vi "PLC_comm.vi"() -> ()   [LabVIEW 2017]
uses:
  <vilib>/addons/database/NI_Database_API.lvlib
  Global/DATA LOG.vi
  Global/Global 1.vi
  <vilib>/DATA AHEAD/SP7/typedefs/PLC Type.ctl
  <vilib>/DATA AHEAD/SP7/SP7.lvlib
  <vilib>/DATA AHEAD/SP7/functions/read/read String.vi
  <vilib>/DATA AHEAD/SP7/functions/write/write Dint array.vi
  <vilib>/DATA AHEAD/SP7/functions/read/read Dint array.vi
  <vilib>/Utility/error.llb/DialogType.ctl
  <vilib>/DATA AHEAD/SP7/functions/read/read real array.vi
  <vilib>/DATA AHEAD/SP7/functions/write/writeString.vi
  84f8396c-11e3-4f6e-927f-d6cb52f8486f.vi
  edb3f7e3-deb4-4efd-b63a-82a20ab466dd.vi
  737c4a97-5810-4f09-bfe1-7e6a970161fd.vi
  98a23aa7-5d76-4ce5-89a1-7ffa2d6e86d6.vi
  065602cd-1ec6-46a4-aff5-3b00a0c776c3.vi
  <vilib>/DATA AHEAD/SP7/typedefs/S7 Connection.ctl
  Control/PLC_Comm_State.ctl
  <vilib>/addons/database/Connection.llb/DB Tools Open Connec (String).vi
  f53d9a16-31ea-4c58-9ec6-4ab155e6634a.vi
  f2e501b8-8033-40fd-b99e-90a89dd29cf5.vi
  a17ecfbb-e8aa-4e6f-9723-a9b27e8c0652.vi
  3deaaee4-0312-4209-8b7c-ccc637c44985.vi
  adc7d8b8-ea76-443b-992e-07ffa118bf03.vi
  cf2a4f70-d875-4391-b4be-4b1ea527ec99.vi
  b767813d-b0bc-4642-82b7-59e8eeaf8486.vi
panel:
  out "error out 4":errorcluster
  out "error out 3":errorcluster
  out "IP1 8":string
  out "PLC 8":bool
  out "IP1 7":string
  out "PLC 7":bool
  out "IP1 6":string
  out "PLC 6":bool
  out "IP1 5":string
  out "PLC 5":bool
  out "PLC 4":bool
  out "PLC 3":bool
  out "PLC 1":bool
  out "IP1 4":string
  out "IP1 3":string
  out "IP1 2":string
  out "IP1":string
  in  "stop":bool
  out "error out":errorcluster
  in  "error in (no error)":errorcluster
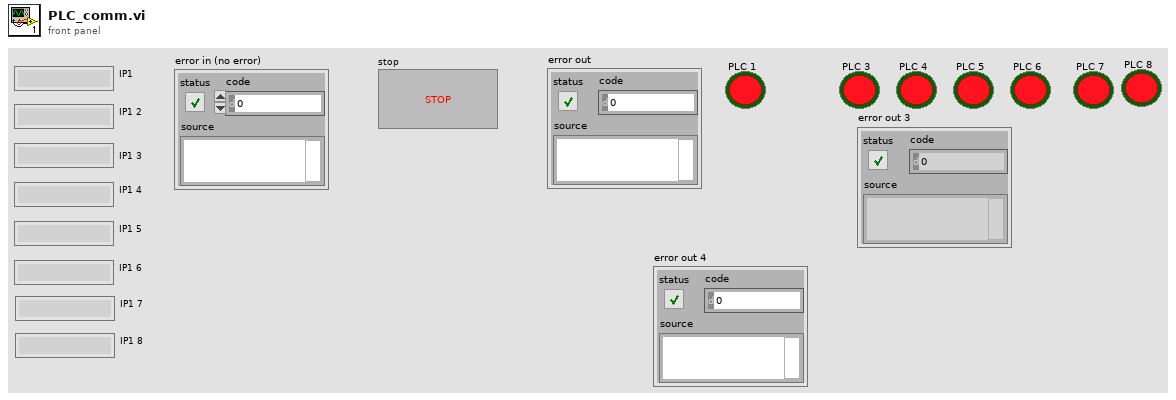
[diagram p1: front panel]
types:
  T1 = typedef "PLC_Comm_State.ctl" = enum16{"Int", "Connect", "Write", "Write2", "Write3", "Read", "Read2", "Read3", "Error", "Disconnect"}
  T2 = typedef "DialogType.ctl" = u16
  T3 = typedef "NI_Database_API.lvlib/Conn ObjectReference.ctl" = refnum<k1>
  T4 = typedef "SP7.lvlib/PLC Type.ctl" = enum16{"S7 200", "S7 300/400", "S7 1200", "S7 1500", "LOGO!8"}
  T5 = typedef "SP7.lvlib/S7 Connection.ctl" = cluster{"TCP Connection Ref":refnum<k5>, "IP address":string, "timeout ms":i32, "Connected?":bool, "PLC Type":T4, "Rack S7 400":u8, "Slot S7 400":u8, "PDU Size":u16, "connection semaphore":T6}
  T6 = typedef "Semaphore RefNum" = refnum<k1>
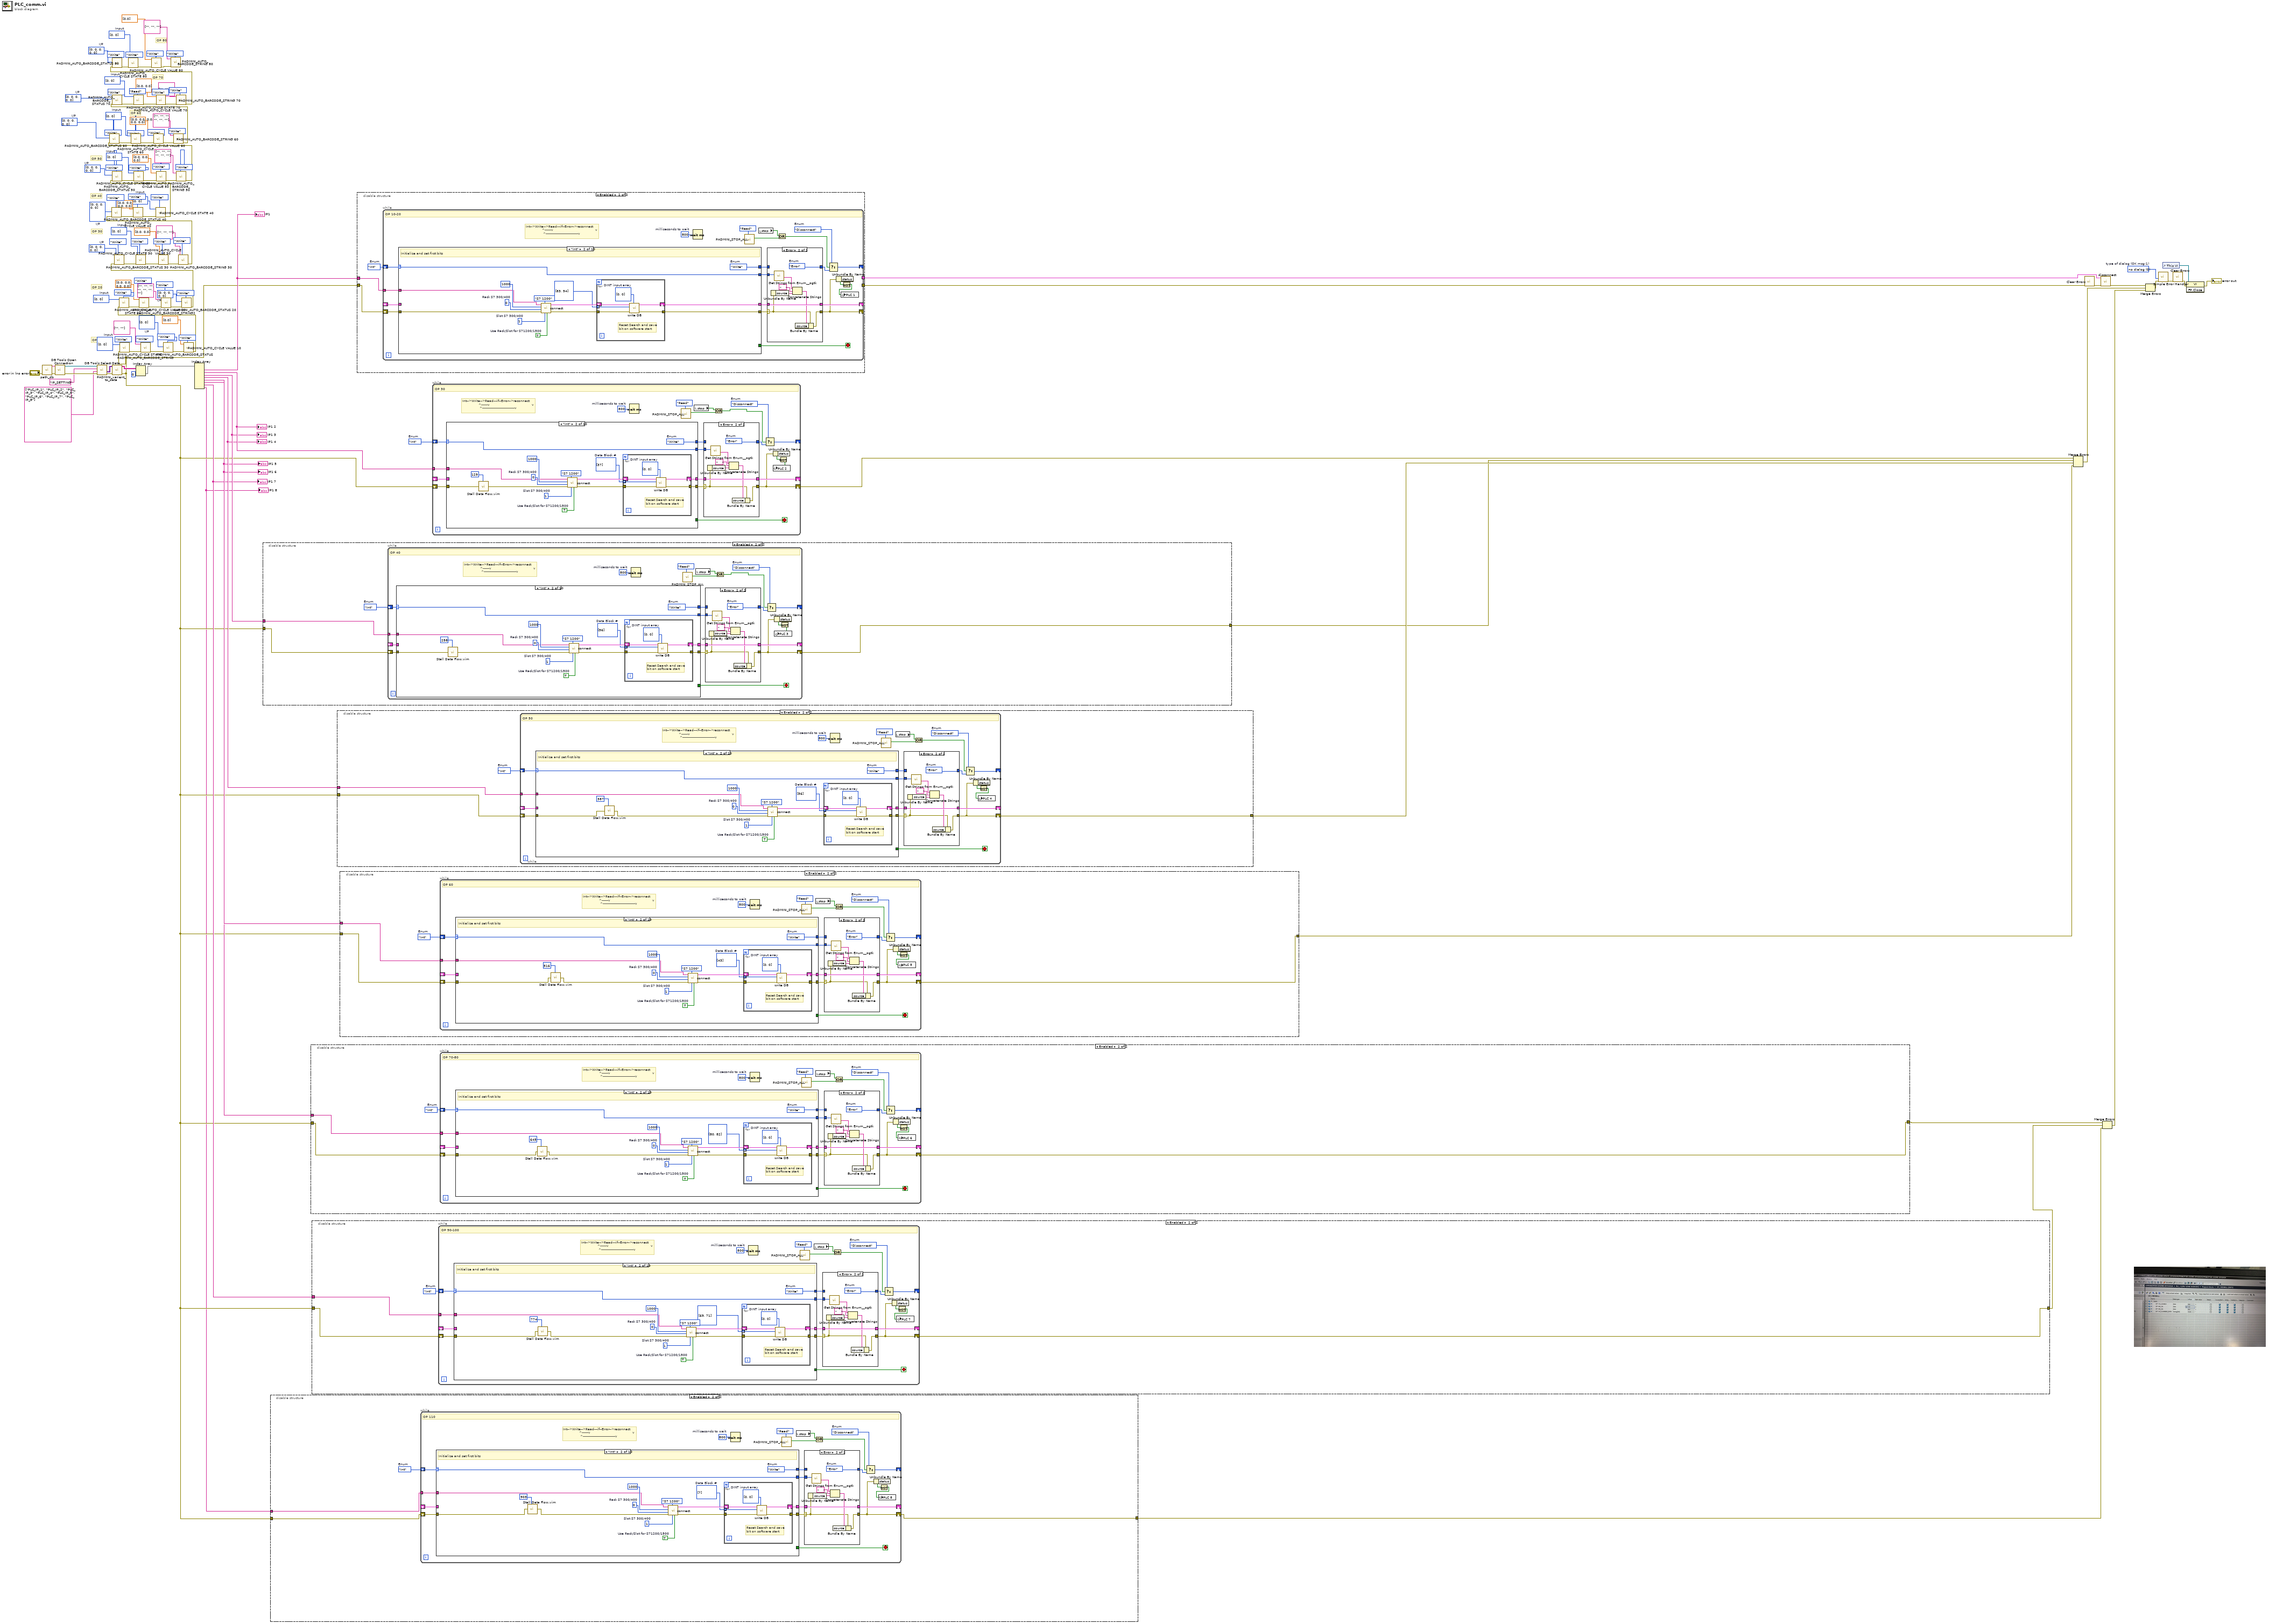
[diagram p0: block diagram]
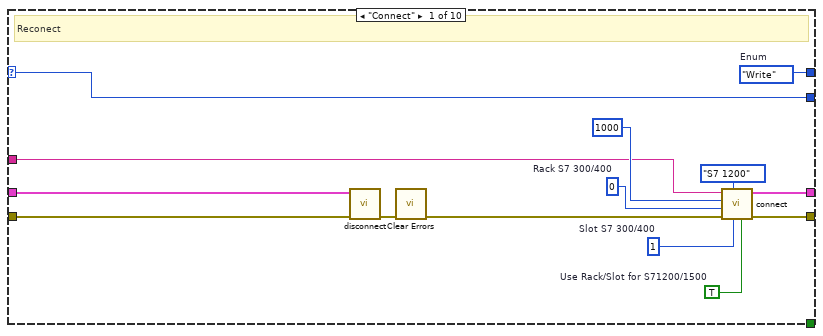
[diagram p3: hidden frame]
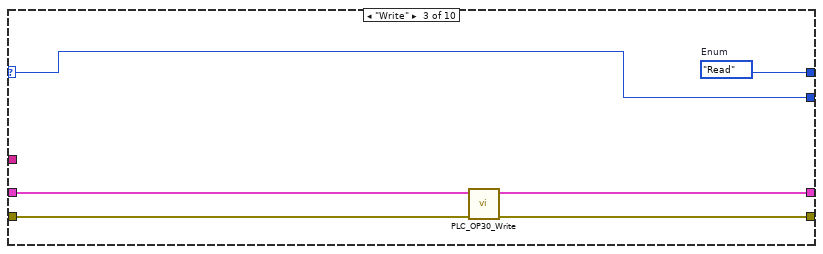
[diagram p4: hidden frame]
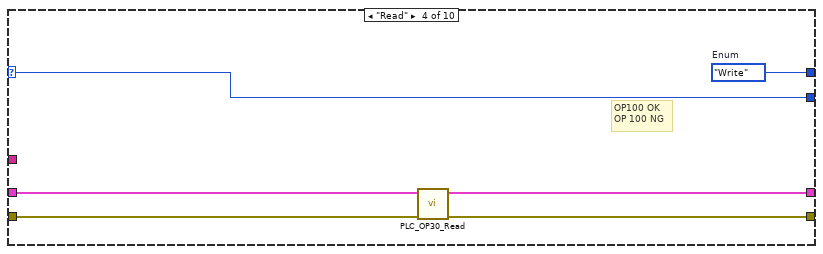
[diagram p5: hidden frame]
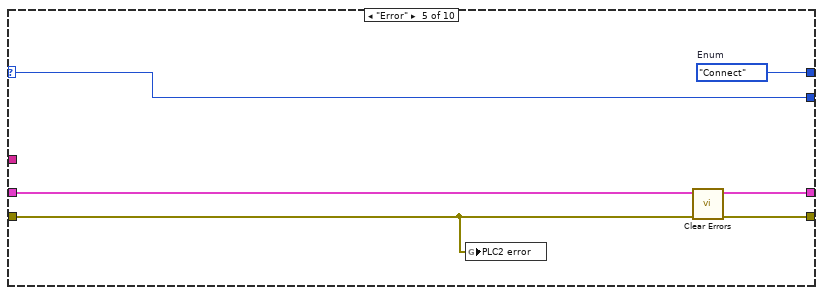
[diagram p6: hidden frame]
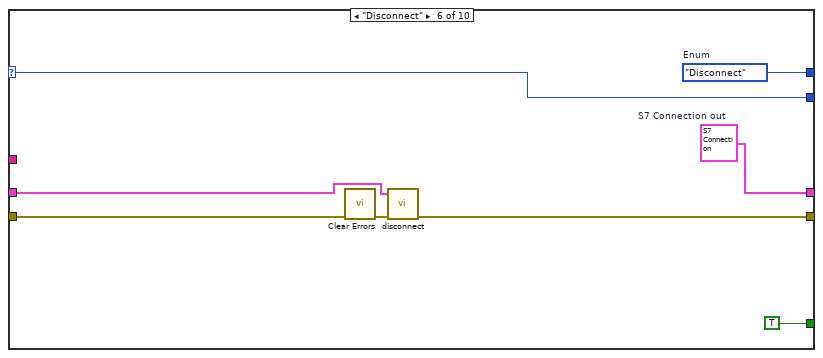
[diagram p7: hidden frame]
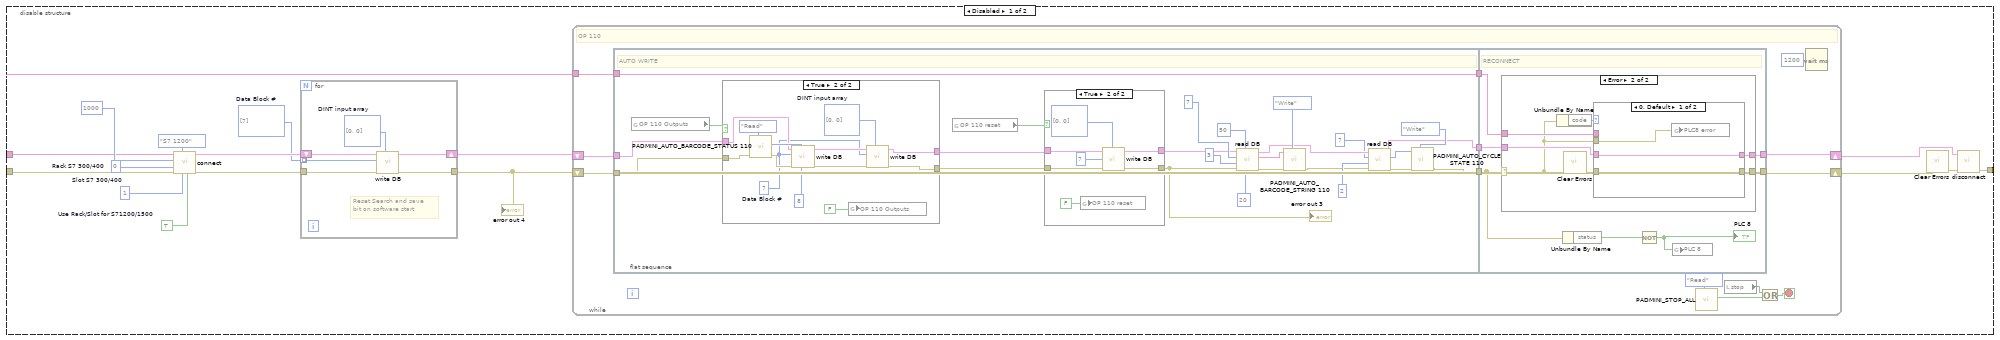
[diagram p12: hidden frame]
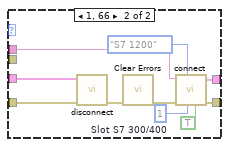
[diagram p16: hidden frame]
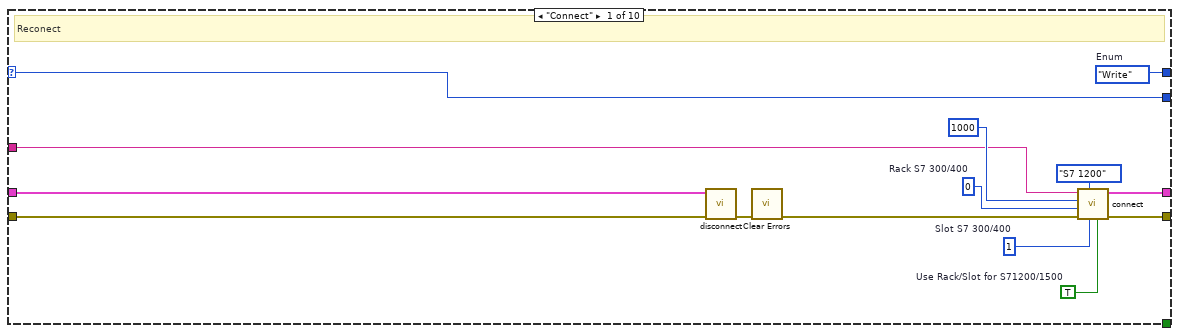
[diagram p18: hidden frame]
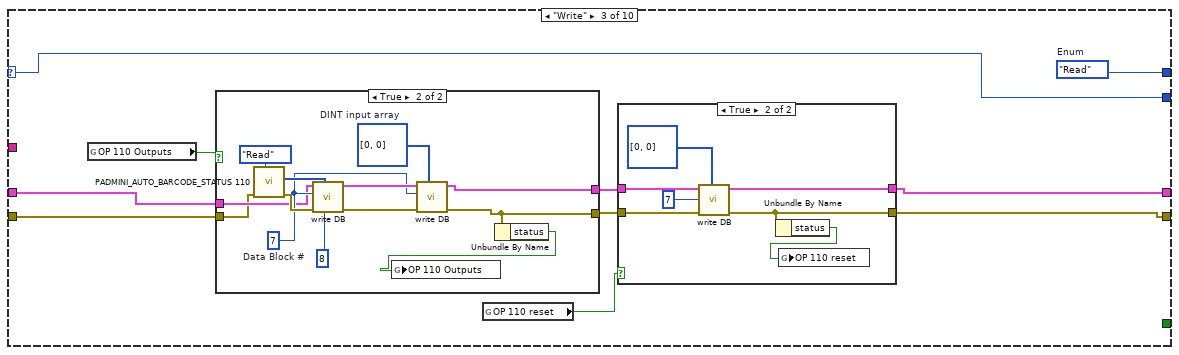
[diagram p19: hidden frame]
diagram:
  w1 = PLC_Comm_State."Int"  # Enum
  w10 = T2 0 items=["no dialog", "OK message", "continue or stop message", "OK message + warnings", "continue/stop + warnings"]  # type of dialog (OK msg:1)
  w12 = i32[] [0, 0, 0, 0, 0]  # I/P
  w13 = i32[] [0, 0]  # Input
  w15 = i32[] [0, 0]  # Input
  w16 = i32[] [0, 0]  # Input
  w18 = i32[] [0, 0]  # Input
  w14 = i32[] [0, 0, 0, 0, 0]  # I/P
  w17 = i32[] [0, 0, 0, 0, 0]  # I/P
  w19 = i32[] [0, 0, 0, 0, 0]  # I/P
  w20 = i32[] [0, 0, 0, 0, 0]  # I/P
  w21 = i32[] [0, 0]  # Input
  w22 = i32[] [0, 0]  # Input
  w23 = i32[] [0, 0, 0, 0, 0]  # I/P
  w24 = i32[] [0, 0, 0, 0, 0]  # I/P
  w25 = i32[] [0, 0]  # Input
  w26 = i32[] [0, 0]  # I/P
  w27 = i32[] [0, 0]  # Input
  # "OP 80"
  # "OP 70"
  # "OP 60"
  # "OP 50"
  # "OP 40"
  # "OP 30"
  # "OP 20"
  # "OP 10"
  n1 = call "path_db.vi"("error in"="error in (no error)") -> ("error out"=w128:errorcluster, "resulting string"=w133:string)  [unwired: 9 in]
  n2 = call-poly <vilib>:"DB Tools Open Connection.vi"("error in (no error)"=w128, "connection information"=w133) -> ("error out"=w132:errorcluster, "connection reference"=w131:T3)  [unwired: 6 in]
  n3 = call <vilib>:"DB Tools Select Data.vi"("error in (no error)"=w132, "columns"=string[] ["PLC_IP_1", "PLC_IP_2", "PLC_IP_3", "PLC_IP_4", "PLC_IP_5", "PLC_IP_6", "PLC_IP_7", "PLC_IP_8"], "table"="IP_SETTING", "connection reference"=w131) -> ("error out"=w130:errorcluster, "data"=w129:variant[][])  [unwired: 2 in, 1 out]
  n4 = call "PADMINI_varient_to_data.vi"("error in (no error)"=w130, "data"=w129) -> ("error out"=w9:errorcluster, "Array"=w124:string[][])  [unwired: 8 in]
  n5 = call "PADMINI_AUTO_CYCLE STATE.vi"("Enum"=enum16{"Read", "Write"}."Write", "error in (no error)"=w9, "Input"=w27) -> ("error out"=w114:errorcluster)  [unwired: 7 in, 1 out]
  n6 = Index Array(array=w124, index (row)=0) -> (element=w123:string[])  [unwired: 1 in]
  n7 = call "PADMINI_AUTO_BARCODE_STRING.vi"("Enum"=enum16{"Read", "Write"}."Write", "error in (no error)"=w114, "Input"=string[] ["", ""]) -> ("error out"=w111:errorcluster)  [unwired: 7 in, 1 out]
  n8 = call "PADMINI_AUTO_BARCODE_STATUS.vi"("Enum"=enum16{"Read", "Write"}."Write", "error in (no error)"=w111, "I/P"=w26) -> ("error out"=w109:errorcluster)  [unwired: 7 in, 1 out]
  n9 = call "PADMINI_AUTO_CYCLE VALUE 10.vi"("Enum"=enum16{"Read", "Write"}."Write", "error in (no error)"=w109, "Input"=dbl[] [0.0]) -> ("error out"=w103:errorcluster)  [unwired: 7 in, 1 out]
  n10 = call "PADMINI_AUTO_CYCLE STATE 20.vi"("Enum"=enum16{"Read", "Write"}."Write", "error in (no error)"=w103, "Input"=w13) -> ("error out"=w101:errorcluster)  [unwired: 7 in, 1 out]
  n11 = call "PADMINI_AUTO_CYCLE VALUE 20.vi"("Enum"=enum16{"Read", "Write"}."Write", "error in (no error)"=w101, "Input"=dbl[] [0.0, 0.0, 0.0, 0.0]) -> ("error out"=w97:errorcluster)  [unwired: 7 in, 1 out]
  n12 = call "PADMINI_AUTO_BARCODE_STRING2.vi"("Enum"=enum16{"Read", "Write"}."Write", "error in (no error)"=w97, "Input"=string[] ["", "", "", "", "", "", ""]) -> ("error out"=w95:errorcluster)  [unwired: 7 in, 1 out]
  n13 = call "PADMINI_AUTO_BARCODE_STATUS 20.vi"("Enum"=enum16{"Read", "Write"}."Write", "error in (no error)"=w95, "I/P"=w12) -> ("error out"=w93:errorcluster)  [unwired: 7 in, 1 out]
  n14 = call "PADMINI_AUTO_BARCODE_STATUS 30.vi"("Enum"=enum16{"Read", "Write"}."Write", "error in (no error)"=w93, "I/P"=w14) -> ("error out"=w90:errorcluster)  [unwired: 7 in, 1 out]
  n15 = call "PADMINI_AUTO_CYCLE STATE 30.vi"("Enum"=enum16{"Read", "Write"}."Write", "error in (no error)"=w90, "Input"=w15) -> ("error out"=w89:errorcluster)  [unwired: 7 in, 1 out]
  n16 = call "PADMINI_AUTO_CYCLE VALUE 30.vi"("Enum"=enum16{"Read", "Write"}."Write", "error in (no error)"=w89, "Input"=dbl[] [0.0, 0.0]) -> ("error out"=w86:errorcluster)  [unwired: 7 in, 1 out]
  n17 = call "PADMINI_AUTO_BARCODE_STRING 30.vi"("Enum"=enum16{"Read", "Write"}."Write", "error in (no error)"=w86, "Input"=string[] ["", "", ""]) -> ("error out"=w76:errorcluster)  [unwired: 7 in, 1 out]
  n18 = call "PADMINI_AUTO_BARCODE_STATUS 40.vi"("Enum"=enum16{"Read", "Write"}."Write", "error in (no error)"=w76, "I/P"=w17) -> ("error out"=w75:errorcluster)  [unwired: 7 in, 1 out]
  n19 = call "PADMINI_AUTO_CYCLE VALUE 40.vi"("Enum"=enum16{"Read", "Write"}."Write", "error in (no error)"=w75, "Input"=dbl[] [0.0, 0.0, 0.0, 0.0]) -> ("error out"=w74:errorcluster)  [unwired: 7 in, 1 out]
  n20 = call "PADMINI_AUTO_CYCLE STATE 40.vi"("Enum"=enum16{"Read", "Write"}."Write", "error in (no error)"=w74, "Input"=w16) -> ("error out"=w73:errorcluster)  [unwired: 7 in, 1 out]
  n21 = call "PADMINI_AUTO_BARCODE_STATUS 50.vi"("Enum"=enum16{"Read", "Write"}."Write", "error in (no error)"=w73, "I/P"=w19) -> ("error out"=w65:errorcluster)  [unwired: 7 in, 1 out]
  n22 = call "PADMINI_AUTO_CYCLE STATE 50.vi"("Enum"=enum16{"Read", "Write"}."Write", "error in (no error)"=w65, "Input"=w18) -> ("error out"=w69:errorcluster)  [unwired: 7 in, 1 out]
  n23 = call "PADMINI_AUTO_CYCLE VALUE 50.vi"("Enum"=enum16{"Read", "Write"}."Write", "error in (no error)"=w69, "Input"=dbl[] [0.0, 0.0, 0.0]) -> ("error out"=w66:errorcluster)  [unwired: 7 in, 1 out]
  n24 = call "PADMINI_AUTO_BARCODE_STRING 50.vi"("Enum"=enum16{"Read", "Write"}."Write", "error in (no error)"=w66, "Input"=string[] ["", "", "", "", "", ""]) -> ("error out"=w51:errorcluster)  [unwired: 7 in, 1 out]
  n25 = call "PADMINI_AUTO_BARCODE_STATUS 60.vi"("Enum"=enum16{"Read", "Write"}."Write", "error in (no error)"=w51, "I/P"=w20) -> ("error out"=w55:errorcluster)  [unwired: 7 in, 1 out]
  n26 = call "PADMINI_AUTO_CYCLE STATE 60.vi"("Enum"=enum16{"Read", "Write"}."Write", "error in (no error)"=w55, "Input"=w21) -> ("error out"=w57:errorcluster)  [unwired: 7 in, 1 out]
  n27 = call "PADMINI_AUTO_CYCLE VALUE 60.vi"("Enum"=enum16{"Read", "Write"}."Write", "error in (no error)"=w57, "Input"=dbl[] [0.0, 0.0, 0.0, 0.0, 0.0]) -> ("error out"=w60:errorcluster)  [unwired: 7 in, 1 out]
  n28 = call "PADMINI_AUTO_BARCODE_STRING 60.vi"("Enum"=enum16{"Read", "Write"}."Write", "error in (no error)"=w60, "Input"=string[] ["", "", "", "", "", ""]) -> ("error out"=w34:errorcluster)  [unwired: 7 in, 1 out]
  n29 = call "PADMINI_AUTO_BARCODE_STATUS 70.vi"("Enum"=enum16{"Read", "Write"}."Write", "error in (no error)"=w34, "I/P"=w23) -> ("error out"=w37:errorcluster)  [unwired: 7 in, 1 out]
  n30 = call "PADMINI_AUTO_CYCLE STATE 70.vi"("Enum"=enum16{"Read", "Write"}."Read", "error in (no error)"=w37, "Input"=w22) -> ("error out"=w49:errorcluster)  [unwired: 7 in, 1 out]
  n31 = call "PADMINI_AUTO_CYCLE VALUE 70.vi"("Enum"=enum16{"Read", "Write"}."Write", "error in (no error)"=w49, "Input"=dbl[] [0.0, 0.0]) -> ("error out"=w46:errorcluster)  [unwired: 7 in, 1 out]
  n32 = call "PADMINI_AUTO_BARCODE_STRING 70.vi"("Enum"=enum16{"Read", "Write"}."Write", "error in (no error)"=w46, "Input"=string[] ["", ""]) -> ("error out"=w31:errorcluster)  [unwired: 7 in, 1 out]
  n33 = call "PADMINI_AUTO_BARCODE_STATUS 80.vi"("Enum"=enum16{"Read", "Write"}."Write", "error in (no error)"=w31, "I/P"=w24) -> ("error out"=w38:errorcluster)  [unwired: 7 in, 1 out]
  n34 = call "PADMINI_AUTO_CYCLE STATE 80.vi"("Enum"=enum16{"Read", "Write"}."Write", "error in (no error)"=w38, "Input"=w25) -> ("error out"=w42:errorcluster)  [unwired: 7 in, 1 out]
  n35 = call "PADMINI_AUTO_CYCLE VALUE 80.vi"("Enum"=enum16{"Read", "Write"}."Write", "error in (no error)"=w42, "Input"=sgl[] [0.0]) -> ("error out"=w45:errorcluster)  [unwired: 7 in, 1 out]
  n36 = call "PADMINI_AUTO_BARCODE_STRING 80.vi"("Enum"=enum16{"Read", "Write"}."Write", "error in (no error)"=w45, "Input"=string[] ["", "", ""]) -> ()  [unwired: 7 in, 2 out]
  n37 = Index Array(array=w123) -> (element #1=w82:string, element #2=w83:string, element #3=w81:string, element #4=w71:string, element #5=w61:string, element #6=w30:string, element #7=w29:string, element #8=w8:string)  [unwired: 8 in]
  "IP1" <- w82
  "IP1 2" <- w83
  "IP1 3" <- w81
  "IP1 4" <- w71
  "IP1 5" <- w61
  "IP1 6" <- w30
  "IP1 7" <- w29
  "IP1 8" <- w8
  n38 = disable-structure shown="Enabled" {
    disable-tunnel: w81 -> [w148 w270]
    disable-tunnel: w9 -> [w139 w269]
    disable-tunnel: [w134 w268] -> w3
    frame Disabled {
      w136 = TRUE  # Use Rack/Slot for S71200/1500
      w137 = u8 0  # Rack S7 300/400
      w138 = u8 1  # Slot S7 300/400
      w144 = i32[] [0, 0]  # DINT input array
      # "Reset Search and save \nbit on software start"
      n39 = call <vilib>:"connect.vi"("Use Rack/Slot for S71200/1500"=w136, "Slot S7 300/400"=w138, "PLC Type"=PLC_Type."S7 1200" ("PLC Type 2"), "error in (no error)"=w139, "Rack S7 300/400"=w137, "timeout [ms]"=1000 ("timeout [ms] 2"), "IP address"=w148) -> ("error out"=w141:errorcluster, "S7 Connection out"=w140:T5)  [unwired: 3 in]
      n40 = call-poly <vilib>:"write DB.vi"("DINT input array"=w144, "error in (no error)"=w141, "Data Block #"=u16 56, "S7 Connection in"=w140) -> ("error out"=w143:errorcluster, "S7 Connection out"=w142:T5)  [unwired: 4 in, 2 out]
      n41 = while {
        shift-right: [w153] -> w146
        shift-left: w142 -> [w163]
        shift-right: [w161] -> w147
        shift-left: w143 -> [w162]
        tunnel: w148 -> [w152]
        stop <- w155 stop-if-true
        # "OP 40"
        n42 = flat-sequence {
          tunnel: [w165] -> w159
          tunnel: [w168] -> w154
          tunnel: w162 -> [w213]
          tunnel: w163 -> [w212]
          tunnel: w152 -> [w200]
          tunnel: [w200] -> w151
          tunnel: [w241] -> w161
          tunnel: [w240] -> w153
          tunnel: w159 -> [w243]
          tunnel: w154 -> [w242]
          tunnel: w151 -> [w239]
          frame #0 {
            w193 = u16 57 ("Data Block #")
            w164 = u16 56 ("Data Block #")
            # "AUTO WRITE"
            n43 = global read "DATA LOG.vi" "OP 40 Outputs"() -> (w211:bool)
            n44 = case shown="True" w211 {
              tunnel: w212 -> [w224 w237]
              tunnel: [w225 w229] -> w198
              tunnel: [w224 w231] -> w199
              tunnel: w213 -> [w225 w234]
              frame False {
              }
              frame True {
                w238 = u16 57  # Data Block #
                n45 = call "PADMINI_AUTO_BARCODE_STATUS 40.vi"("Enum"=enum16{"Read", "Write"}."Read", "error in (no error)"=w234) -> ("error out"=w233:errorcluster, "O/P"=w235:i32[])  [unwired: 8 in]
                n46 = global write "DATA LOG.vi" "OP 40 Outputs"(FALSE) -> ()
                n47 = call-poly <vilib>:"write DB.vi"("DINT input array"=w235, "error in (no error)"=w233, "Data Block #"=w238, "S7 Connection in"=w237) -> ("error out"=w228:errorcluster, "S7 Connection out"=w230:T5)  [unwired: 4 in, 2 out]
                n48 = call-poly <vilib>:"write DB.vi"("DINT input array"=i32[] [0], "error in (no error)"=w228, "Data Block #"=u16 56, "S7 Connection in"=w230) -> ("error out"=w229:errorcluster, "S7 Connection out"=w231:T5)  [unwired: 4 in, 2 out]
              }
            }
            n49 = global read "DATA LOG.vi" "OP 40 reset"() -> (w197:bool)
            n50 = global read "DATA LOG.vi" "Auto Cycle On"() -> (w175:bool)
            n51 = case shown="True" w197 {
              tunnel: w198 -> [w214 w223]
              tunnel: [w214 w222] -> w186
              tunnel: w199 -> [w215 w221]
              tunnel: [w215 w220] -> w187
              frame False {
              }
              frame True {
                n52 = global write "DATA LOG.vi" "OP 40 reset"(FALSE) -> ()
                n53 = call-poly <vilib>:"write DB.vi"("Item offset [byte]"=u16 4 ("Data Block #"), "DINT input array"=i32[] [0], "error in (no error)"=w223, "Data Block #"=u16 56, "S7 Connection in"=w221) -> ("error out"=w222:errorcluster, "S7 Connection out"=w220:T5)  [unwired: 3 in, 2 out]
              }
            }
            n54 = Boolean To (0,1)(Boolean=w175) -> (0, 1=w174:i16)
            n55 = Build Array(w174) -> (w173:i16[])
            n56 = global read "Global 1.vi" "Filtered BARCODE selected"() -> (w196:string[])
            n57 = call-poly <vilib>:"write DB.vi"("Item offset [byte]"=u32 20, "DINT input array"=w173, "error in (no error)"=w186, "Data Block #"=w193, "S7 Connection in"=w187) -> ("error out"=w191:errorcluster, "S7 Connection out"=w190:T5)  [unwired: 3 in, 2 out]
            n58 = call-poly <vilib>:"write DB.vi"("Item offset [byte]"=u32 24, "Input STRINGS"=w196, "error in (no error)"=w191, "String length reserved in DB (default=254)"=u16 15, "Data Block #"=w193, "S7 Connection in"=w190) -> ("error out"=w188:errorcluster, "S7 Connection out"=w189:T5)  [unwired: 2 in, 2 out]
            n59 = call-poly <vilib>:"read DB.vi"("Item offset [byte]"=u32 8, "error in (no error)"=w188, "items #"=u16 4 ("Items # [byte]"), "Data Block #"=w164, "S7 Connection in"=w189) -> ("error out"=w203:errorcluster, "REAL result array"=w201:sgl[], "S7 Connection out"=w209:T5)  [unwired: 4 in]
            n60 = call "PADMINI_AUTO_CYCLE VALUE 40.vi"("Enum"=enum16{"Read", "Write"}."Write", "error in (no error)"=w203, "Input"=w201) -> ("error out"=w202:errorcluster)  [unwired: 7 in, 1 out]
            n61 = call-poly <vilib>:"read DB.vi"("Item offset [byte]"=u32 24, "String length reserved in DB (default=254)"=u16 50, "error in (no error)"=w202, "items #"=u16 1 ("Items # [byte]"), "Data Block #"=w164, "S7 Connection in"=w209) -> ("error out"=w185:errorcluster, "STRING result Array"=w178:string[], "S7 Connection out"=w183:T5)  [unwired: 2 in, 1 out]
            n62 = call-poly <vilib>:"read DB.vi"("Item offset [byte]"=u32 76, "String length reserved in DB (default=254)"=u16 10, "error in (no error)"=w185, "items #"=u16 4 ("Items # [byte]"), "Data Block #"=w164, "S7 Connection in"=w183) -> ("error out"=w184:errorcluster, "STRING result Array"=w177:string[], "S7 Connection out"=w166:T5)  [unwired: 2 in, 1 out]
            n63 = Build Array (concatenate)(w178, w177) -> (w176:string[])
            n64 = call "PADMINI_AUTO_BARCODE_STRING 40.vi"("Enum"=enum16{"Read", "Write"}."Write", "error in (no error)"=w184, "Input"=w176) -> ("error out"=w167:errorcluster)  [unwired: 7 in, 1 out]
            n65 = call-poly <vilib>:"read DB.vi"("error in (no error)"=w167, "items #"=u16 2 ("Items # [byte]"), "Data Block #"=w164, "S7 Connection in"=w166) -> ("error out"=w172:errorcluster, "DINT result array"=w171:i32[], "S7 Connection out"=w165:T5)  [unwired: 5 in]
            n66 = call "PADMINI_AUTO_CYCLE STATE 40.vi"("Enum"=enum16{"Read", "Write"}."Write", "error in (no error)"=w172, "Input"=w171) -> ("error out"=w168:errorcluster)  [unwired: 7 in, 1 out]
          }
          frame #1 {
            # "RECONNECT"
            n67 = case shown="Error" w242 {
              selector: w242 -> [w247 w248]
              tunnel: [w246 w252] -> w240
              tunnel: [w247 w253] -> w241
              tunnel: w243 -> [w246 w251]
              tunnel: w239 -> [_ w250]
              frame No Error {
              }
              frame Error {
                n68 = Unbundle By Name(w248) -> ("code"=w249:i32)
                n69 = call <vilib>:"Clear Errors.vi"("error in (no error)"=w248) -> ("error out"=w254:errorcluster)  [unwired: 5 in, 1 out]
                n70 = case shown="1" w249 {
                  tunnel: w254 -> [w256 w267]
                  tunnel: [w256 w265] -> w253
                  tunnel: [w257 w264] -> w252
                  tunnel: w251 -> [w257 w261]
                  tunnel: w250 -> [_ w260]
                  tunnel: w248 -> [w255 _]
                  frame 0, Default {
                    n71 = global write "Global 1.vi" "PLC3 error"(w255) -> ()
                  }
                  frame 1 {
                    n72 = call <vilib>:"disconnect.vi"("error in (no error)"=w267, "S7 Connection in"=w261) -> ("error out"=w266:errorcluster)  [unwired: 8 in, 1 out]
                    n73 = call <vilib>:"Clear Errors.vi"("error in (no error)"=w266) -> ("error out"=w263:errorcluster)  [unwired: 5 in, 1 out]
                    n74 = call <vilib>:"connect.vi"("Use Rack/Slot for S71200/1500"=TRUE, "Slot S7 300/400"=u8 1, "PLC Type"=PLC_Type."S7 1200" ("PLC Type 2"), "error in (no error)"=w263, "IP address"=w260) -> ("error out"=w265:errorcluster, "S7 Connection out"=w264:T5)  [unwired: 5 in]
                  }
                }
              }
            }
            n75 = Unbundle By Name(w242) -> ("status"=w245:bool)
            n76 = Not(x=w245) -> (.not. x?=w244:bool)
            "PLC 3" <- w244
            n77 = global write "Global 1.vi" "PLC 3"(w244) -> ()
          }
        }
        n78 = call "PADMINI_STOP_ALL.vi"("Enum"=enum16{"Read", "Write"}."Read") -> ("Boolean 2"=w157:bool)  [unwired: 9 in, 1 out]
        n79 = local read "stop"() -> (w156:bool)
        n80 = Or(x=w156, y=w157) -> (x .or. y?=w155:bool)
        n81 = Wait (ms)(milliseconds to wait=u32 1200) -> ()  [unwired: 1 out]
      }
      n82 = call <vilib>:"Clear Errors.vi"("error in (no error)"=w147) -> ("error out"=w135:errorcluster)  [unwired: 5 in, 1 out]
      n83 = call <vilib>:"disconnect.vi"("error in (no error)"=w135, "S7 Connection in"=w146) -> ("error out"=w134:errorcluster)  [unwired: 8 in, 1 out]
    }
    frame Enabled {
      w271 = PLC_Comm_State."Int"  # Enum
      n84 = while {
        shift-right: [w282] -> _
        shift-left: w271 -> [w291]
        shift-right: [w272] -> w268
        shift-left: w269 -> [w290]
        shift-right: [w285] -> _
        shift-left: _ -> [w289]
        tunnel: w270 -> [w288]
        stop <- w283 stop-if-true
        w279 = PLC_Comm_State."Disconnect"  # Enum
        w287 = u32 800  # milliseconds to wait
        # "Int-->Write-->Read---if--Error-->reconnect\n               ^------v                                       v\n                ^------------------------------v"
        # "OP 40"
        n85 = case shown="\"Int\"" w291 {
          selector: w291 -> [w306 w324 w362 w415 w427 w431 _ _ _ _]
          tunnel: [w311 w326 w343 w390 w428 w436 w438 w441 w443 w445] -> w292
          tunnel: [w312 w322 w341 w388 w429 w433 w439 w440 w442 w444] -> w284
          tunnel: w290 -> [w309 w320 w344 w391 w425 w434 w438 w441 w443 w445]
          tunnel: w289 -> [w307 _ w342 w389 w429 w435 w439 w440 w442 w444]
          tunnel: w288 -> [w313 w325 _ _ _ _ _ _ _ _]
          tunnel: [w305 w323 w361 w414 w426 w430 _ _ _ _] -> w286
          tunnel: [_ _ _ _ _ TRUE _ _ _ _] -> w283
          tunnel: [w306 w324 w362 w415 w427 w431 _ _ _ _] -> w280
          frame "Connect" {
            w305 = PLC_Comm_State."Write"  # Enum
            w318 = TRUE  # Use Rack/Slot for S71200/1500
            w317 = u8 1  # Slot S7 300/400
            w315 = u8 0  # Rack S7 300/400
            # "Reconect"
            n86 = call <vilib>:"disconnect.vi"("error in (no error)"=w309, "S7 Connection in"=w307) -> ("error out"=w310:errorcluster)  [unwired: 8 in, 1 out]
            n87 = call <vilib>:"Clear Errors.vi"("error in (no error)"=w310) -> ("error out"=w308:errorcluster)  [unwired: 5 in, 1 out]
            n88 = call <vilib>:"connect.vi"("Use Rack/Slot for S71200/1500"=w318, "Slot S7 300/400"=w317, "PLC Type"=PLC_Type."S7 1200" ("PLC Type 2"), "error in (no error)"=w308, "Rack S7 300/400"=w315, "timeout [ms]"=1000 ("timeout [ms] 2"), "IP address"=w313) -> ("error out"=w311:errorcluster, "S7 Connection out"=w312:T5)  [unwired: 3 in]
          }
          frame "Int" {
            w323 = PLC_Comm_State."Write"  # Enum
            w327 = TRUE  # Use Rack/Slot for S71200/1500
            w328 = u8 1  # Slot S7 300/400
            w329 = u8 0  # Rack S7 300/400
            w330 = u16[] [56]  # Data Block #
            n89 = call "Stall Data Flow.vim"("value in"=w320, "milliseconds to wait"=u32 258) -> ("value out"=w319:errorcluster)  [unwired: 1 out]
            n90 = call <vilib>:"connect.vi"("Use Rack/Slot for S71200/1500"=w327, "Slot S7 300/400"=w328, "PLC Type"=PLC_Type."S7 1200" ("PLC Type 2"), "error in (no error)"=w319, "Rack S7 300/400"=w329, "timeout [ms]"=1000 ("timeout [ms] 2"), "IP address"=w325) -> ("error out"=w332:errorcluster, "S7 Connection out"=w331:T5)  [unwired: 3 in]
            n91 = for {
              tunnel: w330 -> [w340] mode=indexing
              shift-right: [w338] -> w322
              shift-left: w331 -> [w336]
              tunnel: w332 -> [w337]
              tunnel: [w335] -> w326
              w339 = i32[] [0, 0]  # DINT input array
              # "Reset Search and save \nbit on software start"
              n92 = call-poly <vilib>:"write DB.vi"("DINT input array"=w339, "error in (no error)"=w337, "Data Block #"=w340, "S7 Connection in"=w336) -> ("error out"=w335:errorcluster, "S7 Connection out"=w338:T5)  [unwired: 4 in, 2 out]
            }
          }
          frame "Write" {
            w346 = u16 57 ("Data Block #")
            w361 = PLC_Comm_State."Read"  # Enum
            n93 = global read "DATA LOG.vi" "OP 40 Outputs"() -> (w360:bool)
            n94 = case shown="True" w360 {
              tunnel: w342 -> [w373 w375]
              tunnel: [w374 w377] -> w358
              tunnel: [w373 w382] -> w359
              tunnel: w344 -> [w374 w384]
              frame False {
              }
              frame True {
                w387 = u16 57  # Data Block #
                n95 = call "PADMINI_AUTO_BARCODE_STATUS 40.vi"("Enum"=enum16{"Read", "Write"}."Read", "error in (no error)"=w384) -> ("error out"=w383:errorcluster, "O/P"=w385:i32[])  [unwired: 8 in]
                n96 = call-poly <vilib>:"write DB.vi"("DINT input array"=w385, "error in (no error)"=w383, "Data Block #"=w387, "S7 Connection in"=w375) -> ("error out"=w380:errorcluster, "S7 Connection out"=w381:T5)  [unwired: 4 in, 2 out]
                n97 = call-poly <vilib>:"write DB.vi"("DINT input array"=i32[] [0], "error in (no error)"=w380, "Data Block #"=u16 56, "S7 Connection in"=w381) -> ("error out"=w377:errorcluster, "S7 Connection out"=w382:T5)  [unwired: 4 in, 2 out]
                n98 = Unbundle By Name(w377) -> ("status"=w376:bool)
                n99 = global write "DATA LOG.vi" "OP 40 Outputs"(w376) -> ()
              }
            }
            n100 = global read "DATA LOG.vi" "OP 40 reset"() -> (w357:bool)
            n101 = case shown="True" w357 {
              tunnel: w358 -> [w363 w372]
              tunnel: [w363 w367] -> w352
              tunnel: w359 -> [w364 w371]
              tunnel: [w364 w365] -> w353
              frame False {
              }
              frame True {
                n102 = call-poly <vilib>:"write DB.vi"("Item offset [byte]"=u16 4 ("Data Block #"), "DINT input array"=i32[] [0], "error in (no error)"=w372, "Data Block #"=u16 56, "S7 Connection in"=w371) -> ("error out"=w367:errorcluster, "S7 Connection out"=w365:T5)  [unwired: 3 in, 2 out]
                n103 = Unbundle By Name(w367) -> ("status"=w366:bool)
                n104 = global write "DATA LOG.vi" "OP 40 reset"(w366) -> ()
              }
            }
            n105 = global read "Global 1.vi" "Filtered BARCODE selected"() -> (w356:string[])
            n106 = global read "DATA LOG.vi" "Auto Cycle On"() -> (w351:bool)
            n107 = Boolean To (0,1)(Boolean=w351) -> (0, 1=w350:i16)
            n108 = Build Array(w350) -> (w349:i16[])
            n109 = call-poly <vilib>:"write DB.vi"("Item offset [byte]"=u32 20, "DINT input array"=w349, "error in (no error)"=w352, "Data Block #"=w346, "S7 Connection in"=w353) -> ("error out"=w355:errorcluster, "S7 Connection out"=w354:T5)  [unwired: 3 in, 2 out]
            n110 = call-poly <vilib>:"write DB.vi"("Item offset [byte]"=u32 24, "Input STRINGS"=w356, "error in (no error)"=w355, "String length reserved in DB (default=254)"=u16 15, "Data Block #"=w346, "S7 Connection in"=w354) -> ("error out"=w343:errorcluster, "S7 Connection out"=w341:T5)  [unwired: 2 in, 2 out]
          }
          frame "Read" {
            w400 = u16 56 ("Data Block #")
            w414 = PLC_Comm_State."Write"  # Enum
            n111 = call-poly <vilib>:"read DB.vi"("Item offset [byte]"=u32 8, "error in (no error)"=w391, "items #"=u16 4 ("Items # [byte]"), "Data Block #"=w400, "S7 Connection in"=w389) -> ("error out"=w410:errorcluster, "REAL result array"=w413:sgl[], "S7 Connection out"=w411:T5)  [unwired: 4 in]
            n112 = call-poly <vilib>:"read DB.vi"("Item offset [byte]"=u32 24, "String length reserved in DB (default=254)"=u16 50, "error in (no error)"=w410, "items #"=u16 1 ("Items # [byte]"), "Data Block #"=w400, "S7 Connection in"=w411) -> ("error out"=w409:errorcluster, "STRING result Array"=w406:string[], "S7 Connection out"=w407:T5)  [unwired: 2 in, 1 out]
            n113 = call-poly <vilib>:"read DB.vi"("Item offset [byte]"=u32 76, "String length reserved in DB (default=254)"=u16 10, "error in (no error)"=w409, "items #"=u16 4 ("Items # [byte]"), "Data Block #"=w400, "S7 Connection in"=w407) -> ("error out"=w408:errorcluster, "STRING result Array"=w405:string[], "S7 Connection out"=w402:T5)  [unwired: 2 in, 1 out]
            n114 = Build Array (concatenate)(w406, w405) -> (w412:string[])
            n115 = call-poly <vilib>:"read DB.vi"("error in (no error)"=w408, "items #"=u16 2 ("Items # [byte]"), "Data Block #"=w400, "S7 Connection in"=w402) -> ("error out"=w404:errorcluster, "DINT result array"=w403:i32[], "S7 Connection out"=w388:T5)  [unwired: 5 in]
            n116 = case shown="No Error" w404 {
              selector: w404 -> [w419 w424]
              tunnel: w403 -> [w423 _]
              tunnel: w412 -> [w421 _]
              tunnel: w413 -> [w417 _]
              tunnel: [w416 w424] -> w390
              frame No Error {
                w418 = enum16{"Read", "Write"}."Write" ("Enum")
                n117 = call "PADMINI_AUTO_CYCLE VALUE 40.vi"("Enum"=w418, "error in (no error)"=w419, "Input"=w417) -> ("error out"=w420:errorcluster)  [unwired: 7 in, 1 out]
                n118 = call "PADMINI_AUTO_BARCODE_STRING 40.vi"("Enum"=w418, "error in (no error)"=w420, "Input"=w421) -> ("error out"=w422:errorcluster)  [unwired: 7 in, 1 out]
                n119 = call "PADMINI_AUTO_CYCLE STATE 40.vi"("Enum"=w418, "error in (no error)"=w422, "Input"=w423) -> ("error out"=w416:errorcluster)  [unwired: 7 in, 1 out]
              }
              frame Error {
              }
            }
          }
          frame "Error" {
            w426 = PLC_Comm_State."Connect"  # Enum
            n120 = global write "Global 1.vi" "PLC3 error"(w425) -> ()
            n121 = call <vilib>:"Clear Errors.vi"("error in (no error)"=w425) -> ("error out"=w428:errorcluster)  [unwired: 5 in, 1 out]
          }
          frame "Disconnect" {
            w430 = PLC_Comm_State."Disconnect"  # Enum
            w433 = T5 {"TCP Connection Ref"=refnum, "IP address"="", "timeout ms"=5000, "Connected?"=FALSE, "PLC Type"=enum."S7 1200", "Rack S7 400"=0, "Slot S7 400"=0, "PDU Size"=0, "connection semaphore"=refnum}  # S7 Connection out
            n122 = call <vilib>:"Clear Errors.vi"("error in (no error)"=w434) -> ("error out"=w437:errorcluster)  [unwired: 5 in, 1 out]
            n123 = call <vilib>:"disconnect.vi"("error in (no error)"=w437, "S7 Connection in"=w435) -> ("error out"=w436:errorcluster)  [unwired: 8 in, 1 out]
          }
          frame "Write2" {
            # "No Use"
          }
          frame "Write3" {
            # "No Use"
          }
          frame "Read2" {
            # "No Use"
          }
          frame "Read3" {
            # "No Use"
          }
        }
        n124 = Wait (ms)(milliseconds to wait=w287) -> ()  [unwired: 1 out]
        n125 = call "PADMINI_STOP_ALL.vi"("Enum"=enum16{"Read", "Write"}."Read") -> ("Boolean 2"=w278:bool)  [unwired: 9 in, 1 out]
        n126 = local read "stop"() -> (w277:bool)
        n127 = case shown="Error" w292 {
          selector: w292 -> [w295 w298]
          tunnel: [w295 w297] -> w272
          tunnel: [w294 w296] -> w281
          tunnel: w286 -> [w294 _]
          tunnel: [w293 w304] -> w285
          tunnel: w284 -> [w293 w304]
          tunnel: w280 -> [_ w302]
          frame No Error {
          }
          frame Error {
            w296 = PLC_Comm_State."Error"  # Enum
            n128 = Unbundle By Name(w298) -> ("source"=w303:string)
            n129 = call <userlib>:"Get Strings from Enum__ogtk.vi"("Enum"=w302) -> ("String Value"=w301:string)  [unwired: 7 in, 3 out]
            n130 = Concatenate Strings(w301, "    " ("string"), w303) -> (w299:string)
            n131 = Bundle By Name(cluster=w298, "source"=w299) -> (w297:errorcluster)
          }
        }
        n132 = Or(x=w277, y=w278) -> (x .or. y?=w275:bool)
        n133 = Select(t=w279, s=w275, f=w281) -> (s? t:f=w282:T1)
        n134 = Unbundle By Name(w272) -> ("status"=w274:bool)
        n135 = Not(x=w274) -> (.not. x?=w273:bool)
        n136 = global write "Global 1.vi" "PLC 3"(w273) -> ()
      }
    }
  }
  n137 = disable-structure shown="Enabled" {
    disable-tunnel: w9 -> [w455 w560]
    disable-tunnel: w8 -> [w453 w561]
    disable-tunnel: [w449 w559] -> w7
    frame Disabled {
      w446 = TRUE  # Use Rack/Slot for S71200/1500
      w447 = u8 1  # Slot S7 300/400
      w448 = u8 0  # Rack S7 300/400
      w454 = u16[] [7]  # Data Block #
      n138 = call <vilib>:"connect.vi"("Use Rack/Slot for S71200/1500"=w446, "Slot S7 300/400"=w447, "PLC Type"=PLC_Type."S7 1200" ("PLC Type 2"), "error in (no error)"=w455, "Rack S7 300/400"=w448, "timeout [ms]"=1000 ("timeout [ms] 2"), "IP address"=w453) -> ("error out"=w457:errorcluster, "S7 Connection out"=w456:T5)  [unwired: 3 in]
      n139 = for {
        tunnel: w454 -> [w467] mode=indexing
        shift-right: [w465] -> w460
        shift-left: w456 -> [w462]
        tunnel: w457 -> [w463]
        tunnel: [w464] -> w461
        w466 = i32[] [0, 0]  # DINT input array
        # "Reset Search and save \nbit on software start"
        n140 = call-poly <vilib>:"write DB.vi"("DINT input array"=w466, "error in (no error)"=w463, "Data Block #"=w467, "S7 Connection in"=w462) -> ("error out"=w464:errorcluster, "S7 Connection out"=w465:T5)  [unwired: 4 in, 2 out]
      }
      "error out 4" <- w461
      n141 = while {
        shift-right: [w470] -> w450
        shift-left: w460 -> [w480]
        shift-right: [w478] -> w451
        shift-left: w461 -> [w479]
        tunnel: w453 -> [w469]
        stop <- w472 stop-if-true
        # "OP 110"
        n142 = flat-sequence {
          tunnel: [w484] -> w476
          tunnel: [w485] -> w471
          tunnel: w479 -> [w503]
          tunnel: w480 -> [w504]
          tunnel: w469 -> [w505]
          tunnel: [w505] -> w468
          tunnel: [w532] -> w478
          tunnel: [w531] -> w470
          tunnel: w476 -> [w534]
          tunnel: w471 -> [w533]
          tunnel: w468 -> [w530]
          frame #0 {
            # "AUTO WRITE"
            n143 = global read "DATA LOG.vi" "OP 110 Outputs"() -> (w502:bool)
            n144 = case shown="True" w502 {
              tunnel: [w515 w520] -> w494
              tunnel: [w516 w521] -> w493
              tunnel: w503 -> [w515 w525]
              tunnel: w504 -> [w516 w524]
              frame False {
              }
              frame True {
                w517 = i32[] [0, 0]  # DINT input array
                w518 = u16 7  # Data Block #
                n145 = call "PADMINI_AUTO_BARCODE_STATUS 110.vi"("Enum"=enum16{"Read", "Write"}."Read", "error in (no error)"=w525) -> ("error out"=w527:errorcluster, "O/P"=w528:i32[])  [unwired: 8 in]
                n146 = call-poly <vilib>:"write DB.vi"("Item offset [byte]"=u32 8, "DINT input array"=w528, "error in (no error)"=w527, "Data Block #"=w518, "S7 Connection in"=w524) -> ("error out"=w519:errorcluster, "S7 Connection out"=w522:T5)  [unwired: 3 in, 2 out]
                n147 = global write "DATA LOG.vi" "OP 110 Outputs"(FALSE) -> ()
                n148 = call-poly <vilib>:"write DB.vi"("DINT input array"=w517, "error in (no error)"=w519, "Data Block #"=w518, "S7 Connection in"=w522) -> ("error out"=w520:errorcluster, "S7 Connection out"=w521:T5)  [unwired: 4 in, 2 out]
              }
            }
            n149 = global read "DATA LOG.vi" "OP 110 reset"() -> (w491:bool)
            n150 = case shown="True" w491 {
              tunnel: w494 -> [w506 w514]
              tunnel: [w506 w513] -> w495
              tunnel: w493 -> [w507 w512]
              tunnel: [w507 w511] -> w492
              frame False {
              }
              frame True {
                n151 = global write "DATA LOG.vi" "OP 110 reset"(FALSE) -> ()
                n152 = call-poly <vilib>:"write DB.vi"("DINT input array"=i32[] [0, 0], "error in (no error)"=w514, "Data Block #"=u16 7, "S7 Connection in"=w512) -> ("error out"=w513:errorcluster, "S7 Connection out"=w511:T5)  [unwired: 4 in, 2 out]
              }
            }
            "error out 3" <- w495
            n153 = call-poly <vilib>:"read DB.vi"("Item offset [byte]"=u32 20, "String length reserved in DB (default=254)"=u16 50, "error in (no error)"=w495, "items #"=u16 3 ("Items # [byte]"), "Data Block #"=u16 7, "S7 Connection in"=w492) -> ("error out"=w497:errorcluster, "STRING result Array"=w498:string[], "S7 Connection out"=w483:T5)  [unwired: 2 in, 1 out]
            n154 = call "PADMINI_AUTO_BARCODE_STRING 110.vi"("Enum"=enum16{"Read", "Write"}."Write", "error in (no error)"=w497, "Input"=w498) -> ("error out"=w486:errorcluster)  [unwired: 7 in, 1 out]
            n155 = call-poly <vilib>:"read DB.vi"("error in (no error)"=w486, "items #"=u16 2 ("Items # [byte]"), "Data Block #"=u16 7, "S7 Connection in"=w483) -> ("error out"=w490:errorcluster, "DINT result array"=w489:i32[], "S7 Connection out"=w484:T5)  [unwired: 5 in]
            n156 = call "PADMINI_AUTO_CYCLE STATE 110.vi"("Enum"=enum16{"Read", "Write"}."Write", "error in (no error)"=w490, "Input"=w489) -> ("error out"=w485:errorcluster)  [unwired: 7 in, 1 out]
          }
          frame #1 {
            # "RECONNECT"
            n157 = case shown="Error" w533 {
              selector: w533 -> [w538 w539]
              tunnel: [w537 w543] -> w531
              tunnel: [w538 w544] -> w532
              tunnel: w534 -> [w537 w542]
              tunnel: w530 -> [_ w541]
              frame No Error {
              }
              frame Error {
                n158 = Unbundle By Name(w539) -> ("code"=w540:i32)
                n159 = call <vilib>:"Clear Errors.vi"("error in (no error)"=w539) -> ("error out"=w545:errorcluster)  [unwired: 5 in, 1 out]
                n160 = case shown="0, Default" w540 {
                  tunnel: w545 -> [w547 w558]
                  tunnel: [w547 w556] -> w544
                  tunnel: [w548 w555] -> w543
                  tunnel: w542 -> [w548 w552]
                  tunnel: w541 -> [_ w551]
                  tunnel: w539 -> [w546 _]
                  frame 0, Default {
                    n161 = global write "Global 1.vi" "PLC8 error"(w546) -> ()
                  }
                  frame 1, 66 {
                    w550 = u8 1  # Slot S7 300/400
                    n162 = call <vilib>:"disconnect.vi"("error in (no error)"=w558, "S7 Connection in"=w552) -> ("error out"=w557:errorcluster)  [unwired: 8 in, 1 out]
                    n163 = call <vilib>:"Clear Errors.vi"("error in (no error)"=w557) -> ("error out"=w554:errorcluster)  [unwired: 5 in, 1 out]
                    n164 = call <vilib>:"connect.vi"("Use Rack/Slot for S71200/1500"=TRUE, "Slot S7 300/400"=w550, "PLC Type"=PLC_Type."S7 1200" ("PLC Type 2"), "error in (no error)"=w554, "IP address"=w551) -> ("error out"=w556:errorcluster, "S7 Connection out"=w555:T5)  [unwired: 5 in]
                  }
                }
              }
            }
            n165 = Unbundle By Name(w533) -> ("status"=w536:bool)
            n166 = Not(x=w536) -> (.not. x?=w535:bool)
            "PLC 8" <- w535
            n167 = global write "Global 1.vi" "PLC 8"(w535) -> ()
          }
        }
        n168 = call "PADMINI_STOP_ALL.vi"("Enum"=enum16{"Read", "Write"}."Read") -> ("Boolean 2"=w474:bool)  [unwired: 9 in, 1 out]
        n169 = local read "stop"() -> (w473:bool)
        n170 = Or(x=w473, y=w474) -> (x .or. y?=w472:bool)
        n171 = Wait (ms)(milliseconds to wait=u32 1200) -> ()  [unwired: 1 out]
      }
      n172 = call <vilib>:"Clear Errors.vi"("error in (no error)"=w451) -> ("error out"=w452:errorcluster)  [unwired: 5 in, 1 out]
      n173 = call <vilib>:"disconnect.vi"("error in (no error)"=w452, "S7 Connection in"=w450) -> ("error out"=w449:errorcluster)  [unwired: 8 in, 1 out]
    }
    frame Enabled {
      w562 = PLC_Comm_State."Int"  # Enum
      n174 = while {
        shift-right: [w574] -> _
        shift-left: w562 -> [w582]
        shift-right: [w566] -> w559
        shift-left: w560 -> [w581]
        shift-right: [w577] -> _
        shift-left: _ -> [w580]
        tunnel: w561 -> [w563]
        stop <- w575 stop-if-true
        w571 = PLC_Comm_State."Disconnect"  # Enum
        w579 = u32 800  # milliseconds to wait
        # "Int-->Write-->Read---if--Error-->reconnect\n               ^------v                                       v\n                ^------------------------------v"
        # "OP 110"
        n175 = case shown="\"Int\"" w582 {
          selector: w582 -> [w598 w615 w641 w682 w692 w696 _ _ _ _]
          tunnel: [w603 w617 w634 w668 w693 w701 w703 w706 w708 w710] -> w583
          tunnel: [w604 w616 w635 w669 w694 w698 w704 w705 w707 w709] -> w576
          tunnel: w581 -> [w601 w611 w632 w666 w690 w699 w703 w706 w708 w710]
          tunnel: w580 -> [w599 _ w633 w667 w694 w700 w704 w705 w707 w709]
          tunnel: [w597 w614 w640 w681 w691 w695 _ _ _ _] -> w578
          tunnel: [_ _ _ _ _ TRUE _ _ _ _] -> w575
          tunnel: [w598 w615 w641 w682 w692 w696 _ _ _ _] -> w572
          tunnel: w563 -> [w596 w613 _ _ _ _ _ _ _ _]
          frame "Connect" {
            w597 = PLC_Comm_State."Write"  # Enum
            w609 = TRUE  # Use Rack/Slot for S71200/1500
            w608 = u8 1  # Slot S7 300/400
            w606 = u8 0  # Rack S7 300/400
            # "Reconect"
            n176 = call <vilib>:"disconnect.vi"("error in (no error)"=w601, "S7 Connection in"=w599) -> ("error out"=w602:errorcluster)  [unwired: 8 in, 1 out]
            n177 = call <vilib>:"Clear Errors.vi"("error in (no error)"=w602) -> ("error out"=w600:errorcluster)  [unwired: 5 in, 1 out]
            n178 = call <vilib>:"connect.vi"("Use Rack/Slot for S71200/1500"=w609, "Slot S7 300/400"=w608, "PLC Type"=PLC_Type."S7 1200" ("PLC Type 2"), "error in (no error)"=w600, "Rack S7 300/400"=w606, "timeout [ms]"=1000 ("timeout [ms] 2"), "IP address"=w596) -> ("error out"=w603:errorcluster, "S7 Connection out"=w604:T5)  [unwired: 3 in]
          }
          frame "Int" {
            w614 = PLC_Comm_State."Write"  # Enum
            w618 = TRUE  # Use Rack/Slot for S71200/1500
            w619 = u8 1  # Slot S7 300/400
            w620 = u8 0  # Rack S7 300/400
            w621 = u16[] [7]  # Data Block #
            # "Initialize and set first bits"
            n179 = call "Stall Data Flow.vim"("value in"=w611, "milliseconds to wait"=u32 903) -> ("value out"=w610:errorcluster)  [unwired: 1 out]
            n180 = call <vilib>:"connect.vi"("Use Rack/Slot for S71200/1500"=w618, "Slot S7 300/400"=w619, "PLC Type"=PLC_Type."S7 1200" ("PLC Type 2"), "error in (no error)"=w610, "Rack S7 300/400"=w620, "timeout [ms]"=1000 ("timeout [ms] 2"), "IP address"=w613) -> ("error out"=w623:errorcluster, "S7 Connection out"=w622:T5)  [unwired: 3 in]
            n181 = for {
              tunnel: w621 -> [w631] mode=indexing
              shift-right: [w629] -> w616
              shift-left: w622 -> [w627]
              tunnel: w623 -> [w628]
              tunnel: [w626] -> w617
              w630 = i32[] [0, 0]  # DINT input array
              # "Reset Search and save \nbit on software start"
              n182 = call-poly <vilib>:"write DB.vi"("DINT input array"=w630, "error in (no error)"=w628, "Data Block #"=w631, "S7 Connection in"=w627) -> ("error out"=w626:errorcluster, "S7 Connection out"=w629:T5)  [unwired: 4 in, 2 out]
            }
          }
          frame "Write" {
            w640 = PLC_Comm_State."Read"  # Enum
            n183 = global read "DATA LOG.vi" "OP 110 Outputs"() -> (w639:bool)
            n184 = case shown="True" w639 {
              tunnel: [w651 w656] -> w638
              tunnel: [w652 w660] -> w637
              tunnel: w633 -> [w652 w654]
              tunnel: w632 -> [w651 w653]
              frame False {
              }
              frame True {
                w657 = i32[] [0, 0]  # DINT input array
                w658 = u16 7  # Data Block #
                n185 = call "PADMINI_AUTO_BARCODE_STATUS 110.vi"("Enum"=enum16{"Read", "Write"}."Read", "error in (no error)"=w653) -> ("error out"=w663:errorcluster, "O/P"=w664:i32[])  [unwired: 8 in]
                n186 = call-poly <vilib>:"write DB.vi"("Item offset [byte]"=u32 8, "DINT input array"=w664, "error in (no error)"=w663, "Data Block #"=w658, "S7 Connection in"=w654) -> ("error out"=w659:errorcluster, "S7 Connection out"=w661:T5)  [unwired: 3 in, 2 out]
                n187 = call-poly <vilib>:"write DB.vi"("DINT input array"=w657, "error in (no error)"=w659, "Data Block #"=w658, "S7 Connection in"=w661) -> ("error out"=w656:errorcluster, "S7 Connection out"=w660:T5)  [unwired: 4 in, 2 out]
                n188 = Unbundle By Name(w656) -> ("status"=w655:bool)
                n189 = global write "DATA LOG.vi" "OP 110 Outputs"(w655) -> ()
              }
            }
            n190 = global read "DATA LOG.vi" "OP 110 reset"() -> (w636:bool)
            n191 = case shown="True" w636 {
              tunnel: w638 -> [w642 w650]
              tunnel: [w642 w645] -> w634
              tunnel: w637 -> [w643 w649]
              tunnel: [w643 w648] -> w635
              frame False {
              }
              frame True {
                n192 = call-poly <vilib>:"write DB.vi"("DINT input array"=i32[] [0, 0], "error in (no error)"=w650, "Data Block #"=u16 7, "S7 Connection in"=w649) -> ("error out"=w645:errorcluster, "S7 Connection out"=w648:T5)  [unwired: 4 in, 2 out]
                n193 = Unbundle By Name(w645) -> ("status"=w644:bool)
                n194 = global write "DATA LOG.vi" "OP 110 reset"(w644) -> ()
              }
            }
          }
          frame "Read" {
            w681 = PLC_Comm_State."Write"  # Enum
            n195 = call-poly <vilib>:"read DB.vi"("Item offset [byte]"=u32 20, "String length reserved in DB (default=254)"=u16 50, "error in (no error)"=w666, "items #"=u16 3 ("Items # [byte]"), "Data Block #"=u16 7, "S7 Connection in"=w667) -> ("error out"=w679:errorcluster, "STRING result Array"=w680:string[], "S7 Connection out"=w676:T5)  [unwired: 2 in, 1 out]
            n196 = call-poly <vilib>:"read DB.vi"("error in (no error)"=w679, "items #"=u16 2 ("Items # [byte]"), "Data Block #"=u16 7, "S7 Connection in"=w676) -> ("error out"=w678:errorcluster, "DINT result array"=w677:i32[], "S7 Connection out"=w669:T5)  [unwired: 5 in]
            n197 = case shown="Error" w678 {
              selector: w678 -> [w687 w689]
              tunnel: w677 -> [w688 _]
              tunnel: w680 -> [w684 _]
              tunnel: [w683 w689] -> w668
              frame No Error {
                w685 = enum16{"Read", "Write"}."Write" ("Enum")
                n198 = call "PADMINI_AUTO_BARCODE_STRING 110.vi"("Enum"=w685, "error in (no error)"=w687, "Input"=w684) -> ("error out"=w686:errorcluster)  [unwired: 7 in, 1 out]
                n199 = call "PADMINI_AUTO_CYCLE STATE 110.vi"("Enum"=w685, "error in (no error)"=w686, "Input"=w688) -> ("error out"=w683:errorcluster)  [unwired: 7 in, 1 out]
              }
              frame Error {
              }
            }
          }
          frame "Error" {
            w691 = PLC_Comm_State."Connect"  # Enum
            n200 = global write "Global 1.vi" "PLC8 error"(w690) -> ()
            n201 = call <vilib>:"Clear Errors.vi"("error in (no error)"=w690) -> ("error out"=w693:errorcluster)  [unwired: 5 in, 1 out]
          }
          frame "Disconnect" {
            w695 = PLC_Comm_State."Disconnect"  # Enum
            w698 = T5 {"TCP Connection Ref"=refnum, "IP address"="", "timeout ms"=5000, "Connected?"=FALSE, "PLC Type"=enum."S7 1200", "Rack S7 400"=0, "Slot S7 400"=0, "PDU Size"=0, "connection semaphore"=refnum}  # S7 Connection out
            n202 = call <vilib>:"Clear Errors.vi"("error in (no error)"=w699) -> ("error out"=w702:errorcluster)  [unwired: 5 in, 1 out]
            n203 = call <vilib>:"disconnect.vi"("error in (no error)"=w702, "S7 Connection in"=w700) -> ("error out"=w701:errorcluster)  [unwired: 8 in, 1 out]
          }
          frame "Write2" {
            # "No Use"
          }
          frame "Write3" {
            # "No Use"
          }
          frame "Read2" {
            # "No Use"
          }
          frame "Read3" {
            # "No Use"
          }
        }
        n204 = Wait (ms)(milliseconds to wait=w579) -> ()  [unwired: 1 out]
        n205 = call "PADMINI_STOP_ALL.vi"("Enum"=enum16{"Read", "Write"}."Read") -> ("Boolean 2"=w570:bool)  [unwired: 9 in, 1 out]
        n206 = local read "stop"() -> (w565:bool)
        n207 = case shown="Error" w583 {
          selector: w583 -> [w586 w589]
          tunnel: [w586 w588] -> w566
          tunnel: [w585 w587] -> w573
          tunnel: w578 -> [w585 _]
          tunnel: [w584 w595] -> w577
          tunnel: w576 -> [w584 w595]
          tunnel: w572 -> [_ w593]
          frame No Error {
          }
          frame Error {
            w587 = PLC_Comm_State."Error"  # Enum
            n208 = Unbundle By Name(w589) -> ("source"=w594:string)
            n209 = call <userlib>:"Get Strings from Enum__ogtk.vi"("Enum"=w593) -> ("String Value"=w592:string)  [unwired: 7 in, 3 out]
            n210 = Concatenate Strings(w592, "    " ("string"), w594) -> (w590:string)
            n211 = Bundle By Name(cluster=w589, "source"=w590) -> (w588:errorcluster)
          }
        }
        n212 = Or(x=w565, y=w570) -> (x .or. y?=w568:bool)
        n213 = Select(t=w571, s=w568, f=w573) -> (s? t:f=w574:T1)
        n214 = Unbundle By Name(w566) -> ("status"=w567:bool)
        n215 = Not(x=w567) -> (.not. x?=w564:bool)
        n216 = global write "Global 1.vi" "PLC 8"(w564) -> ()
      }
    }
  }
  n217 = disable-structure shown="Enabled" {
    disable-tunnel: w30 -> [w722 w936]
    disable-tunnel: w9 -> [w716 w935]
    disable-tunnel: [w711 w933] -> w5
    frame Disabled {
      w713 = TRUE  # Use Rack/Slot for S71200/1500
      w714 = u8 1  # Slot S7 300/400
      w715 = u8 0  # Rack S7 300/400
      n218 = call <vilib>:"connect.vi"("Use Rack/Slot for S71200/1500"=w713, "Slot S7 300/400"=w714, "PLC Type"=PLC_Type."S7 1200" ("PLC Type 2"), "error in (no error)"=w716, "Rack S7 300/400"=w715, "timeout [ms]"=1000 ("timeout [ms] 2"), "IP address"=w722) -> ("error out"=w717:errorcluster, "S7 Connection out"=w718:T5)  [unwired: 3 in]
      n219 = for {
        tunnel: u16[] [80, 82] ("Data Block #") -> [w732] mode=indexing
        shift-right: [w730] -> w719
        shift-left: w718 -> [w727]
        tunnel: w717 -> [w728]
        tunnel: [w729] -> w720
        w731 = i32[] [0, 0]  # DINT input array
        # "Reset Search and save \nbit on software start"
        n220 = call-poly <vilib>:"write DB.vi"("DINT input array"=w731, "error in (no error)"=w728, "Data Block #"=w732, "S7 Connection in"=w727) -> ("error out"=w729:errorcluster, "S7 Connection out"=w730:T5)  [unwired: 4 in, 2 out]
      }
      n221 = while {
        shift-right: [w735] -> w723
        shift-left: w719 -> [w745]
        shift-right: [w743] -> w724
        shift-left: w720 -> [w744]
        tunnel: w722 -> [w734]
        stop <- w737 stop-if-true
        # "OP 70 - 80"
        n222 = flat-sequence {
          tunnel: [w747] -> w741
          tunnel: [w751] -> w736
          tunnel: w744 -> [w853]
          tunnel: w745 -> [w852]
          tunnel: w734 -> [w840]
          tunnel: [w840] -> w733
          tunnel: [w906] -> w743
          tunnel: [w905] -> w735
          tunnel: w741 -> [w908]
          tunnel: w736 -> [w907]
          tunnel: w733 -> [w904]
          frame #0 {
            w772 = u32 500  # milliseconds to wait
            w799 = u16 83 ("Data Block #")
            w822 = u16 81 ("Data Block #")
            w783 = u16 82 ("Data Block #")
            w759 = u16 80 ("Data Block #")
            # "AUTO WRITE"
            n223 = global read "DATA LOG.vi" "OP 70 Outputs"() -> (w851:bool)
            n224 = case shown="True" w851 {
              tunnel: w852 -> [w889 w902]
              tunnel: [w890 w893] -> w827
              tunnel: [w889 w894] -> w826
              tunnel: w853 -> [w890 w899]
              frame False {
              }
              frame True {
                w903 = u16 81  # Data Block #
                n225 = call "PADMINI_AUTO_BARCODE_STATUS 70.vi"("Enum"=enum16{"Read", "Write"}."Read", "error in (no error)"=w899) -> ("error out"=w898:errorcluster, "O/P"=w900:i32[])  [unwired: 8 in]
                n226 = global write "DATA LOG.vi" "OP 70 Outputs"(FALSE) -> ()
                n227 = call-poly <vilib>:"write DB.vi"("DINT input array"=w900, "error in (no error)"=w898, "Data Block #"=w903, "S7 Connection in"=w902) -> ("error out"=w891:errorcluster, "S7 Connection out"=w892:T5)  [unwired: 4 in, 2 out]
                n228 = call-poly <vilib>:"write DB.vi"("DINT input array"=i32[] [0] ("Data Byte"), "error in (no error)"=w891, "Data Block #"=u16 80, "S7 Connection in"=w892) -> ("error out"=w893:errorcluster, "S7 Connection out"=w894:T5)  [unwired: 4 in, 2 out]
              }
            }
            n229 = global read "DATA LOG.vi" "OP 70 reset"() -> (w828:bool)
            n230 = global read "DATA LOG.vi" "Auto Cycle On"() -> (w776:bool)
            n231 = case shown="True" w828 {
              tunnel: w827 -> [w864 w873]
              tunnel: [w864 w872] -> w817
              tunnel: w826 -> [w865 w871]
              tunnel: [w865 w870] -> w818
              frame False {
              }
              frame True {
                n232 = global write "DATA LOG.vi" "OP 70 reset"(FALSE) -> ()
                n233 = call-poly <vilib>:"write DB.vi"("Item offset [byte]"=u16 4 ("Data Block #"), "DINT input array"=i32[] [0], "error in (no error)"=w873, "Data Block #"=u16 80, "S7 Connection in"=w871) -> ("error out"=w872:errorcluster, "S7 Connection out"=w870:T5)  [unwired: 3 in, 2 out]
              }
            }
            n234 = Boolean To (0,1)(Boolean=w776) -> (0, 1=w775:i16)
            n235 = Build Array(w775) -> (w774:i16[])
            n236 = call "Stall Data Flow.vim"("value in"=w817, "milliseconds to wait"=w772) -> ("value out"=w773:errorcluster)  [unwired: 1 out]
            n237 = global read "Global 1.vi" "Filtered BARCODE selected"() -> (w819:string[])
            n238 = call-poly <vilib>:"write DB.vi"("Item offset [byte]"=u32 20, "DINT input array"=w774, "error in (no error)"=w773, "Data Block #"=w822, "S7 Connection in"=w818) -> ("error out"=w824:errorcluster, "S7 Connection out"=w825:T5)  [unwired: 3 in, 2 out]
            n239 = call-poly <vilib>:"write DB.vi"("Item offset [byte]"=u32 24, "Input STRINGS"=w819, "error in (no error)"=w824, "String length reserved in DB (default=254)"=u16 15, "Data Block #"=w822, "S7 Connection in"=w825) -> ("error out"=w815:errorcluster, "S7 Connection out"=w816:T5)  [unwired: 2 in, 2 out]
            n240 = call "Stall Data Flow.vim"("value in"=w815, "milliseconds to wait"=u32 300) -> ("value out"=w771:errorcluster)  [unwired: 1 out]
            n241 = call-poly <vilib>:"read DB.vi"("Item offset [byte]"=u32 8, "error in (no error)"=w771, "items #"=u16 2 ("Items # [byte]"), "Data Block #"=w759, "S7 Connection in"=w816) -> ("error out"=w843:errorcluster, "REAL result array"=w841:sgl[], "S7 Connection out"=w849:T5)  [unwired: 4 in]
            n242 = call "PADMINI_AUTO_CYCLE VALUE 70.vi"("Enum"=enum16{"Read", "Write"}."Write", "error in (no error)"=w843, "Input"=w841) -> ("error out"=w842:errorcluster)  [unwired: 7 in, 1 out]
            n243 = call "Stall Data Flow.vim"("value in"=w842, "milliseconds to wait"=u32 0) -> ("value out"=w769:errorcluster)  [unwired: 1 out]
            n244 = call-poly <vilib>:"read DB.vi"("Item offset [byte]"=u32 16, "String length reserved in DB (default=254)"=u16 50, "error in (no error)"=w769, "items #"=u16 1 ("Items # [byte]"), "Data Block #"=w759, "S7 Connection in"=w849) -> ("error out"=w808:errorcluster, "STRING result Array"=w807:string[], "S7 Connection out"=w809:T5)  [unwired: 2 in, 1 out]
            n245 = call-poly <vilib>:"read DB.vi"("Item offset [byte]"=u32 68, "String length reserved in DB (default=254)"=u16 10, "error in (no error)"=w808, "items #"=u16 1 ("Items # [byte]"), "Data Block #"=w759, "S7 Connection in"=w809) -> ("error out"=w810:errorcluster, "STRING result Array"=w811:string[], "S7 Connection out"=w758:T5)  [unwired: 2 in, 1 out]
            n246 = Build Array (concatenate)(w807, w811) -> (w805:string[])
            n247 = call "PADMINI_AUTO_BARCODE_STRING 70.vi"("Enum"=enum16{"Read", "Write"}."Write", "error in (no error)"=w810, "Input"=w805) -> ("error out"=w756:errorcluster)  [unwired: 7 in, 1 out]
            n248 = call-poly <vilib>:"read DB.vi"("error in (no error)"=w756, "items #"=u16 2 ("Items # [byte]"), "Data Block #"=w759, "S7 Connection in"=w758) -> ("error out"=w761:errorcluster, "DINT result array"=w763:i32[], "S7 Connection out"=w757:T5)  [unwired: 5 in]
            n249 = call "PADMINI_AUTO_CYCLE STATE 70.vi"("Enum"=enum16{"Read", "Write"}."Write", "error in (no error)"=w761, "Input"=w763) -> ("error out"=w746:errorcluster)  [unwired: 7 in, 1 out]
            n250 = global read "DATA LOG.vi" "OP 80 Outputs"() -> (w829:bool)
            n251 = case shown="True" w829 {
              tunnel: [w875 w878] -> w804
              tunnel: [w874 w879] -> w781
              tunnel: w746 -> [w875 w885]
              tunnel: w757 -> [w874 w882]
              frame False {
              }
              frame True {
                w888 = u16 83  # Data Block #
                n252 = call "PADMINI_AUTO_BARCODE_STATUS 80.vi"("Enum"=enum16{"Read", "Write"}."Read", "error in (no error)"=w885) -> ("error out"=w884:errorcluster, "O/P"=w886:i32[])  [unwired: 8 in]
                n253 = global write "DATA LOG.vi" "OP 80 Outputs"(FALSE) -> ()
                n254 = call-poly <vilib>:"write DB.vi"("DINT input array"=w886, "error in (no error)"=w884, "Data Block #"=w888, "S7 Connection in"=w882) -> ("error out"=w876:errorcluster, "S7 Connection out"=w877:T5)  [unwired: 4 in, 2 out]
                n255 = call-poly <vilib>:"write DB.vi"("DINT input array"=i32[] [0] ("Data Byte"), "error in (no error)"=w876, "Data Block #"=u16 82, "S7 Connection in"=w877) -> ("error out"=w878:errorcluster, "S7 Connection out"=w879:T5)  [unwired: 4 in, 2 out]
              }
            }
            n256 = global read "DATA LOG.vi" "OP 80 reset"() -> (w803:bool)
            n257 = global read "DATA LOG.vi" "Auto Cycle On"() -> (w779:bool)
            n258 = case shown="True" w803 {
              tunnel: w804 -> [w855 w863]
              tunnel: [w855 w858] -> _
              tunnel: [w855 w858] -> w793
              tunnel: w781 -> [w854 w857]
              tunnel: [w854 w856] -> w780
              frame False {
              }
              frame True {
                n259 = global write "DATA LOG.vi" "OP 80 reset"(FALSE) -> ()
                n260 = call-poly <vilib>:"write DB.vi"("Item offset [byte]"=u16 4 ("Data Block #"), "DINT input array"=i32[] [0], "error in (no error)"=w863, "Data Block #"=u16 82, "S7 Connection in"=w857) -> ("error out"=w858:errorcluster, "S7 Connection out"=w856:T5)  [unwired: 3 in, 2 out]
              }
            }
            n261 = Boolean To (0,1)(Boolean=w779) -> (0, 1=w778:i16)
            n262 = Build Array(w778) -> (w777:i16[])
            n263 = global read "Global 1.vi" "Filtered BARCODE selected"() -> (w796:string[])
            n264 = call-poly <vilib>:"write DB.vi"("Item offset [byte]"=u32 20, "DINT input array"=w777, "error in (no error)"=w793, "Data Block #"=w799, "S7 Connection in"=w780) -> ("error out"=w801:errorcluster, "S7 Connection out"=w802:T5)  [unwired: 3 in, 2 out]
            n265 = call-poly <vilib>:"write DB.vi"("Item offset [byte]"=u32 24, "Input STRINGS"=w796, "error in (no error)"=w801, "String length reserved in DB (default=254)"=u16 15, "Data Block #"=w799, "S7 Connection in"=w802) -> ("error out"=w794:errorcluster, "S7 Connection out"=w795:T5)  [unwired: 2 in, 2 out]
            n266 = call-poly <vilib>:"read DB.vi"("Item offset [byte]"=u32 8, "error in (no error)"=w794, "items #"=u16 1 ("Items # [byte]"), "Data Block #"=w783, "S7 Connection in"=w795) -> ("error out"=w837:errorcluster, "REAL result array"=w839:sgl[], "S7 Connection out"=w831:T5)  [unwired: 4 in]
            n267 = call "PADMINI_AUTO_CYCLE VALUE 80.vi"("Enum"=enum16{"Read", "Write"}."Write", "error in (no error)"=w837, "Input"=w839) -> ("error out"=w838:errorcluster)  [unwired: 7 in, 1 out]
            n268 = call "Stall Data Flow.vim"("value in"=w838, "milliseconds to wait"=u32 300) -> ("value out"=w767:errorcluster)  [unwired: 1 out]
            n269 = call-poly <vilib>:"read DB.vi"("Item offset [byte]"=u32 12, "String length reserved in DB (default=254)"=u16 50, "error in (no error)"=w767, "items #"=u16 1 ("Items # [byte]"), "Data Block #"=w783, "S7 Connection in"=w831) -> ("error out"=w788:errorcluster, "STRING result Array"=w786:string[], "S7 Connection out"=w784:T5)  [unwired: 2 in, 1 out]
            n270 = call "Stall Data Flow.vim"("value in"=w788, "milliseconds to wait"=u32 300) -> ("value out"=w765:errorcluster)  [unwired: 1 out]
            n271 = call-poly <vilib>:"read DB.vi"("Item offset [byte]"=u32 64, "String length reserved in DB (default=254)"=u16 10, "error in (no error)"=w765, "items #"=u16 2 ("Items # [byte]"), "Data Block #"=w783, "S7 Connection in"=w784) -> ("error out"=w787:errorcluster, "STRING result Array"=w792:string[], "S7 Connection out"=w748:T5)  [unwired: 2 in, 1 out]
            n272 = Build Array (concatenate)(w786, w792) -> (w785:string[])
            n273 = call "PADMINI_AUTO_BARCODE_STRING 80.vi"("Enum"=enum16{"Read", "Write"}."Write", "error in (no error)"=w787, "Input"=w785) -> ("error out"=w750:errorcluster)  [unwired: 7 in, 1 out]
            n274 = call-poly <vilib>:"read DB.vi"("error in (no error)"=w750, "items #"=u16 2 ("Items # [byte]"), "Data Block #"=u16 82, "S7 Connection in"=w748) -> ("error out"=w754:errorcluster, "DINT result array"=w752:i32[], "S7 Connection out"=w747:T5)  [unwired: 5 in]
            n275 = call "PADMINI_AUTO_CYCLE STATE 80.vi"("Enum"=enum16{"Read", "Write"}."Write", "error in (no error)"=w754, "Input"=w752) -> ("error out"=w751:errorcluster)  [unwired: 7 in, 1 out]
          }
          frame #1 {
            # "RECONNECT"
            n276 = case shown="Error" w907 {
              selector: w907 -> [w912 w913]
              tunnel: [w911 w917] -> w905
              tunnel: [w912 w918] -> w906
              tunnel: w908 -> [w911 w916]
              tunnel: w904 -> [_ w915]
              frame No Error {
              }
              frame Error {
                n277 = Unbundle By Name(w913) -> ("code"=w914:i32)
                n278 = call <vilib>:"Clear Errors.vi"("error in (no error)"=w913) -> ("error out"=w919:errorcluster)  [unwired: 5 in, 1 out]
                n279 = case shown="1, 66" w914 {
                  tunnel: w919 -> [w921 w932]
                  tunnel: [w921 w930] -> w918
                  tunnel: [w922 w929] -> w917
                  tunnel: w916 -> [w922 w926]
                  tunnel: w915 -> [_ w925]
                  tunnel: w913 -> [w920 _]
                  frame 0, Default {
                    n280 = global write "Global 1.vi" "PLC6 error"(w920) -> ()
                  }
                  frame 1, 66 {
                    n281 = call <vilib>:"disconnect.vi"("error in (no error)"=w932, "S7 Connection in"=w926) -> ("error out"=w931:errorcluster)  [unwired: 8 in, 1 out]
                    n282 = call <vilib>:"Clear Errors.vi"("error in (no error)"=w931) -> ("error out"=w928:errorcluster)  [unwired: 5 in, 1 out]
                    n283 = call <vilib>:"connect.vi"("Use Rack/Slot for S71200/1500"=TRUE, "Slot S7 300/400"=u8 1, "PLC Type"=PLC_Type."S7 1200" ("PLC Type 2"), "error in (no error)"=w928, "IP address"=w925) -> ("error out"=w930:errorcluster, "S7 Connection out"=w929:T5)  [unwired: 5 in]
                  }
                }
              }
            }
            n284 = Unbundle By Name(w907) -> ("status"=w910:bool)
            n285 = Not(x=w910) -> (.not. x?=w909:bool)
            "PLC 6" <- w909
            n286 = global write "Global 1.vi" "PLC 6"(w909) -> ()
          }
        }
        n287 = call "PADMINI_STOP_ALL.vi"("Enum"=enum16{"Read", "Write"}."Read") -> ("Boolean 2"=w739:bool)  [unwired: 9 in, 1 out]
        n288 = local read "stop"() -> (w738:bool)
        n289 = Or(x=w738, y=w739) -> (x .or. y?=w737:bool)
        n290 = Wait (ms)(milliseconds to wait=u32 1000) -> ()  [unwired: 1 out]
      }
      n291 = call <vilib>:"Clear Errors.vi"("error in (no error)"=w724) -> ("error out"=w712:errorcluster)  [unwired: 5 in, 1 out]
      n292 = call <vilib>:"disconnect.vi"("error in (no error)"=w712, "S7 Connection in"=w723) -> ("error out"=w711:errorcluster)  [unwired: 8 in, 1 out]
    }
    frame Enabled {
      w934 = PLC_Comm_State."Int"  # Enum
      n293 = while {
        shift-right: [w948] -> _
        shift-left: w934 -> [w956]
        shift-right: [w940] -> w933
        shift-left: w935 -> [w955]
        shift-right: [w951] -> _
        shift-left: _ -> [w954]
        tunnel: w936 -> [w937]
        stop <- w949 stop-if-true
        w945 = PLC_Comm_State."Disconnect"  # Enum
        w953 = u32 800  # milliseconds to wait
        # "Int-->Write-->Read---if--Error-->reconnect\n               ^------v                                       v\n                ^------------------------------v"
        # "OP 70-80"
        n294 = case shown="\"Int\"" w956 {
          selector: w956 -> [w972 w990 w1027 w1079 w1133 w1170 w1183 w1187 _ _]
          tunnel: [w977 w992 w1007 w1061 w1107 w1146 w1184 w1192 w1195 w1197] -> w957
          tunnel: [w978 w991 w1006 w1062 w1106 w1145 w1185 w1189 w1194 w1196] -> w950
          tunnel: w955 -> [w975 w986 w1008 w1060 w1108 w1143 w1181 w1190 w1195 w1197]
          tunnel: w954 -> [w973 _ w1009 w1059 w1109 w1144 w1185 w1191 w1194 w1196]
          tunnel: [w971 w989 w1026 w1080 w1132 w1171 w1182 w1186 _ _] -> w952
          tunnel: [_ _ _ _ _ _ _ TRUE _ _] -> w949
          tunnel: [w972 w990 w1027 w1079 w1133 w1170 w1183 w1187 _ _] -> w946
          tunnel: w937 -> [w970 w988 _ _ _ _ _ _ _ _]
          frame "Connect" {
            w971 = PLC_Comm_State."Write"  # Enum
            w983 = TRUE  # Use Rack/Slot for S71200/1500
            w982 = u8 1  # Slot S7 300/400
            w980 = u8 0  # Rack S7 300/400
            # "Reconect"
            n295 = call <vilib>:"disconnect.vi"("error in (no error)"=w975, "S7 Connection in"=w973) -> ("error out"=w976:errorcluster)  [unwired: 8 in, 1 out]
            n296 = call <vilib>:"Clear Errors.vi"("error in (no error)"=w976) -> ("error out"=w974:errorcluster)  [unwired: 5 in, 1 out]
            n297 = call <vilib>:"connect.vi"("Use Rack/Slot for S71200/1500"=w983, "Slot S7 300/400"=w982, "PLC Type"=PLC_Type."S7 1200" ("PLC Type 2"), "error in (no error)"=w974, "Rack S7 300/400"=w980, "timeout [ms]"=1000 ("timeout [ms] 2"), "IP address"=w970) -> ("error out"=w977:errorcluster, "S7 Connection out"=w978:T5)  [unwired: 3 in]
          }
          frame "Int" {
            w989 = PLC_Comm_State."Write"  # Enum
            w993 = TRUE  # Use Rack/Slot for S71200/1500
            w994 = u8 1  # Slot S7 300/400
            w995 = u8 0  # Rack S7 300/400
            # "Initialize and set first bits"
            n298 = call "Stall Data Flow.vim"("value in"=w986, "milliseconds to wait"=u32 645) -> ("value out"=w985:errorcluster)  [unwired: 1 out]
            n299 = call <vilib>:"connect.vi"("Use Rack/Slot for S71200/1500"=w993, "Slot S7 300/400"=w994, "PLC Type"=PLC_Type."S7 1200" ("PLC Type 2"), "error in (no error)"=w985, "Rack S7 300/400"=w995, "timeout [ms]"=1000 ("timeout [ms] 2"), "IP address"=w988) -> ("error out"=w997:errorcluster, "S7 Connection out"=w996:T5)  [unwired: 3 in]
            n300 = for {
              tunnel: u16[] [80, 82] ("Data Block #") -> [w1005] mode=indexing
              shift-right: [w1003] -> w991
              shift-left: w996 -> [w1001]
              tunnel: w997 -> [w1002]
              tunnel: [w1000] -> w992
              w1004 = i32[] [0, 0]  # DINT input array
              # "Reset Search and save \nbit on software start"
              n301 = call-poly <vilib>:"write DB.vi"("DINT input array"=w1004, "error in (no error)"=w1002, "Data Block #"=w1005, "S7 Connection in"=w1001) -> ("error out"=w1000:errorcluster, "S7 Connection out"=w1003:T5)  [unwired: 4 in, 2 out]
            }
          }
          frame "Write" {
            w1011 = u16 81 ("Data Block #")
            w1026 = PLC_Comm_State."Write2"  # Enum
            # "OP 70 Write"
            n302 = global read "DATA LOG.vi" "OP 70 Outputs"() -> (w1025:bool)
            n303 = case shown="True" w1025 {
              tunnel: w1009 -> [w1041 w1054]
              tunnel: [w1042 w1043] -> w1023
              tunnel: [w1041 w1047] -> w1022
              tunnel: w1008 -> [w1042 w1051]
              frame False {
              }
              frame True {
                w1055 = u16 81  # Data Block #
                n304 = call "PADMINI_AUTO_BARCODE_STATUS 70.vi"("Enum"=enum16{"Read", "Write"}."Read", "error in (no error)"=w1051) -> ("error out"=w1050:errorcluster, "O/P"=w1052:i32[])  [unwired: 8 in]
                n305 = call-poly <vilib>:"write DB.vi"("DINT input array"=w1052, "error in (no error)"=w1050, "Data Block #"=w1055, "S7 Connection in"=w1054) -> ("error out"=w1045:errorcluster, "S7 Connection out"=w1046:T5)  [unwired: 4 in, 2 out]
                n306 = call-poly <vilib>:"write DB.vi"("DINT input array"=i32[] [0] ("Data Byte"), "error in (no error)"=w1045, "Data Block #"=u16 80, "S7 Connection in"=w1046) -> ("error out"=w1044:errorcluster, "S7 Connection out"=w1047:T5)  [unwired: 4 in, 2 out]
                n307 = case shown="No Error" w1044 {
                  selector: w1044 -> [w1056 w1058]
                  tunnel: [w1056 w1058] -> w1043
                  frame No Error {
                    n308 = global write "DATA LOG.vi" "OP 70 Outputs"(FALSE) -> ()
                  }
                  frame Error {
                  }
                }
              }
            }
            n309 = global read "DATA LOG.vi" "OP 70 reset"() -> (w1024:bool)
            n310 = global read "DATA LOG.vi" "Auto Cycle On"() -> (w1016:bool)
            n311 = case shown="True" w1024 {
              tunnel: w1023 -> [w1028 w1037]
              tunnel: [w1028 w1030] -> w1017
              tunnel: w1022 -> [w1029 w1036]
              tunnel: [w1029 w1035] -> w1018
              frame False {
              }
              frame True {
                n312 = call-poly <vilib>:"write DB.vi"("Item offset [byte]"=u16 4 ("Data Block #"), "DINT input array"=i32[] [0], "error in (no error)"=w1037, "Data Block #"=u16 80, "S7 Connection in"=w1036) -> ("error out"=w1031:errorcluster, "S7 Connection out"=w1035:T5)  [unwired: 3 in, 2 out]
                n313 = case shown="No Error" w1031 {
                  selector: w1031 -> [w1038 w1040]
                  tunnel: [w1038 w1040] -> w1030
                  frame No Error {
                    n314 = global write "DATA LOG.vi" "OP 70 reset"(FALSE) -> ()
                  }
                  frame Error {
                  }
                }
              }
            }
            n315 = Boolean To (0,1)(Boolean=w1016) -> (0, 1=w1015:i16)
            n316 = Build Array(w1015) -> (w1014:i16[])
            n317 = global read "Global 1.vi" "Filtered BARCODE selected"() -> (w1019:string[])
            n318 = call-poly <vilib>:"write DB.vi"("Item offset [byte]"=u32 20, "DINT input array"=w1014, "error in (no error)"=w1017, "Data Block #"=w1011, "S7 Connection in"=w1018) -> ("error out"=w1020:errorcluster, "S7 Connection out"=w1021:T5)  [unwired: 3 in, 2 out]
            n319 = call-poly <vilib>:"write DB.vi"("Item offset [byte]"=u32 24, "Input STRINGS"=w1019, "error in (no error)"=w1020, "String length reserved in DB (default=254)"=u16 15, "Data Block #"=w1011, "S7 Connection in"=w1021) -> ("error out"=w1007:errorcluster, "S7 Connection out"=w1006:T5)  [unwired: 2 in, 2 out]
          }
          frame "Write2" {
            w1064 = u16 83 ("Data Block #")
            w1080 = PLC_Comm_State."Read"  # Enum
            # "op 80 wirte 2"
            n320 = global read "DATA LOG.vi" "OP 80 Outputs"() -> (w1078:bool)
            n321 = case shown="True" w1078 {
              tunnel: [w1092 w1094] -> w1077
              tunnel: [w1091 w1097] -> w1071
              tunnel: w1060 -> [w1092 w1102]
              tunnel: w1059 -> [w1091 w1100]
              frame False {
              }
              frame True {
                w1105 = u16 83  # Data Block #
                n322 = call "PADMINI_AUTO_BARCODE_STATUS 80.vi"("Enum"=enum16{"Read", "Write"}."Read", "error in (no error)"=w1102) -> ("error out"=w1101:errorcluster, "O/P"=w1103:i32[])  [unwired: 8 in]
                n323 = call-poly <vilib>:"write DB.vi"("DINT input array"=w1103, "error in (no error)"=w1101, "Data Block #"=w1105, "S7 Connection in"=w1100) -> ("error out"=w1095:errorcluster, "S7 Connection out"=w1096:T5)  [unwired: 4 in, 2 out]
                n324 = call-poly <vilib>:"write DB.vi"("DINT input array"=i32[] [0] ("Data Byte"), "error in (no error)"=w1095, "Data Block #"=u16 82, "S7 Connection in"=w1096) -> ("error out"=w1094:errorcluster, "S7 Connection out"=w1097:T5)  [unwired: 4 in, 2 out]
                n325 = Unbundle By Name(w1094) -> ("status"=w1093:bool)
                n326 = global write "DATA LOG.vi" "OP 80 Outputs"(w1093) -> ()
              }
            }
            n327 = global read "DATA LOG.vi" "OP 80 reset"() -> (w1076:bool)
            n328 = case shown="True" w1076 {
              tunnel: w1077 -> [w1082 w1090]
              tunnel: [w1082 w1084] -> _
              tunnel: [w1082 w1084] -> w1072
              tunnel: w1071 -> [w1081 w1086]
              tunnel: [w1081 w1085] -> w1070
              frame False {
              }
              frame True {
                n329 = call-poly <vilib>:"write DB.vi"("Item offset [byte]"=u16 4 ("Data Block #"), "DINT input array"=i32[] [0], "error in (no error)"=w1090, "Data Block #"=u16 82, "S7 Connection in"=w1086) -> ("error out"=w1084:errorcluster, "S7 Connection out"=w1085:T5)  [unwired: 3 in, 2 out]
                n330 = Unbundle By Name(w1084) -> ("status"=w1083:bool)
                n331 = global write "DATA LOG.vi" "OP 80 reset"(w1083) -> ()
              }
            }
            n332 = global read "DATA LOG.vi" "Auto Cycle On"() -> (w1069:bool)
            n333 = Boolean To (0,1)(Boolean=w1069) -> (0, 1=w1068:i16)
            n334 = Build Array(w1068) -> (w1067:i16[])
            n335 = global read "Global 1.vi" "Filtered BARCODE selected"() -> (w1073:string[])
            n336 = call-poly <vilib>:"write DB.vi"("Item offset [byte]"=u32 20, "DINT input array"=w1067, "error in (no error)"=w1072, "Data Block #"=w1064, "S7 Connection in"=w1070) -> ("error out"=w1074:errorcluster, "S7 Connection out"=w1075:T5)  [unwired: 3 in, 2 out]
            n337 = call-poly <vilib>:"write DB.vi"("Item offset [byte]"=u32 24, "Input STRINGS"=w1073, "error in (no error)"=w1074, "String length reserved in DB (default=254)"=u16 15, "Data Block #"=w1064, "S7 Connection in"=w1075) -> ("error out"=w1061:errorcluster, "S7 Connection out"=w1062:T5)  [unwired: 2 in, 2 out]
          }
          frame "Read" {
            w1118 = u16 80 ("Data Block #")
            w1132 = PLC_Comm_State."Read2"  # Enum
            # "OP70 read"
            n338 = call-poly <vilib>:"read DB.vi"("Item offset [byte]"=u32 8, "error in (no error)"=w1108, "items #"=u16 2 ("Items # [byte]"), "Data Block #"=w1118, "S7 Connection in"=w1109) -> ("error out"=w1128:errorcluster, "REAL result array"=w1131:sgl[], "S7 Connection out"=w1129:T5)  [unwired: 4 in]
            n339 = call-poly <vilib>:"read DB.vi"("Item offset [byte]"=u32 16, "String length reserved in DB (default=254)"=u16 50, "error in (no error)"=w1128, "items #"=u16 1 ("Items # [byte]"), "Data Block #"=w1118, "S7 Connection in"=w1129) -> ("error out"=w1124:errorcluster, "STRING result Array"=w1123:string[], "S7 Connection out"=w1125:T5)  [unwired: 2 in, 1 out]
            n340 = call-poly <vilib>:"read DB.vi"("Item offset [byte]"=u32 68, "String length reserved in DB (default=254)"=u16 10, "error in (no error)"=w1124, "items #"=u16 1 ("Items # [byte]"), "Data Block #"=w1118, "S7 Connection in"=w1125) -> ("error out"=w1126:errorcluster, "STRING result Array"=w1127:string[], "S7 Connection out"=w1120:T5)  [unwired: 2 in, 1 out]
            n341 = Build Array (concatenate)(w1123, w1127) -> (w1130:string[])
            n342 = call-poly <vilib>:"read DB.vi"("error in (no error)"=w1126, "items #"=u16 2 ("Items # [byte]"), "Data Block #"=w1118, "S7 Connection in"=w1120) -> ("error out"=w1121:errorcluster, "DINT result array"=w1122:i32[], "S7 Connection out"=w1106:T5)  [unwired: 5 in]
            n343 = case shown="No Error" w1121 {
              selector: w1121 -> [w1136 w1142]
              tunnel: w1122 -> [w1141 _]
              tunnel: w1130 -> [w1140 _]
              tunnel: w1131 -> [w1137 _]
              tunnel: [w1135 w1142] -> w1107
              frame No Error {
                w1139 = enum16{"Read", "Write"}."Write" ("Enum")
                n344 = call "PADMINI_AUTO_BARCODE_STRING 70.vi"("Enum"=w1139, "error in (no error)"=w1136, "Input"=w1140) -> ("error out"=w1138:errorcluster)  [unwired: 7 in, 1 out]
                n345 = call "PADMINI_AUTO_CYCLE VALUE 70.vi"("Enum"=w1139, "error in (no error)"=w1138, "Input"=w1137) -> ("error out"=w1134:errorcluster)  [unwired: 7 in, 1 out]
                n346 = call "PADMINI_AUTO_CYCLE STATE 70.vi"("Enum"=w1139, "error in (no error)"=w1134, "Input"=w1141) -> ("error out"=w1135:errorcluster)  [unwired: 7 in, 1 out]
              }
              frame Error {
              }
            }
          }
          frame "Read2" {
            w1152 = u16 82 ("Data Block #")
            w1171 = PLC_Comm_State."Write"  # Enum
            # "Op80 Read2"
            n347 = call-poly <vilib>:"read DB.vi"("Item offset [byte]"=u32 8, "error in (no error)"=w1143, "items #"=u16 1 ("Items # [byte]"), "Data Block #"=w1152, "S7 Connection in"=w1144) -> ("error out"=w1158:errorcluster, "REAL result array"=w1169:sgl[], "S7 Connection out"=w1159:T5)  [unwired: 4 in]
            n348 = call-poly <vilib>:"read DB.vi"("Item offset [byte]"=u32 12, "String length reserved in DB (default=254)"=u16 50, "error in (no error)"=w1158, "items #"=u16 1 ("Items # [byte]"), "Data Block #"=w1152, "S7 Connection in"=w1159) -> ("error out"=w1161:errorcluster, "STRING result Array"=w1163:string[], "S7 Connection out"=w1164:T5)  [unwired: 2 in, 1 out]
            n349 = call-poly <vilib>:"read DB.vi"("Item offset [byte]"=u32 64, "String length reserved in DB (default=254)"=u16 10, "error in (no error)"=w1161, "items #"=u16 2 ("Items # [byte]"), "Data Block #"=w1152, "S7 Connection in"=w1164) -> ("error out"=w1162:errorcluster, "STRING result Array"=w1160:string[], "S7 Connection out"=w1167:T5)  [unwired: 2 in, 1 out]
            n350 = Build Array (concatenate)(w1163, w1160) -> (w1168:string[])
            n351 = call-poly <vilib>:"read DB.vi"("error in (no error)"=w1162, "items #"=u16 2 ("Items # [byte]"), "Data Block #"=u16 82, "S7 Connection in"=w1167) -> ("error out"=w1165:errorcluster, "DINT result array"=w1166:i32[], "S7 Connection out"=w1145:T5)  [unwired: 5 in]
            n352 = case shown="No Error" w1165 {
              selector: w1165 -> [w1174 w1180]
              tunnel: w1166 -> [w1179 _]
              tunnel: w1168 -> [w1177 _]
              tunnel: w1169 -> [w1176 _]
              tunnel: [w1172 w1180] -> w1146
              frame No Error {
                w1175 = enum16{"Read", "Write"}."Write" ("Enum")
                n353 = call "PADMINI_AUTO_CYCLE VALUE 80.vi"("Enum"=w1175, "error in (no error)"=w1174, "Input"=w1176) -> ("error out"=w1178:errorcluster)  [unwired: 7 in, 1 out]
                n354 = call "PADMINI_AUTO_BARCODE_STRING 80.vi"("Enum"=w1175, "error in (no error)"=w1178, "Input"=w1177) -> ("error out"=w1173:errorcluster)  [unwired: 7 in, 1 out]
                n355 = call "PADMINI_AUTO_CYCLE STATE 80.vi"("Enum"=w1175, "error in (no error)"=w1173, "Input"=w1179) -> ("error out"=w1172:errorcluster)  [unwired: 7 in, 1 out]
              }
              frame Error {
              }
            }
          }
          frame "Error" {
            w1182 = PLC_Comm_State."Connect"  # Enum
            n356 = global write "Global 1.vi" "PLC6 error"(w1181) -> ()
            n357 = call <vilib>:"Clear Errors.vi"("error in (no error)"=w1181) -> ("error out"=w1184:errorcluster)  [unwired: 5 in, 1 out]
          }
          frame "Disconnect" {
            w1186 = PLC_Comm_State."Disconnect"  # Enum
            w1189 = T5 {"TCP Connection Ref"=refnum, "IP address"="", "timeout ms"=5000, "Connected?"=FALSE, "PLC Type"=enum."S7 1200", "Rack S7 400"=0, "Slot S7 400"=0, "PDU Size"=0, "connection semaphore"=refnum}  # S7 Connection out
            n358 = call <vilib>:"Clear Errors.vi"("error in (no error)"=w1190) -> ("error out"=w1193:errorcluster)  [unwired: 5 in, 1 out]
            n359 = call <vilib>:"disconnect.vi"("error in (no error)"=w1193, "S7 Connection in"=w1191) -> ("error out"=w1192:errorcluster)  [unwired: 8 in, 1 out]
          }
          frame "Write3" {
            # "No Use"
          }
          frame "Read3" {
            # "No Use"
          }
        }
        n360 = Wait (ms)(milliseconds to wait=w953) -> ()  [unwired: 1 out]
        n361 = call "PADMINI_STOP_ALL.vi"("Enum"=enum16{"Read", "Write"}."Read") -> ("Boolean 2"=w944:bool)  [unwired: 9 in, 1 out]
        n362 = local read "stop"() -> (w939:bool)
        n363 = case shown="Error" w957 {
          selector: w957 -> [w960 w963]
          tunnel: [w960 w962] -> w940
          tunnel: [w959 w961] -> w947
          tunnel: w952 -> [w959 _]
          tunnel: [w958 w969] -> w951
          tunnel: w950 -> [w958 w969]
          tunnel: w946 -> [_ w967]
          frame No Error {
          }
          frame Error {
            w961 = PLC_Comm_State."Error"  # Enum
            n364 = Unbundle By Name(w963) -> ("source"=w968:string)
            n365 = call <userlib>:"Get Strings from Enum__ogtk.vi"("Enum"=w967) -> ("String Value"=w966:string)  [unwired: 7 in, 3 out]
            n366 = Concatenate Strings(w966, "    " ("string"), w968) -> (w964:string)
            n367 = Bundle By Name(cluster=w963, "source"=w964) -> (w962:errorcluster)
          }
        }
        n368 = Or(x=w939, y=w944) -> (x .or. y?=w942:bool)
        n369 = Select(t=w945, s=w942, f=w947) -> (s? t:f=w948:T1)
        n370 = Unbundle By Name(w940) -> ("status"=w941:bool)
        n371 = Not(x=w941) -> (.not. x?=w938:bool)
        n372 = global write "Global 1.vi" "PLC 6"(w938) -> ()
      }
    }
  }
  n373 = disable-structure shown="Enabled" {
    disable-tunnel: w29 -> [w1210 w1410]
    disable-tunnel: [w1209 w1408] -> w2
    disable-tunnel: w9 -> [w1203 w1409]
    frame Disabled {
      w1200 = TRUE  # Use Rack/Slot for S71200/1500
      w1201 = u8 1  # Slot S7 300/400
      w1202 = u8 0  # Rack S7 300/400
      n374 = call <vilib>:"connect.vi"("Use Rack/Slot for S71200/1500"=w1200, "Slot S7 300/400"=w1201, "PLC Type"=PLC_Type."S7 1200" ("PLC Type 2"), "error in (no error)"=w1203, "Rack S7 300/400"=w1202, "timeout [ms]"=1000 ("timeout [ms] 2"), "IP address"=w1210) -> ("error out"=w1205:errorcluster, "S7 Connection out"=w1204:T5)  [unwired: 3 in]
      n375 = for {
        tunnel: u16[] [69, 71] ("Data Block #") -> [w1218] mode=indexing
        shift-right: [w1216] -> w1207
        shift-left: w1204 -> [w1213]
        tunnel: w1205 -> [w1214]
        tunnel: [w1215] -> w1206
        w1217 = i32[] [0, 0]  # DINT input array
        # "Reset Search and save \nbit on software start"
        n376 = call-poly <vilib>:"write DB.vi"("DINT input array"=w1217, "error in (no error)"=w1214, "Data Block #"=w1218, "S7 Connection in"=w1213) -> ("error out"=w1215:errorcluster, "S7 Connection out"=w1216:T5)  [unwired: 4 in, 2 out]
      }
      n377 = while {
        shift-right: [w1221] -> w1198
        shift-left: w1207 -> [w1231]
        shift-right: [w1229] -> w1209
        shift-left: w1206 -> [w1230]
        tunnel: w1210 -> [w1220]
        stop <- w1223 stop-if-true
        # "OP 90 - 100"
        n378 = flat-sequence {
          tunnel: [w1233] -> w1227
          tunnel: [w1303] -> w1222
          tunnel: w1230 -> [w1328]
          tunnel: w1231 -> [w1327]
          tunnel: w1220 -> [w1315]
          tunnel: [w1315] -> w1219
          tunnel: [w1381] -> w1229
          tunnel: [w1380] -> w1221
          tunnel: w1227 -> [w1383]
          tunnel: w1222 -> [w1382]
          tunnel: w1219 -> [w1379]
          frame #0 {
            w1272 = u16 72 ("Data Block #")
            w1296 = u16 70 ("Data Block #")
            w1232 = u16 71 ("Data Block #")
            w1240 = u16 69 ("Data Block #")
            # "AUTO WRITE"
            n379 = global read "DATA LOG.vi" "OP 90 Outputs"() -> (w1326:bool)
            n380 = case shown="True" w1326 {
              tunnel: w1327 -> [w1364 w1377]
              tunnel: [w1365 w1366] -> w1301
              tunnel: [w1364 w1367] -> w1302
              tunnel: w1328 -> [w1365 w1374]
              frame False {
              }
              frame True {
                w1378 = u16 70  # Data Block #
                n381 = call "PADMINI_AUTO_BARCODE_STATUS 90.vi"("Enum"=enum16{"Read", "Write"}."Read", "error in (no error)"=w1374) -> ("error out"=w1373:errorcluster, "O/P"=w1375:i32[])  [unwired: 8 in]
                n382 = global write "DATA LOG.vi" "OP 90 Outputs"(FALSE) -> ()
                n383 = call-poly <vilib>:"write DB.vi"("DINT input array"=w1375, "error in (no error)"=w1373, "Data Block #"=w1378, "S7 Connection in"=w1377) -> ("error out"=w1369:errorcluster, "S7 Connection out"=w1368:T5)  [unwired: 4 in, 2 out]
                n384 = call-poly <vilib>:"write DB.vi"("DINT input array"=i32[] [0] ("Data Byte"), "error in (no error)"=w1369, "Data Block #"=u16 69, "S7 Connection in"=w1368) -> ("error out"=w1366:errorcluster, "S7 Connection out"=w1367:T5)  [unwired: 4 in, 2 out]
              }
            }
            n385 = global read "DATA LOG.vi" "OP 90 reset"() -> (w1300:bool)
            n386 = case shown="True" w1300 {
              tunnel: w1301 -> [w1339 w1348]
              tunnel: [w1339 w1347] -> w1289
              tunnel: w1302 -> [w1340 w1346]
              tunnel: [w1340 w1345] -> w1290
              frame False {
              }
              frame True {
                n387 = global write "DATA LOG.vi" "OP 90 reset"(FALSE) -> ()
                n388 = call-poly <vilib>:"write DB.vi"("Item offset [byte]"=u16 4 ("Data Block #"), "DINT input array"=i32[] [0], "error in (no error)"=w1348, "Data Block #"=u16 69, "S7 Connection in"=w1346) -> ("error out"=w1347:errorcluster, "S7 Connection out"=w1345:T5)  [unwired: 3 in, 2 out]
              }
            }
            n389 = global read "DATA LOG.vi" "Auto Cycle On"() -> (w1255:bool)
            n390 = Boolean To (0,1)(Boolean=w1255) -> (0, 1=w1254:i16)
            n391 = Build Array(w1254) -> (w1253:i16[])
            n392 = global read "Global 1.vi" "Filtered BARCODE selected"() -> (w1299:string[])
            n393 = call-poly <vilib>:"write DB.vi"("Item offset [byte]"=u32 20, "DINT input array"=w1253, "error in (no error)"=w1289, "Data Block #"=w1296, "S7 Connection in"=w1290) -> ("error out"=w1294:errorcluster, "S7 Connection out"=w1293:T5)  [unwired: 3 in, 2 out]
            n394 = call-poly <vilib>:"write DB.vi"("Item offset [byte]"=u32 24, "Input STRINGS"=w1299, "error in (no error)"=w1294, "String length reserved in DB (default=254)"=u16 15, "Data Block #"=w1296, "S7 Connection in"=w1293) -> ("error out"=w1291:errorcluster, "S7 Connection out"=w1292:T5)  [unwired: 2 in, 2 out]
            n395 = call-poly <vilib>:"read DB.vi"("Item offset [byte]"=u32 8, "error in (no error)"=w1291, "items #"=u16 2 ("Items # [byte]"), "Data Block #"=w1240, "S7 Connection in"=w1292) -> ("error out"=w1318:errorcluster, "REAL result array"=w1316:sgl[], "S7 Connection out"=w1324:T5)  [unwired: 4 in]
            n396 = call "PADMINI_AUTO_CYCLE VALUE 90.vi"("Enum"=enum16{"Read", "Write"}."Write", "error in (no error)"=w1318, "Input"=w1316) -> ("error out"=w1317:errorcluster)  [unwired: 7 in, 1 out]
            n397 = call-poly <vilib>:"read DB.vi"("Item offset [byte]"=u32 16, "String length reserved in DB (default=254)"=u16 50, "error in (no error)"=w1317, "items #"=u16 1 ("Items # [byte]"), "Data Block #"=w1240, "S7 Connection in"=w1324) -> ("error out"=w1288:errorcluster, "STRING result Array"=w1281:string[], "S7 Connection out"=w1287:T5)  [unwired: 2 in, 1 out]
            n398 = call-poly <vilib>:"read DB.vi"("Item offset [byte]"=u32 68, "String length reserved in DB (default=254)"=u16 10, "error in (no error)"=w1288, "items #"=u16 3 ("Items # [byte]"), "Data Block #"=w1240, "S7 Connection in"=w1287) -> ("error out"=w1286:errorcluster, "STRING result Array"=w1280:string[], "S7 Connection out"=w1243:T5)  [unwired: 2 in, 1 out]
            n399 = Build Array (concatenate)(w1281, w1280) -> (w1279:string[])
            n400 = call "PADMINI_AUTO_BARCODE_STRING 90.vi"("Enum"=enum16{"Read", "Write"}."Write", "error in (no error)"=w1286, "Input"=w1279) -> ("error out"=w1242:errorcluster)  [unwired: 7 in, 1 out]
            n401 = call-poly <vilib>:"read DB.vi"("error in (no error)"=w1242, "items #"=u16 2 ("Items # [byte]"), "Data Block #"=w1240, "S7 Connection in"=w1243) -> ("error out"=w1246:errorcluster, "DINT result array"=w1248:i32[], "S7 Connection out"=w1244:T5)  [unwired: 5 in]
            n402 = call "PADMINI_AUTO_CYCLE STATE 90.vi"("Enum"=enum16{"Read", "Write"}."Write", "error in (no error)"=w1246, "Input"=w1248) -> ("error out"=w1241:errorcluster)  [unwired: 7 in, 1 out]
            n403 = global read "DATA LOG.vi" "OP 100 Outputs"() -> (w1304:bool)
            n404 = case shown="True" w1304 {
              tunnel: w1244 -> [w1349 w1362]
              tunnel: [w1350 w1353] -> w1277
              tunnel: [w1349 w1354] -> w1278
              tunnel: w1241 -> [w1350 w1359]
              frame False {
              }
              frame True {
                w1363 = u16 72  # Data Block #
                n405 = call "PADMINI_AUTO_BARCODE_STATUS 100.vi"("Enum"=enum16{"Read", "Write"}."Read", "error in (no error)"=w1359) -> ("error out"=w1358:errorcluster, "O/P"=w1360:i32[])  [unwired: 8 in]
                n406 = global write "DATA LOG.vi" "OP 100 Outputs"(FALSE) -> ()
                n407 = call-poly <vilib>:"write DB.vi"("DINT input array"=w1360, "error in (no error)"=w1358, "Data Block #"=w1363, "S7 Connection in"=w1362) -> ("error out"=w1352:errorcluster, "S7 Connection out"=w1351:T5)  [unwired: 4 in, 2 out]
                n408 = call-poly <vilib>:"write DB.vi"("DINT input array"=i32[] [0] ("Data Byte"), "error in (no error)"=w1352, "Data Block #"=u16 71, "S7 Connection in"=w1351) -> ("error out"=w1353:errorcluster, "S7 Connection out"=w1354:T5)  [unwired: 4 in, 2 out]
              }
            }
            n409 = global read "DATA LOG.vi" "OP 100 reset"() -> (w1276:bool)
            n410 = case shown="True" w1276 {
              tunnel: w1277 -> [w1329 w1338]
              tunnel: [w1329 w1337] -> w1268
              tunnel: w1278 -> [w1330 w1336]
              tunnel: [w1330 w1335] -> w1267
              frame False {
              }
              frame True {
                n411 = global write "DATA LOG.vi" "OP 100 reset"(FALSE) -> ()
                n412 = call-poly <vilib>:"write DB.vi"("Item offset [byte]"=u16 4 ("Data Block #"), "DINT input array"=i32[] [0], "error in (no error)"=w1338, "Data Block #"=u16 71, "S7 Connection in"=w1336) -> ("error out"=w1337:errorcluster, "S7 Connection out"=w1335:T5)  [unwired: 3 in, 2 out]
              }
            }
            n413 = global read "DATA LOG.vi" "Auto Cycle On"() -> (w1252:bool)
            n414 = Boolean To (0,1)(Boolean=w1252) -> (0, 1=w1251:i16)
            n415 = Build Array(w1251) -> (w1250:i16[])
            n416 = global read "Global 1.vi" "Filtered BARCODE selected"() -> (w1269:string[])
            n417 = call-poly <vilib>:"write DB.vi"("Item offset [byte]"=u32 20, "DINT input array"=w1250, "error in (no error)"=w1268, "Data Block #"=w1272, "S7 Connection in"=w1267) -> ("error out"=w1274:errorcluster, "S7 Connection out"=w1275:T5)  [unwired: 3 in, 2 out]
            n418 = call-poly <vilib>:"write DB.vi"("Item offset [byte]"=u32 24, "Input STRINGS"=w1269, "error in (no error)"=w1274, "String length reserved in DB (default=254)"=u16 15, "Data Block #"=w1272, "S7 Connection in"=w1275) -> ("error out"=w1265:errorcluster, "S7 Connection out"=w1266:T5)  [unwired: 2 in, 2 out]
            n419 = call-poly <vilib>:"read DB.vi"("Item offset [byte]"=u32 8, "error in (no error)"=w1265, "items #"=u16 11 ("Items # [byte]"), "Data Block #"=w1232, "S7 Connection in"=w1266) -> ("error out"=w1312:errorcluster, "REAL result array"=w1314:sgl[], "S7 Connection out"=w1306:T5)  [unwired: 4 in]
            n420 = call "PADMINI_AUTO_CYCLE VALUE 100.vi"("Enum"=enum16{"Read", "Write"}."Write", "error in (no error)"=w1312, "Input"=w1314) -> ("error out"=w1313:errorcluster)  [unwired: 7 in, 1 out]
            n421 = call-poly <vilib>:"read DB.vi"("Item offset [byte]"=u32 52, "String length reserved in DB (default=254)"=u16 50, "error in (no error)"=w1313, "items #"=u16 1 ("Items # [byte]"), "Data Block #"=w1232, "S7 Connection in"=w1306) -> ("error out"=w1262:errorcluster, "STRING result Array"=w1260:string[], "S7 Connection out"=w1261:T5)  [unwired: 2 in, 1 out]
            n422 = call-poly <vilib>:"read DB.vi"("Item offset [byte]"=u32 104, "String length reserved in DB (default=254)"=u16 10, "error in (no error)"=w1262, "items #"=u16 2 ("Items # [byte]"), "Data Block #"=w1232, "S7 Connection in"=w1261) -> ("error out"=w1263:errorcluster, "STRING result Array"=w1258:string[], "S7 Connection out"=w1234:T5)  [unwired: 2 in, 1 out]
            n423 = Build Array (concatenate)(w1260, w1258) -> (w1259:string[])
            n424 = call "PADMINI_AUTO_BARCODE_STRING 100.vi"("Enum"=enum16{"Read", "Write"}."Write", "error in (no error)"=w1263, "Input"=w1259) -> ("error out"=w1235:errorcluster)  [unwired: 7 in, 1 out]
            n425 = call-poly <vilib>:"read DB.vi"("error in (no error)"=w1235, "items #"=u16 2 ("Items # [byte]"), "Data Block #"=w1232, "S7 Connection in"=w1234) -> ("error out"=w1238:errorcluster, "DINT result array"=w1239:i32[], "S7 Connection out"=w1233:T5)  [unwired: 5 in]
            n426 = call "PADMINI_AUTO_CYCLE STATE 100.vi"("Enum"=enum16{"Read", "Write"}."Write", "error in (no error)"=w1238, "Input"=w1239) -> ("error out"=w1303:errorcluster)  [unwired: 7 in, 1 out]
          }
          frame #1 {
            # "RECONNECT"
            n427 = case shown="Error" w1382 {
              selector: w1382 -> [w1387 w1388]
              tunnel: [w1386 w1392] -> w1380
              tunnel: [w1387 w1393] -> w1381
              tunnel: w1383 -> [w1386 w1391]
              tunnel: w1379 -> [_ w1390]
              frame No Error {
              }
              frame Error {
                n428 = Unbundle By Name(w1388) -> ("code"=w1389:i32)
                n429 = call <vilib>:"Clear Errors.vi"("error in (no error)"=w1388) -> ("error out"=w1394:errorcluster)  [unwired: 5 in, 1 out]
                n430 = case shown="1, 66" w1389 {
                  tunnel: w1394 -> [w1396 w1407]
                  tunnel: [w1396 w1405] -> w1393
                  tunnel: [w1397 w1404] -> w1392
                  tunnel: w1391 -> [w1397 w1401]
                  tunnel: w1390 -> [_ w1400]
                  tunnel: w1388 -> [w1395 _]
                  frame 0, Default {
                    n431 = global write "Global 1.vi" "PLC7 error"(w1395) -> ()
                  }
                  frame 1, 66 {
                    n432 = call <vilib>:"disconnect.vi"("error in (no error)"=w1407, "S7 Connection in"=w1401) -> ("error out"=w1406:errorcluster)  [unwired: 8 in, 1 out]
                    n433 = call <vilib>:"Clear Errors.vi"("error in (no error)"=w1406) -> ("error out"=w1403:errorcluster)  [unwired: 5 in, 1 out]
                    n434 = call <vilib>:"connect.vi"("Use Rack/Slot for S71200/1500"=TRUE, "Slot S7 300/400"=u8 1, "PLC Type"=PLC_Type."S7 1200" ("PLC Type 2"), "error in (no error)"=w1403, "IP address"=w1400) -> ("error out"=w1405:errorcluster, "S7 Connection out"=w1404:T5)  [unwired: 5 in]
                  }
                }
              }
            }
            n435 = Unbundle By Name(w1382) -> ("status"=w1385:bool)
            n436 = Not(x=w1385) -> (.not. x?=w1384:bool)
            "PLC 7" <- w1384
            n437 = global write "Global 1.vi" "PLC 7"(w1384) -> ()
          }
        }
        n438 = call "PADMINI_STOP_ALL.vi"("Enum"=enum16{"Read", "Write"}."Read") -> ("Boolean 2"=w1225:bool)  [unwired: 9 in, 1 out]
        n439 = local read "stop"() -> (w1224:bool)
        n440 = Or(x=w1224, y=w1225) -> (x .or. y?=w1223:bool)
        n441 = Wait (ms)(milliseconds to wait=u32 1200) -> ()  [unwired: 1 out]
      }
      n442 = call <vilib>:"Clear Errors.vi"() -> ("error out"=w1199:errorcluster)  [unwired: 6 in, 1 out]
      n443 = call <vilib>:"disconnect.vi"("error in (no error)"=w1199, "S7 Connection in"=w1198) -> ()  [unwired: 8 in, 2 out]
    }
    frame Enabled {
      w1411 = PLC_Comm_State."Int"  # Enum
      n444 = while {
        shift-right: [w1423] -> _
        shift-left: w1411 -> [w1431]
        shift-right: [w1415] -> w1408
        shift-left: w1409 -> [w1430]
        shift-right: [w1426] -> _
        shift-left: _ -> [w1429]
        tunnel: w1410 -> [w1412]
        stop <- w1424 stop-if-true
        w1420 = PLC_Comm_State."Disconnect"  # Enum
        w1428 = u32 800  # milliseconds to wait
        # "Int-->Write-->Read---if--Error-->reconnect\n               ^------v                                       v\n                ^------------------------------v"
        # "OP 90-100"
        n445 = case shown="\"Int\"" w1431 {
          selector: w1431 -> [w1447 w1465 w1502 w1548 w1602 w1638 w1651 w1655 _ _]
          tunnel: [w1452 w1467 w1484 w1529 w1578 w1614 w1652 w1660 w1663 w1665] -> w1432
          tunnel: [w1453 w1466 w1483 w1528 w1579 w1615 w1653 w1657 w1662 w1664] -> w1425
          tunnel: w1430 -> [w1450 w1461 w1481 w1531 w1582 w1613 w1649 w1658 w1663 w1665]
          tunnel: w1429 -> [w1448 _ w1482 w1530 w1583 w1612 w1653 w1659 w1662 w1664]
          tunnel: [w1446 w1464 w1501 w1549 w1601 w1639 w1650 w1654 _ _] -> w1427
          tunnel: [_ _ _ _ _ _ _ TRUE _ _] -> w1424
          tunnel: [w1447 w1465 w1502 w1548 w1602 w1638 w1651 w1655 _ _] -> w1421
          tunnel: w1412 -> [w1445 w1463 _ _ _ _ _ _ _ _]
          frame "Connect" {
            w1446 = PLC_Comm_State."Write"  # Enum
            w1458 = TRUE  # Use Rack/Slot for S71200/1500
            w1457 = u8 1  # Slot S7 300/400
            w1455 = u8 0  # Rack S7 300/400
            # "Reconect"
            n446 = call <vilib>:"disconnect.vi"("error in (no error)"=w1450, "S7 Connection in"=w1448) -> ("error out"=w1451:errorcluster)  [unwired: 8 in, 1 out]
            n447 = call <vilib>:"Clear Errors.vi"("error in (no error)"=w1451) -> ("error out"=w1449:errorcluster)  [unwired: 5 in, 1 out]
            n448 = call <vilib>:"connect.vi"("Use Rack/Slot for S71200/1500"=w1458, "Slot S7 300/400"=w1457, "PLC Type"=PLC_Type."S7 1200" ("PLC Type 2"), "error in (no error)"=w1449, "Rack S7 300/400"=w1455, "timeout [ms]"=1000 ("timeout [ms] 2"), "IP address"=w1445) -> ("error out"=w1452:errorcluster, "S7 Connection out"=w1453:T5)  [unwired: 3 in]
          }
          frame "Int" {
            w1464 = PLC_Comm_State."Write"  # Enum
            w1468 = TRUE  # Use Rack/Slot for S71200/1500
            w1469 = u8 1  # Slot S7 300/400
            w1470 = u8 0  # Rack S7 300/400
            # "Initialize and set first bits"
            n449 = call "Stall Data Flow.vim"("value in"=w1461, "milliseconds to wait"=u32 774) -> ("value out"=w1460:errorcluster)  [unwired: 1 out]
            n450 = call <vilib>:"connect.vi"("Use Rack/Slot for S71200/1500"=w1468, "Slot S7 300/400"=w1469, "PLC Type"=PLC_Type."S7 1200" ("PLC Type 2"), "error in (no error)"=w1460, "Rack S7 300/400"=w1470, "timeout [ms]"=1000 ("timeout [ms] 2"), "IP address"=w1463) -> ("error out"=w1472:errorcluster, "S7 Connection out"=w1471:T5)  [unwired: 3 in]
            n451 = for {
              tunnel: u16[] [69, 71] ("Data Block #") -> [w1480] mode=indexing
              shift-right: [w1478] -> w1466
              shift-left: w1471 -> [w1476]
              tunnel: w1472 -> [w1477]
              tunnel: [w1475] -> w1467
              w1479 = i32[] [0, 0]  # DINT input array
              # "Reset Search and save \nbit on software start"
              n452 = call-poly <vilib>:"write DB.vi"("DINT input array"=w1479, "error in (no error)"=w1477, "Data Block #"=w1480, "S7 Connection in"=w1476) -> ("error out"=w1475:errorcluster, "S7 Connection out"=w1478:T5)  [unwired: 4 in, 2 out]
            }
          }
          frame "Write" {
            w1486 = u16 70 ("Data Block #")
            w1501 = PLC_Comm_State."Write2"  # Enum
            # "OP 90 Write"
            n453 = global read "DATA LOG.vi" "OP 90 Outputs"() -> (w1494:bool)
            n454 = case shown="True" w1494 {
              tunnel: [w1513 w1518] -> w1495
              tunnel: [w1514 w1519] -> w1496
              tunnel: w1482 -> [w1514 w1516]
              tunnel: w1481 -> [w1513 w1515]
              frame False {
              }
              frame True {
                w1527 = u16 70  # Data Block #
                n455 = call "PADMINI_AUTO_BARCODE_STATUS 90.vi"("Enum"=enum16{"Read", "Write"}."Read", "error in (no error)"=w1515) -> ("error out"=w1524:errorcluster, "O/P"=w1525:i32[])  [unwired: 8 in]
                n456 = call-poly <vilib>:"write DB.vi"("DINT input array"=w1525, "error in (no error)"=w1524, "Data Block #"=w1527, "S7 Connection in"=w1516) -> ("error out"=w1521:errorcluster, "S7 Connection out"=w1520:T5)  [unwired: 4 in, 2 out]
                n457 = call-poly <vilib>:"write DB.vi"("DINT input array"=i32[] [0] ("Data Byte"), "error in (no error)"=w1521, "Data Block #"=u16 69, "S7 Connection in"=w1520) -> ("error out"=w1518:errorcluster, "S7 Connection out"=w1519:T5)  [unwired: 4 in, 2 out]
                n458 = Unbundle By Name(w1518) -> ("status"=w1517:bool)
                n459 = global write "DATA LOG.vi" "OP 90 Outputs"(w1517) -> ()
              }
            }
            n460 = global read "DATA LOG.vi" "Auto Cycle On"() -> (w1490:bool)
            n461 = global read "DATA LOG.vi" "OP 90 reset"() -> (w1500:bool)
            n462 = Boolean To (0,1)(Boolean=w1490) -> (0, 1=w1489:i16)
            n463 = case shown="True" w1500 {
              tunnel: w1495 -> [w1503 w1509]
              tunnel: w1496 -> [w1504 w1508]
              tunnel: [w1504 w1507] -> w1497
              tunnel: [w1503 w1506] -> w1498
              frame False {
              }
              frame True {
                n464 = call-poly <vilib>:"write DB.vi"("Item offset [byte]"=u16 4 ("Data Block #"), "DINT input array"=i32[] [0], "error in (no error)"=w1509, "Data Block #"=u16 69, "S7 Connection in"=w1508) -> ("error out"=w1506:errorcluster, "S7 Connection out"=w1507:T5)  [unwired: 3 in, 2 out]
                n465 = Unbundle By Name(w1506) -> ("status"=w1505:bool)
                n466 = global write "DATA LOG.vi" "OP 90 reset"(w1505) -> ()
              }
            }
            n467 = Build Array(w1489) -> (w1499:i16[])
            n468 = global read "Global 1.vi" "Filtered BARCODE selected"() -> (w1493:string[])
            n469 = call-poly <vilib>:"write DB.vi"("Item offset [byte]"=u32 20, "DINT input array"=w1499, "error in (no error)"=w1498, "Data Block #"=w1486, "S7 Connection in"=w1497) -> ("error out"=w1492:errorcluster, "S7 Connection out"=w1491:T5)  [unwired: 3 in, 2 out]
            n470 = call-poly <vilib>:"write DB.vi"("Item offset [byte]"=u32 24, "Input STRINGS"=w1493, "error in (no error)"=w1492, "String length reserved in DB (default=254)"=u16 15, "Data Block #"=w1486, "S7 Connection in"=w1491) -> ("error out"=w1484:errorcluster, "S7 Connection out"=w1483:T5)  [unwired: 2 in, 2 out]
          }
          frame "Write2" {
            w1533 = u16 72 ("Data Block #")
            w1549 = PLC_Comm_State."Read"  # Enum
            # "op 100 wirte 2"
            n471 = global read "DATA LOG.vi" "OP 100 Outputs"() -> (w1547:bool)
            n472 = case shown="True" w1547 {
              tunnel: w1530 -> [w1560 w1573]
              tunnel: [w1561 w1563] -> w1545
              tunnel: [w1560 w1566] -> w1546
              tunnel: w1531 -> [w1561 w1570]
              frame False {
              }
              frame True {
                w1574 = u16 72  # Data Block #
                n473 = call "PADMINI_AUTO_BARCODE_STATUS 100.vi"("Enum"=enum16{"Read", "Write"}."Read", "error in (no error)"=w1570) -> ("error out"=w1569:errorcluster, "O/P"=w1571:i32[])  [unwired: 8 in]
                n474 = call-poly <vilib>:"write DB.vi"("DINT input array"=w1571, "error in (no error)"=w1569, "Data Block #"=w1574, "S7 Connection in"=w1573) -> ("error out"=w1565:errorcluster, "S7 Connection out"=w1564:T5)  [unwired: 4 in, 2 out]
                n475 = call-poly <vilib>:"write DB.vi"("DINT input array"=i32[] [0] ("Data Byte"), "error in (no error)"=w1565, "Data Block #"=u16 71, "S7 Connection in"=w1564) -> ("error out"=w1563:errorcluster, "S7 Connection out"=w1566:T5)  [unwired: 4 in, 2 out]
                n476 = Unbundle By Name(w1563) -> ("status"=w1562:bool)
                n477 = global write "DATA LOG.vi" "OP 100 Outputs"(w1562) -> ()
              }
            }
            n478 = global read "DATA LOG.vi" "OP 100 reset"() -> (w1544:bool)
            n479 = case shown="True" w1544 {
              tunnel: w1545 -> [w1550 w1559]
              tunnel: [w1550 w1553] -> w1540
              tunnel: w1546 -> [w1551 w1558]
              tunnel: [w1551 w1557] -> w1539
              frame False {
              }
              frame True {
                n480 = call-poly <vilib>:"write DB.vi"("Item offset [byte]"=u16 4 ("Data Block #"), "DINT input array"=i32[] [0], "error in (no error)"=w1559, "Data Block #"=u16 71, "S7 Connection in"=w1558) -> ("error out"=w1553:errorcluster, "S7 Connection out"=w1557:T5)  [unwired: 3 in, 2 out]
                n481 = Unbundle By Name(w1553) -> ("status"=w1552:bool)
                n482 = global write "DATA LOG.vi" "OP 100 reset"(w1552) -> ()
              }
            }
            n483 = global read "DATA LOG.vi" "Auto Cycle On"() -> (w1538:bool)
            n484 = global read "Global 1.vi" "Filtered BARCODE selected"() -> (w1541:string[])
            n485 = Boolean To (0,1)(Boolean=w1538) -> (0, 1=w1537:i16)
            n486 = Build Array(w1537) -> (w1536:i16[])
            n487 = call-poly <vilib>:"write DB.vi"("Item offset [byte]"=u32 20, "DINT input array"=w1536, "error in (no error)"=w1540, "Data Block #"=w1533, "S7 Connection in"=w1539) -> ("error out"=w1542:errorcluster, "S7 Connection out"=w1543:T5)  [unwired: 3 in, 2 out]
            n488 = call-poly <vilib>:"write DB.vi"("Item offset [byte]"=u32 24, "Input STRINGS"=w1541, "error in (no error)"=w1542, "String length reserved in DB (default=254)"=u16 15, "Data Block #"=w1533, "S7 Connection in"=w1543) -> ("error out"=w1529:errorcluster, "S7 Connection out"=w1528:T5)  [unwired: 2 in, 2 out]
          }
          frame "Read" {
            w1592 = u16 69 ("Data Block #")
            w1601 = PLC_Comm_State."Read2"  # Enum
            # "OP90 read"
            n489 = call-poly <vilib>:"read DB.vi"("Item offset [byte]"=u32 8, "error in (no error)"=w1582, "items #"=u16 2 ("Items # [byte]"), "Data Block #"=w1592, "S7 Connection in"=w1583) -> ("error out"=w1599:errorcluster, "REAL result array"=w1575:sgl[], "S7 Connection out"=w1600:T5)  [unwired: 4 in]
            n490 = call-poly <vilib>:"read DB.vi"("Item offset [byte]"=u32 16, "String length reserved in DB (default=254)"=u16 50, "error in (no error)"=w1599, "items #"=u16 1 ("Items # [byte]"), "Data Block #"=w1592, "S7 Connection in"=w1600) -> ("error out"=w1598:errorcluster, "STRING result Array"=w1596:string[], "S7 Connection out"=w1597:T5)  [unwired: 2 in, 1 out]
            n491 = call-poly <vilib>:"read DB.vi"("Item offset [byte]"=u32 68, "String length reserved in DB (default=254)"=u16 10, "error in (no error)"=w1598, "items #"=u16 3 ("Items # [byte]"), "Data Block #"=w1592, "S7 Connection in"=w1597) -> ("error out"=w1576:errorcluster, "STRING result Array"=w1595:string[], "S7 Connection out"=w1594:T5)  [unwired: 2 in, 1 out]
            n492 = Build Array (concatenate)(w1596, w1595) -> (w1581:string[])
            n493 = call-poly <vilib>:"read DB.vi"("error in (no error)"=w1576, "items #"=u16 2 ("Items # [byte]"), "Data Block #"=w1592, "S7 Connection in"=w1594) -> ("error out"=w1577:errorcluster, "DINT result array"=w1580:i32[], "S7 Connection out"=w1579:T5)  [unwired: 5 in]
            n494 = case shown="No Error" w1577 {
              selector: w1577 -> [w1605 w1611]
              tunnel: w1580 -> [w1610 _]
              tunnel: w1581 -> [w1609 _]
              tunnel: [w1604 w1611] -> w1578
              tunnel: w1575 -> [w1603 _]
              frame No Error {
                w1608 = enum16{"Read", "Write"}."Write" ("Enum")
                n495 = call "PADMINI_AUTO_CYCLE VALUE 90.vi"("Enum"=w1608, "error in (no error)"=w1605, "Input"=w1603) -> ("error out"=w1607:errorcluster)  [unwired: 7 in, 1 out]
                n496 = call "PADMINI_AUTO_BARCODE_STRING 90.vi"("Enum"=w1608, "error in (no error)"=w1607, "Input"=w1609) -> ("error out"=w1606:errorcluster)  [unwired: 7 in, 1 out]
                n497 = call "PADMINI_AUTO_CYCLE STATE 90.vi"("Enum"=w1608, "error in (no error)"=w1606, "Input"=w1610) -> ("error out"=w1604:errorcluster)  [unwired: 7 in, 1 out]
              }
              frame Error {
              }
            }
          }
          frame "Read2" {
            w1624 = u16 71 ("Data Block #")
            w1639 = PLC_Comm_State."Write"  # Enum
            # "Op100 Read2"
            n498 = call-poly <vilib>:"read DB.vi"("Item offset [byte]"=u32 8, "error in (no error)"=w1613, "items #"=u16 11 ("Items # [byte]"), "Data Block #"=w1624, "S7 Connection in"=w1612) -> ("error out"=w1635:errorcluster, "REAL result array"=w1637:sgl[], "S7 Connection out"=w1634:T5)  [unwired: 4 in]
            n499 = call-poly <vilib>:"read DB.vi"("Item offset [byte]"=u32 52, "String length reserved in DB (default=254)"=u16 50, "error in (no error)"=w1635, "items #"=u16 1 ("Items # [byte]"), "Data Block #"=w1624, "S7 Connection in"=w1634) -> ("error out"=w1632:errorcluster, "STRING result Array"=w1630:string[], "S7 Connection out"=w1631:T5)  [unwired: 2 in, 1 out]
            n500 = call-poly <vilib>:"read DB.vi"("Item offset [byte]"=u32 104, "String length reserved in DB (default=254)"=u16 10, "error in (no error)"=w1632, "items #"=u16 2 ("Items # [byte]"), "Data Block #"=w1624, "S7 Connection in"=w1631) -> ("error out"=w1633:errorcluster, "STRING result Array"=w1629:string[], "S7 Connection out"=w1626:T5)  [unwired: 2 in, 1 out]
            n501 = Build Array (concatenate)(w1630, w1629) -> (w1636:string[])
            n502 = call-poly <vilib>:"read DB.vi"("error in (no error)"=w1633, "items #"=u16 2 ("Items # [byte]"), "Data Block #"=w1624, "S7 Connection in"=w1626) -> ("error out"=w1627:errorcluster, "DINT result array"=w1628:i32[], "S7 Connection out"=w1615:T5)  [unwired: 5 in]
            n503 = case shown="No Error" w1627 {
              selector: w1627 -> [w1644 w1648]
              tunnel: w1628 -> [w1647 _]
              tunnel: w1636 -> [w1642 _]
              tunnel: w1637 -> [w1641 _]
              tunnel: [w1640 w1648] -> w1614
              frame No Error {
                w1643 = enum16{"Read", "Write"}."Write" ("Enum")
                n504 = call "PADMINI_AUTO_CYCLE VALUE 100.vi"("Enum"=w1643, "error in (no error)"=w1644, "Input"=w1641) -> ("error out"=w1645:errorcluster)  [unwired: 7 in, 1 out]
                n505 = call "PADMINI_AUTO_BARCODE_STRING 100.vi"("Enum"=w1643, "error in (no error)"=w1645, "Input"=w1642) -> ("error out"=w1646:errorcluster)  [unwired: 7 in, 1 out]
                n506 = call "PADMINI_AUTO_CYCLE STATE 100.vi"("Enum"=w1643, "error in (no error)"=w1646, "Input"=w1647) -> ("error out"=w1640:errorcluster)  [unwired: 7 in, 1 out]
              }
              frame Error {
              }
            }
          }
          frame "Error" {
            w1650 = PLC_Comm_State."Connect"  # Enum
            n507 = global write "Global 1.vi" "PLC7 error"(w1649) -> ()
            n508 = call <vilib>:"Clear Errors.vi"("error in (no error)"=w1649) -> ("error out"=w1652:errorcluster)  [unwired: 5 in, 1 out]
          }
          frame "Disconnect" {
            w1654 = PLC_Comm_State."Disconnect"  # Enum
            w1657 = T5 {"TCP Connection Ref"=refnum, "IP address"="", "timeout ms"=5000, "Connected?"=FALSE, "PLC Type"=enum."S7 1200", "Rack S7 400"=0, "Slot S7 400"=0, "PDU Size"=0, "connection semaphore"=refnum}  # S7 Connection out
            n509 = call <vilib>:"Clear Errors.vi"("error in (no error)"=w1658) -> ("error out"=w1661:errorcluster)  [unwired: 5 in, 1 out]
            n510 = call <vilib>:"disconnect.vi"("error in (no error)"=w1661, "S7 Connection in"=w1659) -> ("error out"=w1660:errorcluster)  [unwired: 8 in, 1 out]
          }
          frame "Write3" {
            # "No Use"
          }
          frame "Read3" {
            # "No Use"
          }
        }
        n511 = Wait (ms)(milliseconds to wait=w1428) -> ()  [unwired: 1 out]
        n512 = call "PADMINI_STOP_ALL.vi"("Enum"=enum16{"Read", "Write"}."Read") -> ("Boolean 2"=w1419:bool)  [unwired: 9 in, 1 out]
        n513 = local read "stop"() -> (w1414:bool)
        n514 = case shown="Error" w1432 {
          selector: w1432 -> [w1435 w1438]
          tunnel: [w1435 w1437] -> w1415
          tunnel: [w1434 w1436] -> w1422
          tunnel: w1427 -> [w1434 _]
          tunnel: [w1433 w1444] -> w1426
          tunnel: w1425 -> [w1433 w1444]
          tunnel: w1421 -> [_ w1442]
          frame No Error {
          }
          frame Error {
            w1436 = PLC_Comm_State."Error"  # Enum
            n515 = Unbundle By Name(w1438) -> ("source"=w1443:string)
            n516 = call <userlib>:"Get Strings from Enum__ogtk.vi"("Enum"=w1442) -> ("String Value"=w1441:string)  [unwired: 7 in, 3 out]
            n517 = Concatenate Strings(w1441, "    " ("string"), w1443) -> (w1439:string)
            n518 = Bundle By Name(cluster=w1438, "source"=w1439) -> (w1437:errorcluster)
          }
        }
        n519 = Or(x=w1414, y=w1419) -> (x .or. y?=w1417:bool)
        n520 = Select(t=w1420, s=w1417, f=w1422) -> (s? t:f=w1423:T1)
        n521 = Unbundle By Name(w1415) -> ("status"=w1416:bool)
        n522 = Not(x=w1416) -> (.not. x?=w1413:bool)
        n523 = global write "Global 1.vi" "PLC 7"(w1413) -> ()
      }
    }
  }
  n524 = disable-structure shown="Enabled" {
    disable-tunnel: w71 -> [w1678 w1803]
    disable-tunnel: w9 -> [w1671 w1802]
    disable-tunnel: [w1666 w1801] -> w4
    frame Disabled {
      w1668 = TRUE  # Use Rack/Slot for S71200/1500
      w1669 = u8 1  # Slot S7 300/400
      w1670 = u8 0  # Rack S7 300/400
      w1677 = i32[] [0, 0]  # DINT input array
      # "Reset Search and save \nbit on software start"
      n525 = call <vilib>:"connect.vi"("Use Rack/Slot for S71200/1500"=w1668, "Slot S7 300/400"=w1669, "PLC Type"=PLC_Type."S7 1200" ("PLC Type 2"), "error in (no error)"=w1671, "Rack S7 300/400"=w1670, "timeout [ms]"=1000 ("timeout [ms] 2"), "IP address"=w1678) -> ("error out"=w1673:errorcluster, "S7 Connection out"=w1672:T5)  [unwired: 3 in]
      n526 = call-poly <vilib>:"write DB.vi"("DINT input array"=w1677, "error in (no error)"=w1673, "Data Block #"=u16 56, "S7 Connection in"=w1672) -> ("error out"=w1674:errorcluster, "S7 Connection out"=w1675:T5)  [unwired: 4 in, 2 out]
      n527 = while {
        shift-right: [w1685] -> w1682
        shift-left: w1675 -> [w1695]
        shift-right: [w1693] -> w1681
        shift-left: w1674 -> [w1694]
        tunnel: w1678 -> [w1684]
        stop <- w1687 stop-if-true
        # "OP 50"
        n528 = flat-sequence {
          tunnel: [w1698] -> w1691
          tunnel: [w1696] -> w1686
          tunnel: w1694 -> [w1746]
          tunnel: w1695 -> [w1745]
          tunnel: w1684 -> [w1733]
          tunnel: [w1733] -> w1683
          tunnel: [w1774] -> w1693
          tunnel: [w1773] -> w1685
          tunnel: w1691 -> [w1776]
          tunnel: w1686 -> [w1775]
          tunnel: w1683 -> [w1772]
          frame #0 {
            w1716 = u16 57 ("Data Block #")
            w1724 = u16 56 ("Data Block #")
            # "AUTO WRITE"
            n529 = global read "DATA LOG.vi" "OP 50 Outputs"() -> (w1744:bool)
            n530 = case shown="True" w1744 {
              tunnel: w1745 -> [w1757 w1770]
              tunnel: [w1758 w1759] -> w1732
              tunnel: [w1757 w1762] -> w1731
              tunnel: w1746 -> [w1758 w1767]
              frame False {
              }
              frame True {
                w1771 = u16 57  # Data Block #
                n531 = call "PADMINI_AUTO_BARCODE_STATUS 50.vi"("Enum"=enum16{"Read", "Write"}."Read", "error in (no error)"=w1767) -> ("error out"=w1766:errorcluster, "O/P"=w1768:i32[])  [unwired: 8 in]
                n532 = global write "DATA LOG.vi" "OP 50 Outputs"(FALSE) -> ()
                n533 = call-poly <vilib>:"write DB.vi"("DINT input array"=w1768, "error in (no error)"=w1766, "Data Block #"=w1771, "S7 Connection in"=w1770) -> ("error out"=w1760:errorcluster, "S7 Connection out"=w1761:T5)  [unwired: 4 in, 2 out]
                n534 = call-poly <vilib>:"write DB.vi"("DINT input array"=i32[] [0] ("Data Byte"), "error in (no error)"=w1760, "Data Block #"=u16 56, "S7 Connection in"=w1761) -> ("error out"=w1759:errorcluster, "S7 Connection out"=w1762:T5)  [unwired: 4 in, 2 out]
              }
            }
            n535 = global read "DATA LOG.vi" "OP 50 reset"() -> (w1730:bool)
            n536 = global read "DATA LOG.vi" "Auto Cycle On"() -> (w1707:bool)
            n537 = case shown="True" w1730 {
              tunnel: w1732 -> [w1747 w1756]
              tunnel: [w1747 w1755] -> w1709
              tunnel: w1731 -> [w1748 w1754]
              tunnel: [w1748 w1753] -> w1712
              frame False {
              }
              frame True {
                n538 = global write "DATA LOG.vi" "OP 50 reset"(FALSE) -> ()
                n539 = call-poly <vilib>:"write DB.vi"("Item offset [byte]"=u16 4 ("Data Block #"), "DINT input array"=i32[] [0], "error in (no error)"=w1756, "Data Block #"=u16 56, "S7 Connection in"=w1754) -> ("error out"=w1755:errorcluster, "S7 Connection out"=w1753:T5)  [unwired: 3 in, 2 out]
              }
            }
            n540 = Boolean To (0,1)(Boolean=w1707) -> (0, 1=w1706:i16)
            n541 = Build Array(w1706) -> (w1705:i16[])
            n542 = global read "Global 1.vi" "Filtered BARCODE selected"() -> (w1713:string[])
            n543 = call-poly <vilib>:"write DB.vi"("Item offset [byte]"=u32 20, "DINT input array"=w1705, "error in (no error)"=w1709, "Data Block #"=w1716, "S7 Connection in"=w1712) -> ("error out"=w1718:errorcluster, "S7 Connection out"=w1719:T5)  [unwired: 3 in, 2 out]
            n544 = call-poly <vilib>:"write DB.vi"("Item offset [byte]"=u32 24, "Input STRINGS"=w1713, "error in (no error)"=w1718, "String length reserved in DB (default=254)"=u16 15, "Data Block #"=w1716, "S7 Connection in"=w1719) -> ("error out"=w1710:errorcluster, "S7 Connection out"=w1711:T5)  [unwired: 2 in, 2 out]
            n545 = call-poly <vilib>:"read DB.vi"("Item offset [byte]"=u32 8, "error in (no error)"=w1710, "items #"=u16 3 ("Items # [byte]"), "Data Block #"=w1724, "S7 Connection in"=w1711) -> ("error out"=w1736:errorcluster, "REAL result array"=w1734:sgl[], "S7 Connection out"=w1742:T5)  [unwired: 4 in]
            n546 = call "PADMINI_AUTO_CYCLE VALUE 50.vi"("Enum"=enum16{"Read", "Write"}."Write", "error in (no error)"=w1736, "Input"=w1734) -> ("error out"=w1735:errorcluster)  [unwired: 7 in, 1 out]
            n547 = call-poly <vilib>:"read DB.vi"("Item offset [byte]"=u32 20, "String length reserved in DB (default=254)"=u16 50, "error in (no error)"=w1735, "items #"=u16 1 ("Items # [byte]"), "Data Block #"=w1724, "S7 Connection in"=w1742) -> ("error out"=w1726:errorcluster, "STRING result Array"=w1723:string[], "S7 Connection out"=w1725:T5)  [unwired: 2 in, 1 out]
            n548 = call-poly <vilib>:"read DB.vi"("Item offset [byte]"=u32 72, "String length reserved in DB (default=254)"=u16 10, "error in (no error)"=w1726, "items #"=u16 5 ("Items # [byte]"), "Data Block #"=w1724, "S7 Connection in"=w1725) -> ("error out"=w1727:errorcluster, "STRING result Array"=w1722:string[], "S7 Connection out"=w1699:T5)  [unwired: 2 in, 1 out]
            n549 = Build Array (concatenate)(w1723, w1722) -> (w1721:string[])
            n550 = call "PADMINI_AUTO_BARCODE_STRING 50.vi"("Enum"=enum16{"Read", "Write"}."Write", "error in (no error)"=w1727, "Input"=w1721) -> ("error out"=w1697:errorcluster)  [unwired: 7 in, 1 out]
            n551 = call-poly <vilib>:"read DB.vi"("error in (no error)"=w1697, "items #"=u16 2 ("Items # [byte]"), "Data Block #"=u16 56, "S7 Connection in"=w1699) -> ("error out"=w1701:errorcluster, "DINT result array"=w1703:i32[], "S7 Connection out"=w1698:T5)  [unwired: 5 in]
            n552 = call "PADMINI_AUTO_CYCLE STATE 50.vi"("Enum"=enum16{"Read", "Write"}."Write", "error in (no error)"=w1701, "Input"=w1703) -> ("error out"=w1696:errorcluster)  [unwired: 7 in, 1 out]
          }
          frame #1 {
            # "RECONNECT"
            n553 = case shown="Error" w1775 {
              selector: w1775 -> [w1780 w1781]
              tunnel: [w1779 w1785] -> w1773
              tunnel: [w1780 w1786] -> w1774
              tunnel: w1776 -> [w1779 w1784]
              tunnel: w1772 -> [_ w1783]
              frame No Error {
              }
              frame Error {
                n554 = Unbundle By Name(w1781) -> ("code"=w1782:i32)
                n555 = call <vilib>:"Clear Errors.vi"("error in (no error)"=w1781) -> ("error out"=w1787:errorcluster)  [unwired: 5 in, 1 out]
                n556 = case shown="1, 66" w1782 {
                  tunnel: w1787 -> [w1789 w1800]
                  tunnel: [w1789 w1798] -> w1786
                  tunnel: [w1790 w1797] -> w1785
                  tunnel: w1784 -> [w1790 w1794]
                  tunnel: w1783 -> [_ w1793]
                  tunnel: w1781 -> [w1788 _]
                  frame 0, Default {
                    n557 = global write "Global 1.vi" "PLC4 error"(w1788) -> ()
                  }
                  frame 1, 66 {
                    n558 = call <vilib>:"disconnect.vi"("error in (no error)"=w1800, "S7 Connection in"=w1794) -> ("error out"=w1799:errorcluster)  [unwired: 8 in, 1 out]
                    n559 = call <vilib>:"Clear Errors.vi"("error in (no error)"=w1799) -> ("error out"=w1796:errorcluster)  [unwired: 5 in, 1 out]
                    n560 = call <vilib>:"connect.vi"("Use Rack/Slot for S71200/1500"=TRUE, "Slot S7 300/400"=u8 1, "PLC Type"=PLC_Type."S7 1200" ("PLC Type 2"), "error in (no error)"=w1796, "IP address"=w1793) -> ("error out"=w1798:errorcluster, "S7 Connection out"=w1797:T5)  [unwired: 5 in]
                  }
                }
              }
            }
            n561 = Unbundle By Name(w1775) -> ("status"=w1778:bool)
            n562 = Not(x=w1778) -> (.not. x?=w1777:bool)
            "PLC 4" <- w1777
            n563 = global write "Global 1.vi" "PLC 4"(w1777) -> ()
          }
        }
        n564 = call "PADMINI_STOP_ALL.vi"("Enum"=enum16{"Read", "Write"}."Read") -> ("Boolean 2"=w1689:bool)  [unwired: 9 in, 1 out]
        n565 = local read "stop"() -> (w1688:bool)
        n566 = Or(x=w1688, y=w1689) -> (x .or. y?=w1687:bool)
        n567 = Wait (ms)(milliseconds to wait=u32 1200) -> ()  [unwired: 1 out]
      }
      n568 = call <vilib>:"Clear Errors.vi"("error in (no error)"=w1681) -> ("error out"=w1667:errorcluster)  [unwired: 5 in, 1 out]
      n569 = call <vilib>:"disconnect.vi"("error in (no error)"=w1667, "S7 Connection in"=w1682) -> ("error out"=w1666:errorcluster)  [unwired: 8 in, 1 out]
    }
    frame Enabled {
      w1804 = PLC_Comm_State."Int"  # Enum
      n570 = while {
        shift-right: [w1816] -> _
        shift-left: w1804 -> [w1824]
        shift-right: [w1808] -> w1801
        shift-left: w1802 -> [w1823]
        shift-right: [w1819] -> _
        shift-left: _ -> [w1822]
        tunnel: w1803 -> [w1805]
        stop <- w1817 stop-if-true
        w1813 = PLC_Comm_State."Disconnect"  # Enum
        w1821 = u32 800  # milliseconds to wait
        # "Int-->Write-->Read---if--Error-->reconnect\n               ^------v                                       v\n                ^------------------------------v"
        # "OP 50"
        n571 = case shown="\"Int\"" w1824 {
          selector: w1824 -> [w1840 w1857 w1895 w1948 w1960 w1964 _ _ _ _]
          tunnel: [w1845 w1859 w1875 w1923 w1961 w1969 w1971 w1974 w1976 w1978] -> w1825
          tunnel: [w1846 w1858 w1874 w1922 w1962 w1966 w1972 w1973 w1975 w1977] -> w1818
          tunnel: w1823 -> [w1843 w1853 w1876 w1924 w1958 w1967 w1971 w1974 w1976 w1978]
          tunnel: w1822 -> [w1841 _ w1877 w1921 w1962 w1968 w1972 w1973 w1975 w1977]
          tunnel: [w1839 w1856 w1894 w1947 w1959 w1963 _ _ _ _] -> w1820
          tunnel: [_ _ _ _ _ TRUE _ _ _ _] -> w1817
          tunnel: [w1840 w1857 w1895 w1948 w1960 w1964 _ _ _ _] -> w1814
          tunnel: w1805 -> [w1838 w1855 _ _ _ _ _ _ _ _]
          frame "Connect" {
            w1839 = PLC_Comm_State."Write"  # Enum
            w1851 = TRUE  # Use Rack/Slot for S71200/1500
            w1850 = u8 1  # Slot S7 300/400
            w1848 = u8 0  # Rack S7 300/400
            # "Reconect"
            n572 = call <vilib>:"disconnect.vi"("error in (no error)"=w1843, "S7 Connection in"=w1841) -> ("error out"=w1844:errorcluster)  [unwired: 8 in, 1 out]
            n573 = call <vilib>:"Clear Errors.vi"("error in (no error)"=w1844) -> ("error out"=w1842:errorcluster)  [unwired: 5 in, 1 out]
            n574 = call <vilib>:"connect.vi"("Use Rack/Slot for S71200/1500"=w1851, "Slot S7 300/400"=w1850, "PLC Type"=PLC_Type."S7 1200" ("PLC Type 2"), "error in (no error)"=w1842, "Rack S7 300/400"=w1848, "timeout [ms]"=1000 ("timeout [ms] 2"), "IP address"=w1838) -> ("error out"=w1845:errorcluster, "S7 Connection out"=w1846:T5)  [unwired: 3 in]
          }
          frame "Int" {
            w1856 = PLC_Comm_State."Write"  # Enum
            w1860 = TRUE  # Use Rack/Slot for S71200/1500
            w1861 = u8 1  # Slot S7 300/400
            w1862 = u8 0  # Rack S7 300/400
            w1863 = u16[] [56]  # Data Block #
            # "Initialize and set first bits"
            n575 = call "Stall Data Flow.vim"("value in"=w1853, "milliseconds to wait"=u32 387) -> ("value out"=w1852:errorcluster)  [unwired: 1 out]
            n576 = call <vilib>:"connect.vi"("Use Rack/Slot for S71200/1500"=w1860, "Slot S7 300/400"=w1861, "PLC Type"=PLC_Type."S7 1200" ("PLC Type 2"), "error in (no error)"=w1852, "Rack S7 300/400"=w1862, "timeout [ms]"=1000 ("timeout [ms] 2"), "IP address"=w1855) -> ("error out"=w1865:errorcluster, "S7 Connection out"=w1864:T5)  [unwired: 3 in]
            n577 = for {
              tunnel: w1863 -> [w1873] mode=indexing
              shift-right: [w1871] -> w1858
              shift-left: w1864 -> [w1869]
              tunnel: w1865 -> [w1870]
              tunnel: [w1868] -> w1859
              w1872 = i32[] [0, 0]  # DINT input array
              # "Reset Search and save \nbit on software start"
              n578 = call-poly <vilib>:"write DB.vi"("DINT input array"=w1872, "error in (no error)"=w1870, "Data Block #"=w1873, "S7 Connection in"=w1869) -> ("error out"=w1868:errorcluster, "S7 Connection out"=w1871:T5)  [unwired: 4 in, 2 out]
            }
          }
          frame "Write" {
            w1879 = u16 57 ("Data Block #")
            w1894 = PLC_Comm_State."Read"  # Enum
            n579 = global read "DATA LOG.vi" "OP 50 Outputs"() -> (w1893:bool)
            n580 = case shown="True" w1893 {
              tunnel: w1877 -> [w1906 w1919]
              tunnel: [w1907 w1909] -> w1892
              tunnel: [w1906 w1912] -> w1891
              tunnel: w1876 -> [w1907 w1916]
              frame False {
              }
              frame True {
                w1920 = u16 57  # Data Block #
                n581 = call "PADMINI_AUTO_BARCODE_STATUS 50.vi"("Enum"=enum16{"Read", "Write"}."Read", "error in (no error)"=w1916) -> ("error out"=w1915:errorcluster, "O/P"=w1917:i32[])  [unwired: 8 in]
                n582 = call-poly <vilib>:"write DB.vi"("DINT input array"=w1917, "error in (no error)"=w1915, "Data Block #"=w1920, "S7 Connection in"=w1919) -> ("error out"=w1910:errorcluster, "S7 Connection out"=w1911:T5)  [unwired: 4 in, 2 out]
                n583 = call-poly <vilib>:"write DB.vi"("DINT input array"=i32[] [0] ("Data Byte"), "error in (no error)"=w1910, "Data Block #"=u16 56, "S7 Connection in"=w1911) -> ("error out"=w1909:errorcluster, "S7 Connection out"=w1912:T5)  [unwired: 4 in, 2 out]
                n584 = Unbundle By Name(w1909) -> ("status"=w1908:bool)
                n585 = global write "DATA LOG.vi" "OP 50 Outputs"(w1908) -> ()
              }
            }
            n586 = global read "DATA LOG.vi" "OP 50 reset"() -> (w1890:bool)
            n587 = case shown="True" w1890 {
              tunnel: w1892 -> [w1896 w1905]
              tunnel: [w1896 w1899] -> w1885
              tunnel: w1891 -> [w1897 w1904]
              tunnel: [w1897 w1903] -> w1886
              frame False {
              }
              frame True {
                n588 = call-poly <vilib>:"write DB.vi"("Item offset [byte]"=u16 4 ("Data Block #"), "DINT input array"=i32[] [0], "error in (no error)"=w1905, "Data Block #"=u16 56, "S7 Connection in"=w1904) -> ("error out"=w1899:errorcluster, "S7 Connection out"=w1903:T5)  [unwired: 3 in, 2 out]
                n589 = Unbundle By Name(w1899) -> ("status"=w1898:bool)
                n590 = global write "DATA LOG.vi" "OP 50 reset"(w1898) -> ()
              }
            }
            n591 = global read "DATA LOG.vi" "Auto Cycle On"() -> (w1884:bool)
            n592 = global read "Global 1.vi" "Filtered BARCODE selected"() -> (w1887:string[])
            n593 = Boolean To (0,1)(Boolean=w1884) -> (0, 1=w1883:i16)
            n594 = Build Array(w1883) -> (w1882:i16[])
            n595 = call-poly <vilib>:"write DB.vi"("Item offset [byte]"=u32 20, "DINT input array"=w1882, "error in (no error)"=w1885, "Data Block #"=w1879, "S7 Connection in"=w1886) -> ("error out"=w1888:errorcluster, "S7 Connection out"=w1889:T5)  [unwired: 3 in, 2 out]
            n596 = call-poly <vilib>:"write DB.vi"("Item offset [byte]"=u32 24, "Input STRINGS"=w1887, "error in (no error)"=w1888, "String length reserved in DB (default=254)"=u16 15, "Data Block #"=w1879, "S7 Connection in"=w1889) -> ("error out"=w1875:errorcluster, "S7 Connection out"=w1874:T5)  [unwired: 2 in, 2 out]
          }
          frame "Read" {
            w1933 = u16 56 ("Data Block #")
            w1947 = PLC_Comm_State."Write"  # Enum
            # "OP 50 Read"
            n597 = call-poly <vilib>:"read DB.vi"("error in (no error)"=w1924, "items #"=u16 2 ("Items # [byte]"), "Data Block #"=w1933, "S7 Connection in"=w1921) -> ("error out"=w1945:errorcluster, "DINT result array"=w1941:i32[], "S7 Connection out"=w1944:T5)  [unwired: 5 in]
            n598 = call-poly <vilib>:"read DB.vi"("Item offset [byte]"=u32 8, "error in (no error)"=w1945, "items #"=u16 3 ("Items # [byte]"), "Data Block #"=w1933, "S7 Connection in"=w1944) -> ("error out"=w1939:errorcluster, "REAL result array"=w1943:sgl[], "S7 Connection out"=w1940:T5)  [unwired: 4 in]
            n599 = call-poly <vilib>:"read DB.vi"("Item offset [byte]"=u32 20, "String length reserved in DB (default=254)"=u16 50, "error in (no error)"=w1939, "items #"=u16 1 ("Items # [byte]"), "Data Block #"=w1933, "S7 Connection in"=w1940) -> ("error out"=w1938:errorcluster, "STRING result Array"=w1936:string[], "S7 Connection out"=w1937:T5)  [unwired: 2 in, 1 out]
            n600 = call-poly <vilib>:"read DB.vi"("Item offset [byte]"=u32 72, "String length reserved in DB (default=254)"=u16 10, "error in (no error)"=w1938, "items #"=u16 5 ("Items # [byte]"), "Data Block #"=w1933, "S7 Connection in"=w1937) -> ("error out"=w1946:errorcluster, "STRING result Array"=w1935:string[], "S7 Connection out"=w1922:T5)  [unwired: 2 in, 1 out]
            n601 = Build Array (concatenate)(w1936, w1935) -> (w1942:string[])
            n602 = case shown="No Error" w1946 {
              selector: w1946 -> [w1952 w1957]
              tunnel: w1941 -> [w1956 _]
              tunnel: w1942 -> [w1954 _]
              tunnel: w1943 -> [w1951 _]
              tunnel: [w1950 w1957] -> w1923
              frame No Error {
                w1949 = enum16{"Read", "Write"}."Write" ("Enum")
                n603 = call "PADMINI_AUTO_CYCLE VALUE 50.vi"("Enum"=w1949, "error in (no error)"=w1952, "Input"=w1951) -> ("error out"=w1953:errorcluster)  [unwired: 7 in, 1 out]
                n604 = call "PADMINI_AUTO_BARCODE_STRING 50.vi"("Enum"=w1949, "error in (no error)"=w1953, "Input"=w1954) -> ("error out"=w1955:errorcluster)  [unwired: 7 in, 1 out]
                n605 = call "PADMINI_AUTO_CYCLE STATE 50.vi"("Enum"=w1949, "error in (no error)"=w1955, "Input"=w1956) -> ("error out"=w1950:errorcluster)  [unwired: 7 in, 1 out]
              }
              frame Error {
              }
            }
          }
          frame "Error" {
            w1959 = PLC_Comm_State."Connect"  # Enum
            n606 = global write "Global 1.vi" "PLC4 error"(w1958) -> ()
            n607 = call <vilib>:"Clear Errors.vi"("error in (no error)"=w1958) -> ("error out"=w1961:errorcluster)  [unwired: 5 in, 1 out]
          }
          frame "Disconnect" {
            w1963 = PLC_Comm_State."Disconnect"  # Enum
            w1966 = T5 {"TCP Connection Ref"=refnum, "IP address"="", "timeout ms"=5000, "Connected?"=FALSE, "PLC Type"=enum."S7 1200", "Rack S7 400"=0, "Slot S7 400"=0, "PDU Size"=0, "connection semaphore"=refnum}  # S7 Connection out
            n608 = call <vilib>:"Clear Errors.vi"("error in (no error)"=w1967) -> ("error out"=w1970:errorcluster)  [unwired: 5 in, 1 out]
            n609 = call <vilib>:"disconnect.vi"("error in (no error)"=w1970, "S7 Connection in"=w1968) -> ("error out"=w1969:errorcluster)  [unwired: 8 in, 1 out]
          }
          frame "Write2" {
            # "No Use"
          }
          frame "Write3" {
            # "No Use"
          }
          frame "Read2" {
            # "No Use"
          }
          frame "Read3" {
            # "No Use"
          }
        }
        n610 = Wait (ms)(milliseconds to wait=w1821) -> ()  [unwired: 1 out]
        n611 = call "PADMINI_STOP_ALL.vi"("Enum"=enum16{"Read", "Write"}."Read") -> ("Boolean 2"=w1812:bool)  [unwired: 9 in, 1 out]
        n612 = local read "stop"() -> (w1807:bool)
        n613 = case shown="Error" w1825 {
          selector: w1825 -> [w1828 w1831]
          tunnel: [w1828 w1830] -> w1808
          tunnel: [w1827 w1829] -> w1815
          tunnel: w1820 -> [w1827 _]
          tunnel: [w1826 w1837] -> w1819
          tunnel: w1818 -> [w1826 w1837]
          tunnel: w1814 -> [_ w1835]
          frame No Error {
          }
          frame Error {
            w1829 = PLC_Comm_State."Error"  # Enum
            n614 = Unbundle By Name(w1831) -> ("source"=w1836:string)
            n615 = call <userlib>:"Get Strings from Enum__ogtk.vi"("Enum"=w1835) -> ("String Value"=w1834:string)  [unwired: 7 in, 3 out]
            n616 = Concatenate Strings(w1834, "    " ("string"), w1836) -> (w1832:string)
            n617 = Bundle By Name(cluster=w1831, "source"=w1832) -> (w1830:errorcluster)
          }
        }
        n618 = Or(x=w1807, y=w1812) -> (x .or. y?=w1810:bool)
        n619 = Select(t=w1813, s=w1810, f=w1815) -> (s? t:f=w1816:T1)
        n620 = Unbundle By Name(w1808) -> ("status"=w1809:bool)
        n621 = Not(x=w1809) -> (.not. x?=w1806:bool)
        n622 = global write "Global 1.vi" "PLC 4"(w1806) -> ()
      }
    }
  }
  n623 = disable-structure shown="Enabled" {
    disable-tunnel: w61 -> [w1991 w2116]
    disable-tunnel: w9 -> [w1984 w2115]
    disable-tunnel: [w1979 w2114] -> w6
    frame Disabled {
      w1981 = TRUE  # Use Rack/Slot for S71200/1500
      w1982 = u8 1  # Slot S7 300/400
      w1983 = u8 0  # Rack S7 300/400
      w1989 = i32[] [0, 0]  # DINT input array
      # "Reset Search and save \nbit on software start"
      n624 = call <vilib>:"connect.vi"("Use Rack/Slot for S71200/1500"=w1981, "Slot S7 300/400"=w1982, "PLC Type"=PLC_Type."S7 1200" ("PLC Type 2"), "error in (no error)"=w1984, "Rack S7 300/400"=w1983, "timeout [ms]"=1000 ("timeout [ms] 2"), "IP address"=w1991) -> ("error out"=w1985:errorcluster, "S7 Connection out"=w1986:T5)  [unwired: 3 in]
      n625 = call-poly <vilib>:"write DB.vi"("DINT input array"=w1989, "error in (no error)"=w1985, "Data Block #"=u16 43, "S7 Connection in"=w1986) -> ("error out"=w1988:errorcluster, "S7 Connection out"=w1987:T5)  [unwired: 4 in, 2 out]
      n626 = while {
        shift-right: [w1998] -> w1992
        shift-left: w1987 -> [w2008]
        shift-right: [w2006] -> w1993
        shift-left: w1988 -> [w2007]
        tunnel: w1991 -> [w1997]
        stop <- w2000 stop-if-true
        # "OP 60"
        n627 = flat-sequence {
          tunnel: [w2011] -> w2004
          tunnel: [w2009] -> w1999
          tunnel: w2007 -> [w2059]
          tunnel: w2008 -> [w2058]
          tunnel: w1997 -> [w2046]
          tunnel: [w2046] -> w1996
          tunnel: [w2087] -> w2006
          tunnel: [w2086] -> w1998
          tunnel: w2004 -> [w2089]
          tunnel: w1999 -> [w2088]
          tunnel: w1996 -> [w2085]
          frame #0 {
            w2042 = u16 44 ("Data Block #")
            w2023 = u16 43 ("Data Block #")
            # "AUTO WRITE"
            n628 = global read "DATA LOG.vi" "OP 60 Outputs"() -> (w2057:bool)
            n629 = case shown="True" w2057 {
              tunnel: w2058 -> [w2070 w2083]
              tunnel: [w2071 w2072] -> w2034
              tunnel: [w2070 w2075] -> w2033
              tunnel: w2059 -> [w2071 w2080]
              frame False {
              }
              frame True {
                w2084 = u16 44  # Data Block #
                n630 = call "PADMINI_AUTO_BARCODE_STATUS 60.vi"("Enum"=enum16{"Read", "Write"}."Read", "error in (no error)"=w2080) -> ("error out"=w2079:errorcluster, "O/P"=w2081:i32[])  [unwired: 8 in]
                n631 = global write "DATA LOG.vi" "OP 60 Outputs"(FALSE) -> ()
                n632 = call-poly <vilib>:"write DB.vi"("DINT input array"=w2081, "error in (no error)"=w2079, "Data Block #"=w2084, "S7 Connection in"=w2083) -> ("error out"=w2073:errorcluster, "S7 Connection out"=w2074:T5)  [unwired: 4 in, 2 out]
                n633 = call-poly <vilib>:"write DB.vi"("DINT input array"=i32[] [0] ("Data Byte"), "error in (no error)"=w2073, "Data Block #"=u16 43, "S7 Connection in"=w2074) -> ("error out"=w2072:errorcluster, "S7 Connection out"=w2075:T5)  [unwired: 4 in, 2 out]
              }
            }
            n634 = global read "DATA LOG.vi" "OP 60 reset"() -> (w2032:bool)
            n635 = global read "DATA LOG.vi" "Auto Cycle On"() -> (w2020:bool)
            n636 = case shown="True" w2032 {
              tunnel: w2034 -> [w2060 w2069]
              tunnel: [w2060 w2068] -> w2035
              tunnel: w2033 -> [w2061 w2067]
              tunnel: [w2061 w2066] -> w2036
              frame False {
              }
              frame True {
                n637 = global write "DATA LOG.vi" "OP 60 reset"(FALSE) -> ()
                n638 = call-poly <vilib>:"write DB.vi"("Item offset [byte]"=u16 4 ("Data Block #"), "DINT input array"=i32[] [0], "error in (no error)"=w2069, "Data Block #"=u16 43, "S7 Connection in"=w2067) -> ("error out"=w2068:errorcluster, "S7 Connection out"=w2066:T5)  [unwired: 3 in, 2 out]
              }
            }
            n639 = Boolean To (0,1)(Boolean=w2020) -> (0, 1=w2019:i16)
            n640 = Build Array(w2019) -> (w2018:i16[])
            n641 = global read "Global 1.vi" "Filtered BARCODE selected"() -> (w2045:string[])
            n642 = call-poly <vilib>:"write DB.vi"("Item offset [byte]"=u32 20, "DINT input array"=w2018, "error in (no error)"=w2035, "Data Block #"=w2042, "S7 Connection in"=w2036) -> ("error out"=w2040:errorcluster, "S7 Connection out"=w2039:T5)  [unwired: 3 in, 2 out]
            n643 = call-poly <vilib>:"write DB.vi"("Item offset [byte]"=u32 24, "Input STRINGS"=w2045, "error in (no error)"=w2040, "String length reserved in DB (default=254)"=u16 15, "Data Block #"=w2042, "S7 Connection in"=w2039) -> ("error out"=w2037:errorcluster, "S7 Connection out"=w2038:T5)  [unwired: 2 in, 2 out]
            n644 = call-poly <vilib>:"read DB.vi"("Item offset [byte]"=u32 8, "error in (no error)"=w2037, "items #"=u16 6 ("Items # [byte]"), "Data Block #"=w2023, "S7 Connection in"=w2038) -> ("error out"=w2049:errorcluster, "REAL result array"=w2047:sgl[], "S7 Connection out"=w2055:T5)  [unwired: 4 in]
            n645 = call "PADMINI_AUTO_CYCLE VALUE 60.vi"("Enum"=enum16{"Read", "Write"}."Write", "error in (no error)"=w2049, "Input"=w2047) -> ("error out"=w2048:errorcluster)  [unwired: 7 in, 1 out]
            n646 = call-poly <vilib>:"read DB.vi"("Item offset [byte]"=u32 32, "String length reserved in DB (default=254)"=u16 50, "error in (no error)"=w2048, "items #"=u16 1 ("Items # [byte]"), "Data Block #"=w2023, "S7 Connection in"=w2055) -> ("error out"=w2027:errorcluster, "STRING result Array"=w2025:string[], "S7 Connection out"=w2026:T5)  [unwired: 2 in, 1 out]
            n647 = call-poly <vilib>:"read DB.vi"("Item offset [byte]"=u32 84, "String length reserved in DB (default=254)"=u16 10, "error in (no error)"=w2027, "items #"=u16 7 ("Items # [byte]"), "Data Block #"=w2023, "S7 Connection in"=w2026) -> ("error out"=w2028:errorcluster, "STRING result Array"=w2031:string[], "S7 Connection out"=w2012:T5)  [unwired: 2 in, 1 out]
            n648 = Build Array (concatenate)(w2025, w2031) -> (w2024:string[])
            n649 = call "PADMINI_AUTO_BARCODE_STRING 60.vi"("Enum"=enum16{"Read", "Write"}."Write", "error in (no error)"=w2028, "Input"=w2024) -> ("error out"=w2010:errorcluster)  [unwired: 7 in, 1 out]
            n650 = call-poly <vilib>:"read DB.vi"("error in (no error)"=w2010, "items #"=u16 2 ("Items # [byte]"), "Data Block #"=u16 43, "S7 Connection in"=w2012) -> ("error out"=w2017:errorcluster, "DINT result array"=w2015:i32[], "S7 Connection out"=w2011:T5)  [unwired: 5 in]
            n651 = call "PADMINI_AUTO_CYCLE STATE 60.vi"("Enum"=enum16{"Read", "Write"}."Write", "error in (no error)"=w2017, "Input"=w2015) -> ("error out"=w2009:errorcluster)  [unwired: 7 in, 1 out]
          }
          frame #1 {
            # "RECONNECT"
            n652 = case shown="Error" w2088 {
              selector: w2088 -> [w2093 w2094]
              tunnel: [w2092 w2098] -> w2086
              tunnel: [w2093 w2099] -> w2087
              tunnel: w2089 -> [w2092 w2097]
              tunnel: w2085 -> [_ w2096]
              frame No Error {
              }
              frame Error {
                n653 = Unbundle By Name(w2094) -> ("code"=w2095:i32)
                n654 = call <vilib>:"Clear Errors.vi"("error in (no error)"=w2094) -> ("error out"=w2100:errorcluster)  [unwired: 5 in, 1 out]
                n655 = case shown="0, Default" w2095 {
                  tunnel: w2100 -> [w2102 w2113]
                  tunnel: [w2102 w2111] -> w2099
                  tunnel: [w2103 w2110] -> w2098
                  tunnel: w2097 -> [w2103 w2107]
                  tunnel: w2096 -> [_ w2106]
                  tunnel: w2094 -> [w2101 _]
                  frame 0, Default {
                    n656 = global write "Global 1.vi" "PLC5 error"(w2101) -> ()
                  }
                  frame 1, 66 {
                    n657 = call <vilib>:"disconnect.vi"("error in (no error)"=w2113, "S7 Connection in"=w2107) -> ("error out"=w2112:errorcluster)  [unwired: 8 in, 1 out]
                    n658 = call <vilib>:"Clear Errors.vi"("error in (no error)"=w2112) -> ("error out"=w2109:errorcluster)  [unwired: 5 in, 1 out]
                    n659 = call <vilib>:"connect.vi"("Use Rack/Slot for S71200/1500"=TRUE, "Slot S7 300/400"=u8 1, "PLC Type"=PLC_Type."S7 1200" ("PLC Type 2"), "error in (no error)"=w2109, "IP address"=w2106) -> ("error out"=w2111:errorcluster, "S7 Connection out"=w2110:T5)  [unwired: 5 in]
                  }
                }
              }
            }
            n660 = Unbundle By Name(w2088) -> ("status"=w2091:bool)
            n661 = Not(x=w2091) -> (.not. x?=w2090:bool)
            "PLC 5" <- w2090
            n662 = global write "Global 1.vi" "PLC 5"(w2090) -> ()
          }
        }
        n663 = call "PADMINI_STOP_ALL.vi"("Enum"=enum16{"Read", "Write"}."Read") -> ("Boolean 2"=w2002:bool)  [unwired: 9 in, 1 out]
        n664 = local read "stop"() -> (w2001:bool)
        n665 = Or(x=w2001, y=w2002) -> (x .or. y?=w2000:bool)
        n666 = Wait (ms)(milliseconds to wait=u32 1200) -> ()  [unwired: 1 out]
      }
      n667 = call <vilib>:"Clear Errors.vi"("error in (no error)"=w1993) -> ("error out"=w1980:errorcluster)  [unwired: 5 in, 1 out]
      n668 = call <vilib>:"disconnect.vi"("error in (no error)"=w1980, "S7 Connection in"=w1992) -> ("error out"=w1979:errorcluster)  [unwired: 8 in, 1 out]
    }
    frame Enabled {
      w2117 = PLC_Comm_State."Int"  # Enum
      n669 = while {
        shift-right: [w2129] -> _
        shift-left: w2117 -> [w2137]
        shift-right: [w2121] -> w2114
        shift-left: w2115 -> [w2136]
        shift-right: [w2132] -> _
        shift-left: _ -> [w2135]
        tunnel: w2116 -> [w2118]
        stop <- w2130 stop-if-true
        w2126 = PLC_Comm_State."Disconnect"  # Enum
        w2134 = u32 800  # milliseconds to wait
        # "Int-->Write-->Read---if--Error-->reconnect\n               ^------v                                       v\n                ^------------------------------v"
        # "OP 60"
        n670 = case shown="\"Int\"" w2137 {
          selector: w2137 -> [w2153 w2170 w2208 w2262 w2274 w2278 _ _ _ _]
          tunnel: [w2158 w2172 w2187 w2237 w2275 w2283 w2285 w2288 w2290 w2292] -> w2138
          tunnel: [w2159 w2171 w2190 w2234 w2276 w2280 w2286 w2287 w2289 w2291] -> w2131
          tunnel: w2136 -> [w2156 w2167 w2188 w2236 w2272 w2281 w2285 w2288 w2290 w2292]
          tunnel: w2135 -> [w2154 _ w2189 w2235 w2276 w2282 w2286 w2287 w2289 w2291]
          tunnel: [w2152 w2169 w2207 w2261 w2273 w2277 _ _ _ _] -> w2133
          tunnel: [_ _ _ _ _ TRUE _ _ _ _] -> w2130
          tunnel: [w2153 w2170 w2208 w2262 w2274 w2278 _ _ _ _] -> w2127
          tunnel: w2118 -> [w2151 w2168 _ _ _ _ _ _ _ _]
          frame "Connect" {
            w2152 = PLC_Comm_State."Write"  # Enum
            w2164 = TRUE  # Use Rack/Slot for S71200/1500
            w2163 = u8 1  # Slot S7 300/400
            w2161 = u8 0  # Rack S7 300/400
            # "Reconect"
            n671 = call <vilib>:"disconnect.vi"("error in (no error)"=w2156, "S7 Connection in"=w2154) -> ("error out"=w2157:errorcluster)  [unwired: 8 in, 1 out]
            n672 = call <vilib>:"Clear Errors.vi"("error in (no error)"=w2157) -> ("error out"=w2155:errorcluster)  [unwired: 5 in, 1 out]
            n673 = call <vilib>:"connect.vi"("Use Rack/Slot for S71200/1500"=w2164, "Slot S7 300/400"=w2163, "PLC Type"=PLC_Type."S7 1200" ("PLC Type 2"), "error in (no error)"=w2155, "Rack S7 300/400"=w2161, "timeout [ms]"=1000 ("timeout [ms] 2"), "IP address"=w2151) -> ("error out"=w2158:errorcluster, "S7 Connection out"=w2159:T5)  [unwired: 3 in]
          }
          frame "Int" {
            w2169 = PLC_Comm_State."Write"  # Enum
            w2173 = TRUE  # Use Rack/Slot for S71200/1500
            w2174 = u8 1  # Slot S7 300/400
            w2175 = u8 0  # Rack S7 300/400
            w2176 = u16[] [43]  # Data Block #
            # "Initialize and set first bits"
            n674 = call "Stall Data Flow.vim"("value in"=w2167, "milliseconds to wait"=u32 516) -> ("value out"=w2166:errorcluster)  [unwired: 1 out]
            n675 = call <vilib>:"connect.vi"("Use Rack/Slot for S71200/1500"=w2173, "Slot S7 300/400"=w2174, "PLC Type"=PLC_Type."S7 1200" ("PLC Type 2"), "error in (no error)"=w2166, "Rack S7 300/400"=w2175, "timeout [ms]"=1000 ("timeout [ms] 2"), "IP address"=w2168) -> ("error out"=w2178:errorcluster, "S7 Connection out"=w2177:T5)  [unwired: 3 in]
            n676 = for {
              tunnel: w2176 -> [w2186] mode=indexing
              shift-right: [w2184] -> w2171
              shift-left: w2177 -> [w2182]
              tunnel: w2178 -> [w2183]
              tunnel: [w2181] -> w2172
              w2185 = i32[] [0, 0]  # DINT input array
              # "Reset Search and save \nbit on software start"
              n677 = call-poly <vilib>:"write DB.vi"("DINT input array"=w2185, "error in (no error)"=w2183, "Data Block #"=w2186, "S7 Connection in"=w2182) -> ("error out"=w2181:errorcluster, "S7 Connection out"=w2184:T5)  [unwired: 4 in, 2 out]
            }
          }
          frame "Write" {
            w2192 = u16 44 ("Data Block #")
            w2207 = PLC_Comm_State."Read"  # Enum
            n678 = global read "DATA LOG.vi" "OP 60 Outputs"() -> (w2206:bool)
            n679 = case shown="True" w2206 {
              tunnel: w2189 -> [w2219 w2232]
              tunnel: [w2220 w2222] -> w2200
              tunnel: [w2219 w2225] -> w2199
              tunnel: w2188 -> [w2220 w2229]
              frame False {
              }
              frame True {
                w2233 = u16 44  # Data Block #
                n680 = call "PADMINI_AUTO_BARCODE_STATUS 60.vi"("Enum"=enum16{"Read", "Write"}."Read", "error in (no error)"=w2229) -> ("error out"=w2228:errorcluster, "O/P"=w2230:i32[])  [unwired: 8 in]
                n681 = call-poly <vilib>:"write DB.vi"("DINT input array"=w2230, "error in (no error)"=w2228, "Data Block #"=w2233, "S7 Connection in"=w2232) -> ("error out"=w2223:errorcluster, "S7 Connection out"=w2224:T5)  [unwired: 4 in, 2 out]
                n682 = call-poly <vilib>:"write DB.vi"("DINT input array"=i32[] [0] ("Data Byte"), "error in (no error)"=w2223, "Data Block #"=u16 43, "S7 Connection in"=w2224) -> ("error out"=w2222:errorcluster, "S7 Connection out"=w2225:T5)  [unwired: 4 in, 2 out]
                n683 = Unbundle By Name(w2222) -> ("status"=w2221:bool)
                n684 = global write "DATA LOG.vi" "OP 60 Outputs"(w2221) -> ()
              }
            }
            n685 = global read "DATA LOG.vi" "OP 60 reset"() -> (w2198:bool)
            n686 = global read "DATA LOG.vi" "Auto Cycle On"() -> (w2197:bool)
            n687 = case shown="True" w2198 {
              tunnel: w2200 -> [w2209 w2218]
              tunnel: [w2209 w2212] -> w2201
              tunnel: w2199 -> [w2210 w2217]
              tunnel: [w2210 w2216] -> w2202
              frame False {
              }
              frame True {
                n688 = call-poly <vilib>:"write DB.vi"("Item offset [byte]"=u16 4 ("Data Block #"), "DINT input array"=i32[] [0], "error in (no error)"=w2218, "Data Block #"=u16 43, "S7 Connection in"=w2217) -> ("error out"=w2212:errorcluster, "S7 Connection out"=w2216:T5)  [unwired: 3 in, 2 out]
                n689 = Unbundle By Name(w2212) -> ("status"=w2211:bool)
                n690 = global write "DATA LOG.vi" "OP 60 reset"(w2211) -> ()
              }
            }
            n691 = Boolean To (0,1)(Boolean=w2197) -> (0, 1=w2196:i16)
            n692 = Build Array(w2196) -> (w2195:i16[])
            n693 = global read "Global 1.vi" "Filtered BARCODE selected"() -> (w2205:string[])
            n694 = call-poly <vilib>:"write DB.vi"("Item offset [byte]"=u32 20, "DINT input array"=w2195, "error in (no error)"=w2201, "Data Block #"=w2192, "S7 Connection in"=w2202) -> ("error out"=w2204:errorcluster, "S7 Connection out"=w2203:T5)  [unwired: 3 in, 2 out]
            n695 = call-poly <vilib>:"write DB.vi"("Item offset [byte]"=u32 24, "Input STRINGS"=w2205, "error in (no error)"=w2204, "String length reserved in DB (default=254)"=u16 15, "Data Block #"=w2192, "S7 Connection in"=w2203) -> ("error out"=w2187:errorcluster, "S7 Connection out"=w2190:T5)  [unwired: 2 in, 2 out]
          }
          frame "Read" {
            w2243 = u16 43 ("Data Block #")
            w2261 = PLC_Comm_State."Write"  # Enum
            n696 = call-poly <vilib>:"read DB.vi"("Item offset [byte]"=u32 8, "error in (no error)"=w2236, "items #"=u16 6 ("Items # [byte]"), "Data Block #"=w2243, "S7 Connection in"=w2235) -> ("error out"=w2257:errorcluster, "REAL result array"=w2260:sgl[], "S7 Connection out"=w2258:T5)  [unwired: 4 in]
            n697 = call-poly <vilib>:"read DB.vi"("Item offset [byte]"=u32 32, "String length reserved in DB (default=254)"=u16 50, "error in (no error)"=w2257, "items #"=u16 1 ("Items # [byte]"), "Data Block #"=w2243, "S7 Connection in"=w2258) -> ("error out"=w2254:errorcluster, "STRING result Array"=w2252:string[], "S7 Connection out"=w2253:T5)  [unwired: 2 in, 1 out]
            n698 = call-poly <vilib>:"read DB.vi"("Item offset [byte]"=u32 84, "String length reserved in DB (default=254)"=u16 10, "error in (no error)"=w2254, "items #"=u16 7 ("Items # [byte]"), "Data Block #"=w2243, "S7 Connection in"=w2253) -> ("error out"=w2255:errorcluster, "STRING result Array"=w2256:string[], "S7 Connection out"=w2249:T5)  [unwired: 2 in, 1 out]
            n699 = Build Array (concatenate)(w2252, w2256) -> (w2259:string[])
            n700 = call-poly <vilib>:"read DB.vi"("error in (no error)"=w2255, "items #"=u16 2 ("Items # [byte]"), "Data Block #"=u16 43, "S7 Connection in"=w2249) -> ("error out"=w2251:errorcluster, "DINT result array"=w2250:i32[], "S7 Connection out"=w2234:T5)  [unwired: 5 in]
            n701 = case shown="No Error" w2251 {
              selector: w2251 -> [w2264 w2271]
              tunnel: w2250 -> [w2263 _]
              tunnel: w2259 -> [w2270 _]
              tunnel: w2260 -> [w2268 _]
              tunnel: [w2265 w2271] -> w2237
              frame No Error {
                w2269 = enum16{"Read", "Write"}."Write" ("Enum")
                n702 = call "PADMINI_AUTO_BARCODE_STRING 60.vi"("Enum"=w2269, "error in (no error)"=w2264, "Input"=w2270) -> ("error out"=w2267:errorcluster)  [unwired: 7 in, 1 out]
                n703 = call "PADMINI_AUTO_CYCLE VALUE 60.vi"("Enum"=w2269, "error in (no error)"=w2267, "Input"=w2268) -> ("error out"=w2266:errorcluster)  [unwired: 7 in, 1 out]
                n704 = call "PADMINI_AUTO_CYCLE STATE 60.vi"("Enum"=w2269, "error in (no error)"=w2266, "Input"=w2263) -> ("error out"=w2265:errorcluster)  [unwired: 7 in, 1 out]
              }
              frame Error {
              }
            }
          }
          frame "Error" {
            w2273 = PLC_Comm_State."Connect"  # Enum
            n705 = global write "Global 1.vi" "PLC5 error"(w2272) -> ()
            n706 = call <vilib>:"Clear Errors.vi"("error in (no error)"=w2272) -> ("error out"=w2275:errorcluster)  [unwired: 5 in, 1 out]
          }
          frame "Disconnect" {
            w2277 = PLC_Comm_State."Disconnect"  # Enum
            w2280 = T5 {"TCP Connection Ref"=refnum, "IP address"="", "timeout ms"=5000, "Connected?"=FALSE, "PLC Type"=enum."S7 1200", "Rack S7 400"=0, "Slot S7 400"=0, "PDU Size"=0, "connection semaphore"=refnum}  # S7 Connection out
            n707 = call <vilib>:"Clear Errors.vi"("error in (no error)"=w2281) -> ("error out"=w2284:errorcluster)  [unwired: 5 in, 1 out]
            n708 = call <vilib>:"disconnect.vi"("error in (no error)"=w2284, "S7 Connection in"=w2282) -> ("error out"=w2283:errorcluster)  [unwired: 8 in, 1 out]
          }
          frame "Write2" {
            # "No Use"
          }
          frame "Write3" {
            # "No Use"
          }
          frame "Read2" {
            # "No Use"
          }
          frame "Read3" {
            # "No Use"
          }
        }
        n709 = Wait (ms)(milliseconds to wait=w2134) -> ()  [unwired: 1 out]
        n710 = call "PADMINI_STOP_ALL.vi"("Enum"=enum16{"Read", "Write"}."Read") -> ("Boolean 2"=w2125:bool)  [unwired: 9 in, 1 out]
        n711 = local read "stop"() -> (w2120:bool)
        n712 = case shown="Error" w2138 {
          selector: w2138 -> [w2141 w2144]
          tunnel: [w2141 w2143] -> w2121
          tunnel: [w2140 w2142] -> w2128
          tunnel: w2133 -> [w2140 _]
          tunnel: [w2139 w2150] -> w2132
          tunnel: w2131 -> [w2139 w2150]
          tunnel: w2127 -> [_ w2148]
          frame No Error {
          }
          frame Error {
            w2142 = PLC_Comm_State."Error"  # Enum
            n713 = Unbundle By Name(w2144) -> ("source"=w2149:string)
            n714 = call <userlib>:"Get Strings from Enum__ogtk.vi"("Enum"=w2148) -> ("String Value"=w2147:string)  [unwired: 7 in, 3 out]
            n715 = Concatenate Strings(w2147, "    " ("string"), w2149) -> (w2145:string)
            n716 = Bundle By Name(cluster=w2144, "source"=w2145) -> (w2143:errorcluster)
          }
        }
        n717 = Or(x=w2120, y=w2125) -> (x .or. y?=w2123:bool)
        n718 = Select(t=w2126, s=w2123, f=w2128) -> (s? t:f=w2129:T1)
        n719 = Unbundle By Name(w2121) -> ("status"=w2122:bool)
        n720 = Not(x=w2122) -> (.not. x?=w2119:bool)
        n721 = global write "Global 1.vi" "PLC 5"(w2119) -> ()
      }
    }
  }
  n722 = disable-structure shown="Enabled" {
    disable-tunnel: [w2306 _] -> w117
    disable-tunnel: [w2303 _] -> w106
    disable-tunnel: w82 -> [w2302 w2368]
    disable-tunnel: w9 -> [w2296 w2367]
    frame Disabled {
      n723 = call <vilib>:"connect.vi"("Use Rack/Slot for S71200/1500"=TRUE, "Slot S7 300/400"=u8 1, "PLC Type"=PLC_Type."S7 1200" ("PLC Type 2"), "error in (no error)"=w2296, "Rack S7 300/400"=u8 0, "timeout [ms]"=1000, "IP address"=w2302) -> ("error out"=w2298:errorcluster, "S7 Connection out"=w2297:T5)  [unwired: 3 in]
      n724 = for {
        tunnel: u16[] [83, 94] ("Data Block #") -> [w2312] mode=indexing
        shift-right: [w2310] -> w2300
        shift-left: w2297 -> [w2307]
        tunnel: w2298 -> [w2308]
        tunnel: [w2309] -> w2299
        w2311 = i32[] [0, 0]  # DINT input array
        # "Reset Search and save \nbit on software start"
        n725 = call-poly <vilib>:"write DB.vi"("DINT input array"=w2311, "error in (no error)"=w2308, "Data Block #"=w2312, "S7 Connection in"=w2307) -> ("error out"=w2309:errorcluster, "S7 Connection out"=w2310:T5)  [unwired: 4 in, 2 out]
      }
      n726 = while {
        shift-right: [w2315] -> w2303
        shift-left: w2300 -> [w2325]
        shift-right: [w2323] -> w2306
        shift-left: w2299 -> [w2324]
        tunnel: w2302 -> [w2313]
        stop <- w2318 stop-if-true
        # "OP 10 AND 20"
        n727 = flat-sequence {
          tunnel: [w2328] -> w2317
          tunnel: [w2334] -> w2316
          tunnel: w2324 -> [w2335]
          tunnel: w2325 -> [w2336]
          tunnel: [w2333] -> w2314
          tunnel: w2313 -> [w2333]
          tunnel: [w2340] -> w2323
          tunnel: [w2339] -> w2315
          tunnel: w2317 -> [w2341]
          tunnel: w2316 -> [w2337]
          tunnel: w2314 -> [w2338]
          frame #0 {
            # "NEW CHANGES"
            n728 = call "PLC_OP10_Write.vi"("error in (no error)"=w2335, "S7 Connection in"=w2336) -> ("error out"=w2331:errorcluster, "S7 Connection out"=w2332:T5)  [unwired: 8 in]
            n729 = call "PLC_OP10_Read.vi"("error in (no error)"=w2331, "S7 Connection in"=w2332) -> ("error out"=w2330:errorcluster, "S7 Connection out"=w2329:T5)  [unwired: 8 in]
            n730 = call "PLC_OP20_Write.vi"("error in (no error)"=w2330, "S7 Connection in"=w2329) -> ("error out"=w2326:errorcluster, "S7 Connection out"=w2327:T5)  [unwired: 8 in]
            n731 = call "PLC_OP20_Read.vi"("error in (no error)"=w2326, "S7 Connection in"=w2327) -> ("error out"=w2334:errorcluster, "S7 Connection out 2"=w2328:T5)  [unwired: 8 in]
          }
          frame #1 {
            # "RECONNECT"
            n732 = case shown="Error" w2337 {
              selector: w2337 -> [w2345 w2347]
              tunnel: [w2344 w2350] -> w2339
              tunnel: [w2345 w2351] -> w2340
              tunnel: w2341 -> [w2344 w2349]
              tunnel: w2338 -> [_ w2348]
              frame No Error {
              }
              frame Error {
                n733 = Unbundle By Name(w2347) -> ("code"=w2346:i32)
                n734 = case shown="1, 66" w2346 {
                  tunnel: w2347 -> [w2352 w2365]
                  tunnel: [w2353 w2363] -> w2351
                  tunnel: [w2354 w2362] -> w2350
                  tunnel: w2349 -> [w2354 w2359]
                  tunnel: w2348 -> [_ w2358]
                  frame 0, Default {
                    n735 = call <vilib>:"Clear Errors.vi"("error in (no error)"=w2352) -> ("error out"=w2353:errorcluster)  [unwired: 5 in, 1 out]
                    n736 = global write "Global 1.vi" "PLC1 error"(w2352) -> ()
                  }
                  frame 1, 66 {
                    w2357 = 1000  # timeout [ms]
                    n737 = call <vilib>:"Clear Errors.vi"("error in (no error)"=w2365) -> ("error out"=w2366:errorcluster)  [unwired: 5 in, 1 out]
                    n738 = call <vilib>:"disconnect.vi"("error in (no error)"=w2366, "S7 Connection in"=w2359) -> ("error out"=w2364:errorcluster)  [unwired: 8 in, 1 out]
                    n739 = call <vilib>:"Clear Errors.vi"("error in (no error)"=w2364) -> ("error out"=w2361:errorcluster)  [unwired: 5 in, 1 out]
                    n740 = call <vilib>:"connect.vi"("Use Rack/Slot for S71200/1500"=TRUE, "Slot S7 300/400"=u8 1, "PLC Type"=PLC_Type."S7 1200" ("PLC Type 2"), "error in (no error)"=w2361, "timeout [ms]"=w2357, "IP address"=w2358) -> ("error out"=w2363:errorcluster, "S7 Connection out"=w2362:T5)  [unwired: 4 in]
                  }
                }
              }
            }
            n741 = Unbundle By Name(w2337) -> ("status"=w2343:bool)
            n742 = Not(x=w2343) -> (.not. x?=w2342:bool)
            "PLC 1" <- w2342
            n743 = global write "Global 1.vi" "PLC 1"(w2342) -> ()
          }
        }
        n744 = call "PADMINI_STOP_ALL.vi"("Enum"=enum16{"Read", "Write"}."Read") -> ("Boolean 2"=w2320:bool)  [unwired: 9 in, 1 out]
        n745 = Wait (ms)(milliseconds to wait=u32 1200) -> ()  [unwired: 1 out]
        n746 = Or(x="stop", y=w2320) -> (x .or. y?=w2318:bool)
      }
    }
    frame Enabled {
      w2369 = PLC_Comm_State."Int"  # Enum
      n747 = while {
        shift-right: [w2381] -> _
        shift-left: w2369 -> [w2389]
        shift-right: [w2373] -> _
        shift-left: w2367 -> [w2388]
        shift-right: [w2384] -> _
        shift-left: _ -> [w2387]
        tunnel: w2368 -> [w2370]
        stop <- w2382 stop-if-true
        w2378 = PLC_Comm_State."Disconnect"  # Enum
        w2386 = u32 800  # milliseconds to wait
        # "Int-->Write-->Read---if--Error-->reconnect\n               ^------v                                       v\n                ^------------------------------v"
        # "OP 10-20"
        n748 = case shown="\"Int\"" w2389 {
          selector: w2389 -> [w2405 w2420 w2442 w2447 w2454 w2459 w2463 w2467 _ _]
          tunnel: [w2410 w2423 w2439 w2443 w2451 w2457 w2464 w2472 w2475 w2477] -> w2390
          tunnel: [w2411 w2422 w2437 w2445 w2449 w2455 w2465 w2469 w2474 w2476] -> w2383
          tunnel: w2388 -> [w2408 w2421 w2440 w2444 w2452 w2458 w2461 w2470 w2475 w2477]
          tunnel: w2387 -> [w2406 _ w2438 w2446 w2450 w2456 w2465 w2471 w2474 w2476]
          tunnel: [w2404 w2419 w2441 w2448 w2453 w2460 w2462 w2466 _ _] -> w2385
          tunnel: [_ _ _ _ _ _ _ TRUE _ _] -> w2382
          tunnel: [w2405 w2420 w2442 w2447 w2454 w2459 w2463 w2467 _ _] -> w2379
          tunnel: w2370 -> [w2403 w2418 _ _ _ _ _ _ _ _]
          frame "Connect" {
            w2404 = PLC_Comm_State."Write"  # Enum
            w2416 = TRUE  # Use Rack/Slot for S71200/1500
            w2415 = u8 1  # Slot S7 300/400
            w2413 = u8 0  # Rack S7 300/400
            # "Reconect"
            n749 = call <vilib>:"disconnect.vi"("error in (no error)"=w2408, "S7 Connection in"=w2406) -> ("error out"=w2409:errorcluster)  [unwired: 8 in, 1 out]
            n750 = call <vilib>:"Clear Errors.vi"("error in (no error)"=w2409) -> ("error out"=w2407:errorcluster)  [unwired: 5 in, 1 out]
            n751 = call <vilib>:"connect.vi"("Use Rack/Slot for S71200/1500"=w2416, "Slot S7 300/400"=w2415, "PLC Type"=PLC_Type."S7 1200" ("PLC Type 2"), "error in (no error)"=w2407, "Rack S7 300/400"=w2413, "timeout [ms]"=1000 ("timeout [ms] 2"), "IP address"=w2403) -> ("error out"=w2410:errorcluster, "S7 Connection out"=w2411:T5)  [unwired: 3 in]
          }
          frame "Int" {
            w2419 = PLC_Comm_State."Write"  # Enum
            w2424 = TRUE  # Use Rack/Slot for S71200/1500
            w2425 = u8 1  # Slot S7 300/400
            w2426 = u8 0  # Rack S7 300/400
            # "Initialize and set first bits"
            n752 = call <vilib>:"connect.vi"("Use Rack/Slot for S71200/1500"=w2424, "Slot S7 300/400"=w2425, "PLC Type"=PLC_Type."S7 1200" ("PLC Type 2"), "error in (no error)"=w2421, "Rack S7 300/400"=w2426, "timeout [ms]"=1000 ("timeout [ms] 2"), "IP address"=w2418) -> ("error out"=w2428:errorcluster, "S7 Connection out"=w2427:T5)  [unwired: 3 in]
            n753 = for {
              tunnel: u16[] [83, 94] ("Data Block #") -> [w2436] mode=indexing
              shift-right: [w2434] -> w2422
              shift-left: w2427 -> [w2432]
              tunnel: w2428 -> [w2433]
              tunnel: [w2431] -> w2423
              w2435 = i32[] [0, 0]  # DINT input array
              # "Reset Search and save \nbit on software start"
              n754 = call-poly <vilib>:"write DB.vi"("DINT input array"=w2435, "error in (no error)"=w2433, "Data Block #"=w2436, "S7 Connection in"=w2432) -> ("error out"=w2431:errorcluster, "S7 Connection out"=w2434:T5)  [unwired: 4 in, 2 out]
            }
          }
          frame "Write" {
            w2441 = PLC_Comm_State."Write2"  # Enum
            # "OP 10 Write"
            n755 = call "PLC_OP10_Write.vi"("error in (no error)"=w2440, "S7 Connection in"=w2438) -> ("error out"=w2439:errorcluster, "S7 Connection out"=w2437:T5)  [unwired: 8 in]
          }
          frame "Write2" {
            w2448 = PLC_Comm_State."Read"  # Enum
            # "op 20 wirte 2"
            n756 = call "PLC_OP20_Write.vi"("error in (no error)"=w2444, "S7 Connection in"=w2446) -> ("error out"=w2443:errorcluster, "S7 Connection out"=w2445:T5)  [unwired: 8 in]
          }
          frame "Read" {
            w2453 = PLC_Comm_State."Read2"  # Enum
            # "OP10 read"
            n757 = call "PLC_OP10_Read.vi"("error in (no error)"=w2452, "S7 Connection in"=w2450) -> ("error out"=w2451:errorcluster, "S7 Connection out"=w2449:T5)  [unwired: 8 in]
          }
          frame "Read2" {
            w2460 = PLC_Comm_State."Write"  # Enum
            # "Op20 Read2"
            n758 = call "PLC_OP20_Read.vi"("error in (no error)"=w2458, "S7 Connection in"=w2456) -> ("error out"=w2457:errorcluster, "S7 Connection out 2"=w2455:T5)  [unwired: 8 in]
          }
          frame "Error" {
            w2462 = PLC_Comm_State."Connect"  # Enum
            n759 = global write "Global 1.vi" "PLC1 error"(w2461) -> ()
            n760 = call <vilib>:"Clear Errors.vi"("error in (no error)"=w2461) -> ("error out"=w2464:errorcluster)  [unwired: 5 in, 1 out]
          }
          frame "Disconnect" {
            w2466 = PLC_Comm_State."Disconnect"  # Enum
            w2469 = T5 {"TCP Connection Ref"=refnum, "IP address"="", "timeout ms"=5000, "Connected?"=FALSE, "PLC Type"=enum."S7 1200", "Rack S7 400"=0, "Slot S7 400"=0, "PDU Size"=0, "connection semaphore"=refnum}  # S7 Connection out
            n761 = call <vilib>:"Clear Errors.vi"("error in (no error)"=w2470) -> ("error out"=w2473:errorcluster)  [unwired: 5 in, 1 out]
            n762 = call <vilib>:"disconnect.vi"("error in (no error)"=w2473, "S7 Connection in"=w2471) -> ("error out"=w2472:errorcluster)  [unwired: 8 in, 1 out]
          }
          frame "Write3" {
            # "No Use"
          }
          frame "Read3" {
            # "No Use"
          }
        }
        n763 = Wait (ms)(milliseconds to wait=w2386) -> ()  [unwired: 1 out]
        n764 = call "PADMINI_STOP_ALL.vi"("Enum"=enum16{"Read", "Write"}."Read") -> ("Boolean 2"=w2377:bool)  [unwired: 9 in, 1 out]
        n765 = local read "stop"() -> (w2372:bool)
        n766 = case shown="Error" w2390 {
          selector: w2390 -> [w2393 w2396]
          tunnel: [w2393 w2395] -> w2373
          tunnel: [w2392 w2394] -> w2380
          tunnel: w2385 -> [w2392 _]
          tunnel: [w2391 w2402] -> w2384
          tunnel: w2383 -> [w2391 w2402]
          tunnel: w2379 -> [_ w2400]
          frame No Error {
          }
          frame Error {
            w2394 = PLC_Comm_State."Error"  # Enum
            n767 = Unbundle By Name(w2396) -> ("source"=w2401:string)
            n768 = call <userlib>:"Get Strings from Enum__ogtk.vi"("Enum"=w2400) -> ("String Value"=w2399:string)  [unwired: 7 in, 3 out]
            n769 = Concatenate Strings(w2399, "    " ("string"), w2401) -> (w2397:string)
            n770 = Bundle By Name(cluster=w2396, "source"=w2397) -> (w2395:errorcluster)
          }
        }
        n771 = Or(x=w2372, y=w2377) -> (x .or. y?=w2375:bool)
        n772 = Select(t=w2378, s=w2375, f=w2380) -> (s? t:f=w2381:T1)
        n773 = Unbundle By Name(w2373) -> ("status"=w2374:bool)
        n774 = Not(x=w2374) -> (.not. x?=w2371:bool)
        n775 = global write "Global 1.vi" "PLC 1"(w2371) -> ()
      }
    }
  }
  n776 = while {
    shift-right: [w2488] -> _
    shift-left: w1 -> [w2497]
    shift-right: [w2478] -> w84
    shift-left: w9 -> [w2496]
    shift-right: [w2491] -> _
    shift-left: _ -> [w2495]
    tunnel: w83 -> [w2494]
    stop <- w2489 stop-if-true
    w2485 = PLC_Comm_State."Disconnect"  # Enum
    w2493 = u32 800  # milliseconds to wait
    # "Int-->Write-->Read---if--Error-->reconnect\n               ^------v                                       v\n                ^------------------------------v"
    # "OP 30"
    n777 = case shown="\"Int\"" w2497 {
      selector: w2497 -> [w2512 w2528 w2552 w2558 w2561 w2565 _ _ _ _]
      tunnel: [w2517 w2532 w2547 w2554 w2562 w2570 w2572 w2575 w2577 w2579] -> w2498
      tunnel: [w2518 w2531 w2549 w2555 w2563 w2567 w2573 w2574 w2576 w2578] -> w2490
      tunnel: w2496 -> [w2515 w2530 w2548 w2553 w2559 w2568 w2572 w2575 w2577 w2579]
      tunnel: w2495 -> [w2513 _ w2550 w2556 w2563 w2569 w2573 w2574 w2576 w2578]
      tunnel: w2494 -> [w2519 w2529 _ _ _ _ _ _ _ _]
      tunnel: [w2511 w2527 w2551 w2557 w2560 w2564 _ _ _ _] -> w2492
      tunnel: [_ _ _ _ _ TRUE _ _ _ _] -> w2489
      tunnel: [w2512 w2528 w2552 w2558 w2561 w2565 _ _ _ _] -> w2486
      frame "Connect" {
        w2511 = PLC_Comm_State."Write"  # Enum
        w2524 = TRUE  # Use Rack/Slot for S71200/1500
        w2523 = u8 1  # Slot S7 300/400
        w2521 = u8 0  # Rack S7 300/400
        # "Reconect"
        n778 = call <vilib>:"disconnect.vi"("error in (no error)"=w2515, "S7 Connection in"=w2513) -> ("error out"=w2516:errorcluster)  [unwired: 8 in, 1 out]
        n779 = call <vilib>:"Clear Errors.vi"("error in (no error)"=w2516) -> ("error out"=w2514:errorcluster)  [unwired: 5 in, 1 out]
        n780 = call <vilib>:"connect.vi"("Use Rack/Slot for S71200/1500"=w2524, "Slot S7 300/400"=w2523, "PLC Type"=PLC_Type."S7 1200" ("PLC Type 2"), "error in (no error)"=w2514, "Rack S7 300/400"=w2521, "timeout [ms]"=1000 ("timeout [ms] 2"), "IP address"=w2519) -> ("error out"=w2517:errorcluster, "S7 Connection out"=w2518:T5)  [unwired: 3 in]
      }
      frame "Int" {
        w2527 = PLC_Comm_State."Write"  # Enum
        w2533 = TRUE  # Use Rack/Slot for S71200/1500
        w2534 = u8 1  # Slot S7 300/400
        w2535 = u8 0  # Rack S7 300/400
        w2536 = u16[] [37]  # Data Block #
        n781 = call "Stall Data Flow.vim"("value in"=w2530, "milliseconds to wait"=u32 129) -> ("value out"=w2526:errorcluster)  [unwired: 1 out]
        n782 = call <vilib>:"connect.vi"("Use Rack/Slot for S71200/1500"=w2533, "Slot S7 300/400"=w2534, "PLC Type"=PLC_Type."S7 1200" ("PLC Type 2"), "error in (no error)"=w2526, "Rack S7 300/400"=w2535, "timeout [ms]"=1000 ("timeout [ms] 2"), "IP address"=w2529) -> ("error out"=w2538:errorcluster, "S7 Connection out"=w2537:T5)  [unwired: 3 in]
        n783 = for {
          tunnel: w2536 -> [w2546] mode=indexing
          shift-right: [w2544] -> w2531
          shift-left: w2537 -> [w2542]
          tunnel: w2538 -> [w2543]
          tunnel: [w2541] -> w2532
          w2545 = i32[] [0, 0]  # DINT input array
          # "Reset Search and save \nbit on software start"
          n784 = call-poly <vilib>:"write DB.vi"("DINT input array"=w2545, "error in (no error)"=w2543, "Data Block #"=w2546, "S7 Connection in"=w2542) -> ("error out"=w2541:errorcluster, "S7 Connection out"=w2544:T5)  [unwired: 4 in, 2 out]
        }
      }
      frame "Write" {
        w2551 = PLC_Comm_State."Read"  # Enum
        n785 = call "PLC_OP30_Write.vi"("error in (no error)"=w2548, "S7 Connection in"=w2550) -> ("error out"=w2547:errorcluster, "S7 Connection out"=w2549:T5)  [unwired: 8 in]
      }
      frame "Read" {
        w2557 = PLC_Comm_State."Write"  # Enum
        # "OP100 OK\nOP 100 NG"
        n786 = call "PLC_OP30_Read.vi"("error in (no error)"=w2553, "S7 Connection in"=w2556) -> ("error out"=w2554:errorcluster, "S7 Connection out 2"=w2555:T5)  [unwired: 8 in]
      }
      frame "Error" {
        w2560 = PLC_Comm_State."Connect"  # Enum
        n787 = global write "Global 1.vi" "PLC2 error"(w2559) -> ()
        n788 = call <vilib>:"Clear Errors.vi"("error in (no error)"=w2559) -> ("error out"=w2562:errorcluster)  [unwired: 5 in, 1 out]
      }
      frame "Disconnect" {
        w2564 = PLC_Comm_State."Disconnect"  # Enum
        w2567 = T5 {"TCP Connection Ref"=refnum, "IP address"="", "timeout ms"=5000, "Connected?"=FALSE, "PLC Type"=enum."S7 1200", "Rack S7 400"=0, "Slot S7 400"=0, "PDU Size"=0, "connection semaphore"=refnum}  # S7 Connection out
        n789 = call <vilib>:"Clear Errors.vi"("error in (no error)"=w2568) -> ("error out"=w2571:errorcluster)  [unwired: 5 in, 1 out]
        n790 = call <vilib>:"disconnect.vi"("error in (no error)"=w2571, "S7 Connection in"=w2569) -> ("error out"=w2570:errorcluster)  [unwired: 8 in, 1 out]
      }
      frame "Write2" {
        # "SPARE"
      }
      frame "Write3" {
        # "No Use"
      }
      frame "Read2" {
        # "No Use"
      }
      frame "Read3" {
        # "No Use"
      }
    }
    n791 = Wait (ms)(milliseconds to wait=w2493) -> ()  [unwired: 1 out]
    n792 = call "PADMINI_STOP_ALL.vi"("Enum"=enum16{"Read", "Write"}."Read") -> ("Boolean 2"=w2484:bool)  [unwired: 9 in, 1 out]
    n793 = local read "stop"() -> (w2483:bool)
    n794 = case shown="Error" w2498 {
      selector: w2498 -> [w2501 w2504]
      tunnel: [w2501 w2503] -> w2478
      tunnel: [w2500 w2502] -> w2487
      tunnel: w2492 -> [w2500 _]
      tunnel: [w2499 w2510] -> w2491
      tunnel: w2490 -> [w2499 w2510]
      tunnel: w2486 -> [_ w2508]
      frame No Error {
      }
      frame Error {
        w2502 = PLC_Comm_State."Error"  # Enum
        n795 = Unbundle By Name(w2504) -> ("source"=w2509:string)
        n796 = call <userlib>:"Get Strings from Enum__ogtk.vi"("Enum"=w2508) -> ("String Value"=w2507:string)  [unwired: 7 in, 3 out]
        n797 = Concatenate Strings(w2507, "    " ("string"), w2509) -> (w2505:string)
        n798 = Bundle By Name(cluster=w2504, "source"=w2505) -> (w2503:errorcluster)
      }
    }
    n799 = Or(x=w2483, y=w2484) -> (x .or. y?=w2481:bool)
    n800 = Select(t=w2485, s=w2481, f=w2487) -> (s? t:f=w2488:T1)
    n801 = Unbundle By Name(w2478) -> ("status"=w2480:bool)
    n802 = Not(x=w2480) -> (.not. x?=w2479:bool)
    n803 = global write "Global 1.vi" "PLC 2"(w2479) -> ()
  }
  n804 = Merge Errors(w84, w3, w4, w6) -> (w80:errorcluster)
  n805 = call <vilib>:"Clear Errors.vi"("error in (no error)"=w117) -> ("error out"=w107:errorcluster)  [unwired: 5 in, 1 out]
  n806 = call <vilib>:"disconnect.vi"("error in (no error)"=w107, "S7 Connection in"=w106) -> ("error out"=w105:errorcluster)  [unwired: 8 in, 1 out]
  n807 = Merge Errors(w5, w2, w7) -> (w28:errorcluster)
  n808 = Merge Errors(w105, w80, w28) -> (w122:errorcluster)
  n809 = call <vilib>:"Simple Error Handler.vi"("type of dialog (OK msg:1)"=w10, "error in (no error)"=w122) -> ("error out"=w121:errorcluster)  [unwired: 3 in, 4 out]
  n810 = control-ref of="This VI"() -> (w11:refnum<vi>)
  n811 = call <vilib>:"Clear Errors.vi"("error in (no error)"=w121) -> ("error out"=w120:errorcluster)  [unwired: 5 in, 1 out]
  n812 = invoke class="VI" method="FP.Close"(reference=w11, error in=w120) -> (error out=→"error out":errorcluster)  [unwired: 1 in, 2 out]
